vi "MC_8_27_12d_JW.vi"() -> ()   [LabVIEW 2011]
uses:
  <vilib>/Utility/file.llb/Read From Spreadsheet File (string).vi
  <vilib>/Utility/inputDevices.llb/keyboardAcquire.vi
  <vilib>/Utility/file.llb/Write To Spreadsheet File (DBL).vi
  <vilib>/Utility/file.llb/Write To Spreadsheet File (string).vi
  <vilib>/regexp/Match Regular Expression.xnode
panel:
  in  "default (0 dbl) 6":ext format="%.2e"
  in  "default (0 dbl) 5":ext format="%.2e"
  in  "default (0 dbl) 4":ext format="%.2e"
  in  "default (0 dbl) 3":ext format="%.2e"
  in  "default (0 dbl)":ext format="%.2e"
  out "X Axis Display Type":string
  out "Opj X Axis":string
  in  "Room Temp":dbl=294.0
  out "No Image 2":path=path "\\\\acad1\\physics/Jurchescu-group/JW-PD/Image Not Found.png"
  out "Save1 Array":string[][](array[string])
  out "Lin Vd":dbl
  out "Lin-Vg Array-Used":dbl[](array[numeric])
  out "Lin Id-Used":dbl[](array[numeric])
  out "Rec: Comments":string
  out "Folder Index":dbl caption="Length"
  out "Current \nRecord":string[](array[string])
  out "Transformer \nHeaders":string[](array[string])
  out "Current Device ID":string
  out "Column":string
  out "Row":string
  out "Rec: Concentration":dbl
  out "Rec: Solvent":string
  out "Rec: Method":string
  in  "?":T1(tab)
  in  "Transport File":path
  out "Transport Folder":path
  out "Rec: Material":string
  out "Accel (RPM/s):":dbl
  in  "Transfer File":path
  out "Transfer Folder":path
  in  "Image Folder":path
  out "Image File":path=path "D:/UserData/Desktop/Jeremy/WFU/Research/Programs/VI mods/Image Not Found.png"
  in  "Manual Comments":bool
  in  "Comments:":string
  out "Calc: On/Off":dbl caption="On/Off-Sat" format="%#.2e"
  out "Calc: Off I-Sat":dbl caption="Off I-Sat" format="%#.2e"
  in  "Manuel-Dielectric":bool
  in  "Manuel-Length":bool
  out "Calc: VT-Lin":dbl
  out "New: VT-Lin":dbl
  out "Rec: VT-Lin":dbl caption="VT-Lin" format="%#_3g"
  out "Calc: Trap Density-STS":dbl format="%#.2e"
  out "New: Trap Density-STS":dbl format="%#.2e"
  out "Rec: Trap Density-STS":dbl caption="N-Sat (STS)" format="%#.2e"
  out "Calc: Trap Density-VT":dbl format="%#.2e"
  out "New: Trap Density-VT":dbl format="%#.2e"
  out "Rec: Trap Density-VT":dbl caption="N-Sat (VT)" format="%#.2e"
  out "Calc: Mobility-Lin":dbl format="%#.2e"
  out "New: Mobility-Lin":dbl format="%#_4e"
  out "Rec: Mobility-Lin":dbl caption="Mobility-Lin" format="%#_3e"
  out "Calc: Mobility-Sat":dbl format="%#.2e"
  out "Rec: Length":dbl caption="Length" format="%#_3g"
  out "Rec: Width":dbl caption="Width" format="%#_4g"
  out "Rec: Dielectric (d)":dbl caption="Dielectric (d)" format="%#_3g"
  in  "Cancel Button":bool
  in  "Up Button":bool
  in  "Down Button":bool
  out "Data Name:":string
  in  "Save Changes?":bool
  in  "New: Dielectric":dbl
  in  "New: Length":dbl
  in  "New: Width":dbl
  out "New: Mobility-Sat":dbl format="%#.2e"
  in  "Blank Button":bool
  in  "Zoom":i16(slide)=-3 scale=-5.0..5.0
  out "Image Out 2":T2(plugin-control)
  out "Image Out":T2(plugin-control)
  in  "Magnification":u16(ring) items=["5x", "10x", "20x", "50x", "80x"]
  out "Total Width":dbl
  out "Distances":dbl[](array[numeric])
  in  "Undo Button":bool
  in  "Remove Button":bool
  out "Rec: Mobility-Sat":dbl caption="Mobility-Sat" format="%#.2e"
  in  "Export":bool
  out "Calc: VT-Sat":dbl format="%#.2g"
  out "New: VT-Sat":dbl format="%#.2g"
  in  "Manual-Width":bool caption="Manual"
  out "Calc: STS":dbl format="%#.2g"
  out "New: STS":dbl format="%#.2g"
  out "Rec: VT-Sat":dbl caption="VT-Sat" format="%#.2g"
  out "Rec: STS":dbl caption="STS-Sat" format="%#.2g"
  out "Rec: On/Off":dbl caption="On/Off-Sat" format="%#.2e"
  in  "Save Changes? 2":bool
  in  "Save Changes? 3":bool
  out "Rec: Temp":dbl caption="Sample Temp" format="%.1f"
  in  "New: Temp":dbl format="%.1f"
  out "Rec: Off I-Sat":dbl caption="Off I-Sat" format="%#.2e"
  in  "Independant Variable":string(combo)="Length (um):"
  in  "Transfer Plots":T3(tab)=enum."Saturation"
  in  "Lin-Trans Slider":dbl(slide) step=1.0 scale=-22.0..89.0 scale format="%#_1p"
  out "Sqrt-Lin":cluster{dbl[], dbl[]}[](graph)
  in  "Next Sqrt Lin":bool
  in  "Previous Sqrt Lin":bool
  in  "Sat-Trans Slider":dbl(slide) step=1.0 scale=-22.0..89.0 scale format="%#_1p"
  out "Sqrt-Sat":cluster{dbl[], dbl[]}[](graph)
  in  "Previous Sqrt Sat":bool
  in  "Next Sqrt Sat":bool
  out "Raw- Lin":cluster{dbl[], dbl[]}[](graph)
  out "Raw- Sat":cluster{dbl[], dbl[]}[](graph)
  in  "Log Plots":enum32{"Linear", "Saturation", "Transport"}(tab)=enum."Saturation"
  in  "Lin-Log Slider":dbl(slide) step=1.0 scale=-1.0..82.0 scale format="%#_1p"
  in  "Previous Log Lin":bool
  in  "Next Log Lin":bool
  out "Log-Lin":cluster{dbl[], dbl[]}[](graph)
  in  "Sat-Log Slider":dbl(slide) step=1.0 scale=-1.0..82.0 scale format="%#_1p"
  in  "Previous Log Sat":bool
  in  "Next Log Sat":bool
  out "Sat-Log":cluster{dbl[], dbl[]}[](graph)
  out "Transport":cluster{dbl[], dbl[]}[](graph)
  in  "Manual-Temp":bool caption="Manual"
  out "Date Created":string caption="Fabricated"
  out "Date Recorded":string="Date Recorded" caption="Measured"
  out "Image Name":string
  out "Index":string
  in  "Num Pts":dbl=5.0
  in  "NumPoints Log":dbl=5.0 caption="Num Pts"
  in  "Ring":u16(ring) items=["Extra Small", "Small", "Medium", "Large", "Extra Large"]
  in  "Transport Line Color":u32(colorbox)
  in  "Origin Project File":path=path "\\\\acad1\\physics/Jurchescu-group/JW-PD/Group Library/Origin Project Files/DeviceData_8_10_12a_JW.opj"
  in  "No Image File":path=path "\\\\acad1\\physics/Jurchescu-group/JW-PD/Mega Awesome/Image Not Found.png"
  in  "Ramp (s):":dbl=3.0
  in  "Fabricator:":string="NaN"
  in  "Sample #:":dbl=1.0
  in  "Wait Time (s):":dbl=nan
  in  "RPM:":dbl=nan
  in  "Time (s):":dbl=nan
  in  "Room Temp (F):":dbl=nan
  in  "Relative Humidity (%):":dbl=nan
  in  "Solution Temp (C):":dbl=nan
  in  "# Drops*:":dbl=inf
  in  "Surface Treatment:":string="NaN"
  in  "Treatment Concentration (mM):":dbl=nan
  out "String":string
  out "Index 2":dbl
  out "Sat Id-Log-Used":dbl[](array[numeric])
  out "Vg Array-Log-Used":dbl[](array[numeric])
  out "ROI Descriptor out":T4 {"Contours"."Type" items=["No Selection", "Point", "Line", "Rectangle", "Oval", "Polygon", "Freehand Region", "Annulus", "Unused2", "Unused3", "Broken Line", "Freehand Line", "Rotated Rectangle"]}
  out "ROI Descriptor":T4 {"Contours"."Type" items=["No Selection", "Point", "Line", "Rectangle", "Oval", "Polygon", "Freehand Region", "Annulus", "Unused2", "Unused3", "Broken Line", "Freehand Line", "Rotated Rectangle"]}
  out "Numeric 3":dbl
  out "Array 6":dbl[][](array[numeric])
  out "Cluster":T5
  out "Array 5":dbl[](array[numeric])
  out "Array 4":dbl[](array[numeric])
  out "Array 3":dbl[](array[numeric])
  out "Numeric 2":dbl
  out "Numeric":dbl
  out "Sat Id-Used":dbl[](array[numeric])
  out "Sat Vg Array-Used":dbl[](array[numeric])
  out "MobVi Index":dbl
  in  "Row Start":dbl=20.0
  # "Data Locations"
  # "Transfer Location"
  # "Image Location"
  # "Recorded"
  # "Calculated"
  # "Re-Calculated"
  # "Manual"
  # "Used points display at y=0"
  # "Slider\nDoesn't\nWork"
  # "Slider\nDoesn't\nWork"
  # "No new points displayed"
  # "Sample Properties"
  # "*     Inf = Full coverage\n   NaN = Unknown or Not Applicable"
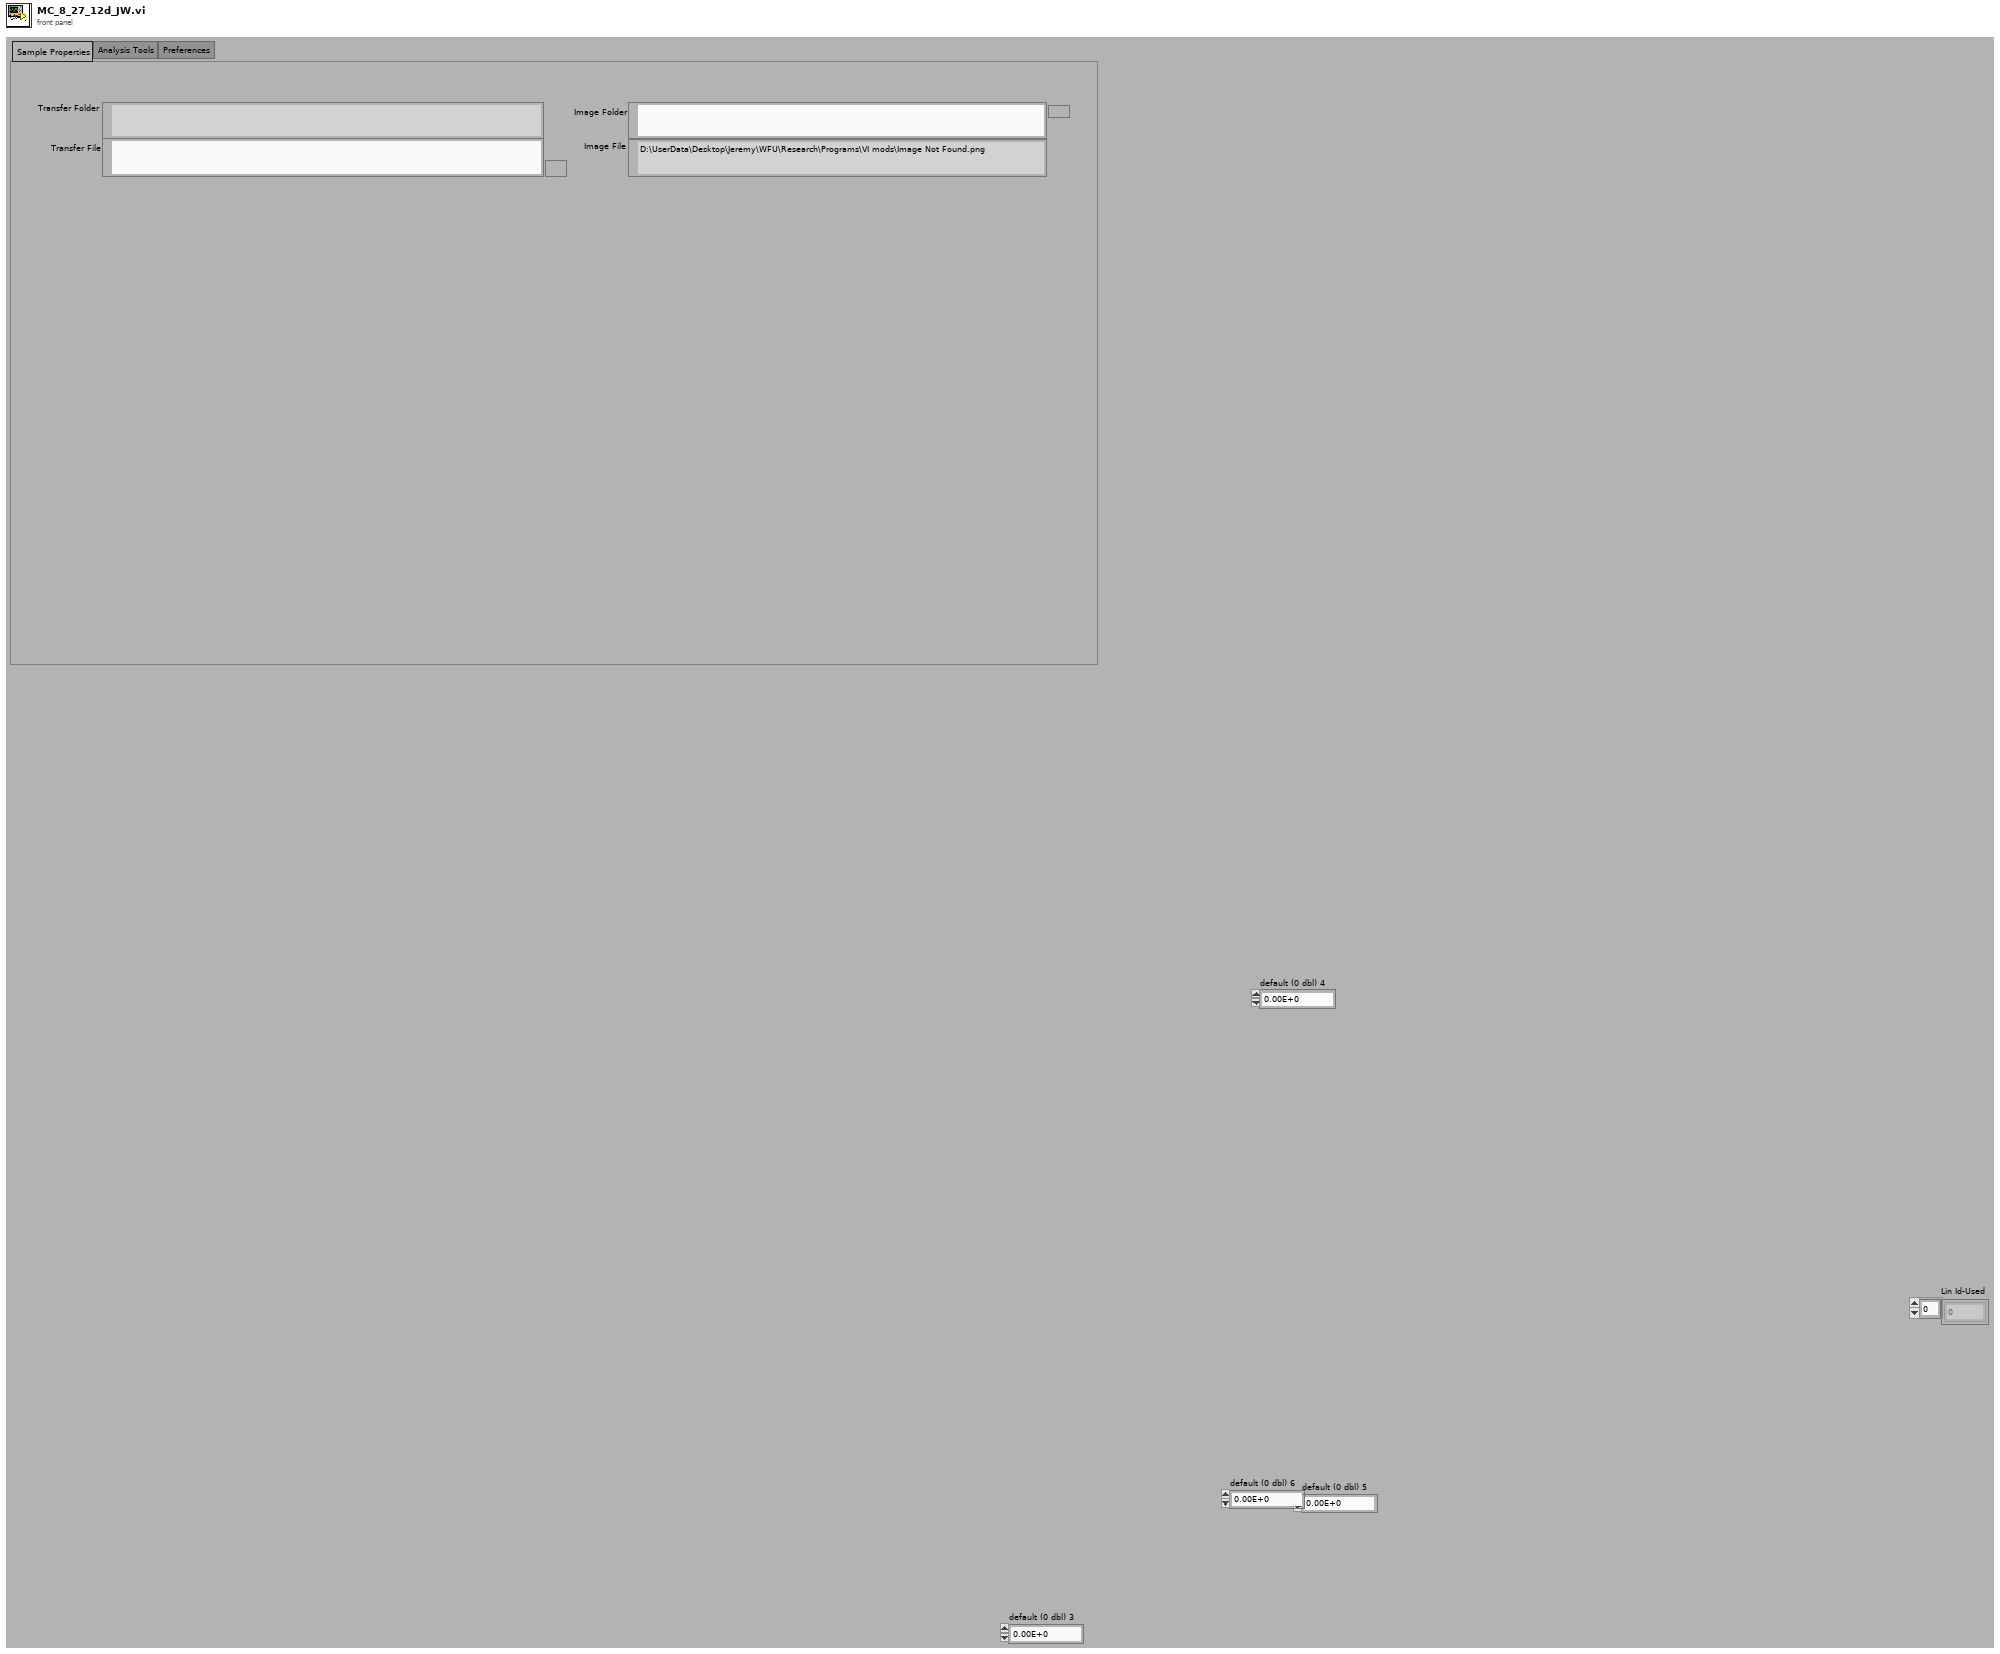
[diagram p1: front panel]
types:
  T1 = enum32{"Sample Properties", "Analysis Tools", "Preferences", "Current Database"}
  T2 = typedef "IMAQ Image.ctl" = refnum<image>
  T3 = enum32{"Linear", "Saturation", "Raw-Linear", "Raw-Saturation"}
  T4 = typedef "ROI Descriptor" = cluster{"Global Rectangle":i32[], "Contours":cluster{"ID":enum32{"External", "Internal"}, "Type":u32, "Coordinates":i32[]}[]}
  T5 = cluster{"Numeric":dbl, "Numeric 2":dbl, "Numeric 3":dbl, "Numeric 4":dbl}
  T6 = cluster{"Mobility-Sat":dbl, "Moblitity-Lin":dbl, "On/Off":dbl, "Off Current":dbl, "Vt-Sat":dbl, "STS":dbl, "Trap Density-VT":dbl, "Trap Density-STS":dbl}
  T7 = cluster{"Date Recorded":string, "Index":string, "Length":dbl, "Width":dbl, "Sample Temp":dbl}
  T8 = cluster{"Date Created":string, "Material":string, "Solvent":string, "Concentration":dbl, "Method":string, "Dielectric (nm)":dbl, "Treatment":string, "Comments":string}
  T9 = cluster{"Raw Sat":cluster{dbl[], dbl[]}[], "Sqrt Sat":cluster{dbl[], dbl[]}[], "Log Sat":cluster{dbl[], dbl[]}[], "Raw Lin":cluster{dbl[], dbl[]}[], "Sqrt Lin":cluster{dbl[], dbl[]}[], "Log Lin":cluster{dbl[], dbl[]}[]}
  T10 = cluster{"Mobility-Sat":dbl, "Vt-Sat":dbl, "Mobility-Lin":dbl, "Vt-Lin":dbl, "Off I-Sat":dbl, "On/Off I-Sat":dbl}
  T11 = cluster{"[0]":cluster{dbl[], dbl[]}, "[1]":cluster{dbl[], dbl[]}, "[2]":cluster{dbl[], dbl[]}, "[3]":cluster{dbl[], dbl[]}, "[4]":cluster{dbl[], dbl[]}, "[5]":cluster{dbl[], dbl[]}, "[6]":cluster{dbl[], dbl[]}, "[7]":cluster{dbl[], dbl[]}, "[8]":cluster{dbl[], dbl[]}}
  T12 = cluster{"Global Rectangle":i32[], "Contours":cluster{"Contour Type":u32, "ROI Type":u32, "Points":i32[]}[]}
  T13 = typedef "LVBoundsTypeDef.ctl" = cluster{"Width":u32, "Height":u32}
  T14 = enum16{"0", "1", "2", "3", "4", "5", "6", "7", "8", "9", "A", "B", "C", "D", "E", "F", "G", "H", "I", "J", "K", "L", "M", "N", "O", "P", "Q", "R", "S", "T", "U", "V", "W", "X", "Y", "Z", "F1", "F2", "F3", "F4", "F5", "F6", "F7", "F8", "F9", "F10", "F11", "F12", "F13", "F14", "F15", "ADD", "BACK", "BACKSLASH", "CAPITAL", "COMMA", "DECIMAL", "DELETE", "DIVIDE", "DOWN", "END", "EQUALS", "ESCAPE", "GRAVE (`)", "HOME", "INSERT", "LBRACKET", "LCONTROL", "LEFT", "L ALT", "LSHIFT", "LWIN", "MINUS", "MULTIPLY", "NEXT", "NUMLOCK", "NUMPAD_0", "NUMPAD_1", "NUMPAD_2", "NUMPAD_3", "NUMPAD_4", "NUMPAD_5", "NUMPAD_6", "NUMPAD_7", "NUMPAD_8", "NUMPAD_9", "PAUSE", "PERIOD", "PRIOR (PG UP)", "RBRACKET", "RCONTROL", "RETURN", "RIGHT", "R ALT", "RSHIFT", "RWIN", "SCROLL", "SEMICOLON", "SLASH", "SPACE", "SUBTRACT", "TAB", "UP", "ENTER (num pad)", "' (quote)"}[]
  T15 = enum16{"0", "1", "2", "3", "4", "5", "6", "7", "8", "9", "A", "B", "C", "D", "E", "F", "G", "H", "I", "J", "K", "L", "M", "N", "O", "P", "Q", "R", "S", "T", "U", "V", "W", "X", "Y", "Z", "F1", "F2", "F3", "F4", "F5", "F6", "F7", "F8", "F9", "F10", "F11", "F12", "F13", "F14", "F15", "ADD", "BACK", "BACKSLASH", "CAPITAL", "COMMA", "DECIMAL", "DELETE", "DIVIDE", "DOWN", "END", "EQUALS", "ESCAPE", "GRAVE (`)", "HOME", "INSERT", "LBRACKET", "LCONTROL", "LEFT", "L ALT", "LSHIFT", "LWIN", "MINUS", "MULTIPLY", "NEXT", "NUMLOCK", "NUMPAD_0", "NUMPAD_1", "NUMPAD_2", "NUMPAD_3", "NUMPAD_4", "NUMPAD_5", "NUMPAD_6", "NUMPAD_7", "NUMPAD_8", "NUMPAD_9", "PAUSE", "PERIOD", "PRIOR (PG UP)", "RBRACKET", "RCONTROL", "RETURN", "RIGHT", "R ALT", "RSHIFT", "RWIN", "SCROLL", "SEMICOLON", "SLASH", "SPACE", "SUBTRACT", "TAB", "UP", "ENTER (num pad)", "' (quote)"}
  T16 = cluster{"Contour Type":u32, "ROI Type":u32, "Points":i32[]}[]
  T17 = cluster{i32[], cluster{"Contour Type":u32, "ROI Type":u32, "Points":i32[]}[]}
  T18 = cluster{"Independant  Variable Indicator":string, "Parameter String Indicator":string}
  T19 = cluster{string, sgl, bool, bool, bool, bool, bool, bool, i32}
  T20 = cluster{i32, cluster{string, sgl, bool, bool, bool, bool, bool, bool, i32}, i32, i32}
  T21 = cluster{"Contour Type":u32, "ROI Type":u32, "Points":i32[]}
  T22 = cluster{"Points[0]":i32, "Points[1]":i32, "Points[2]":i32, "Points[3]":i32, "Points[4]":i32, "Points[5]":i32, "Points[6]":i32, "Points[7]":i32, "Points[8]":i32}
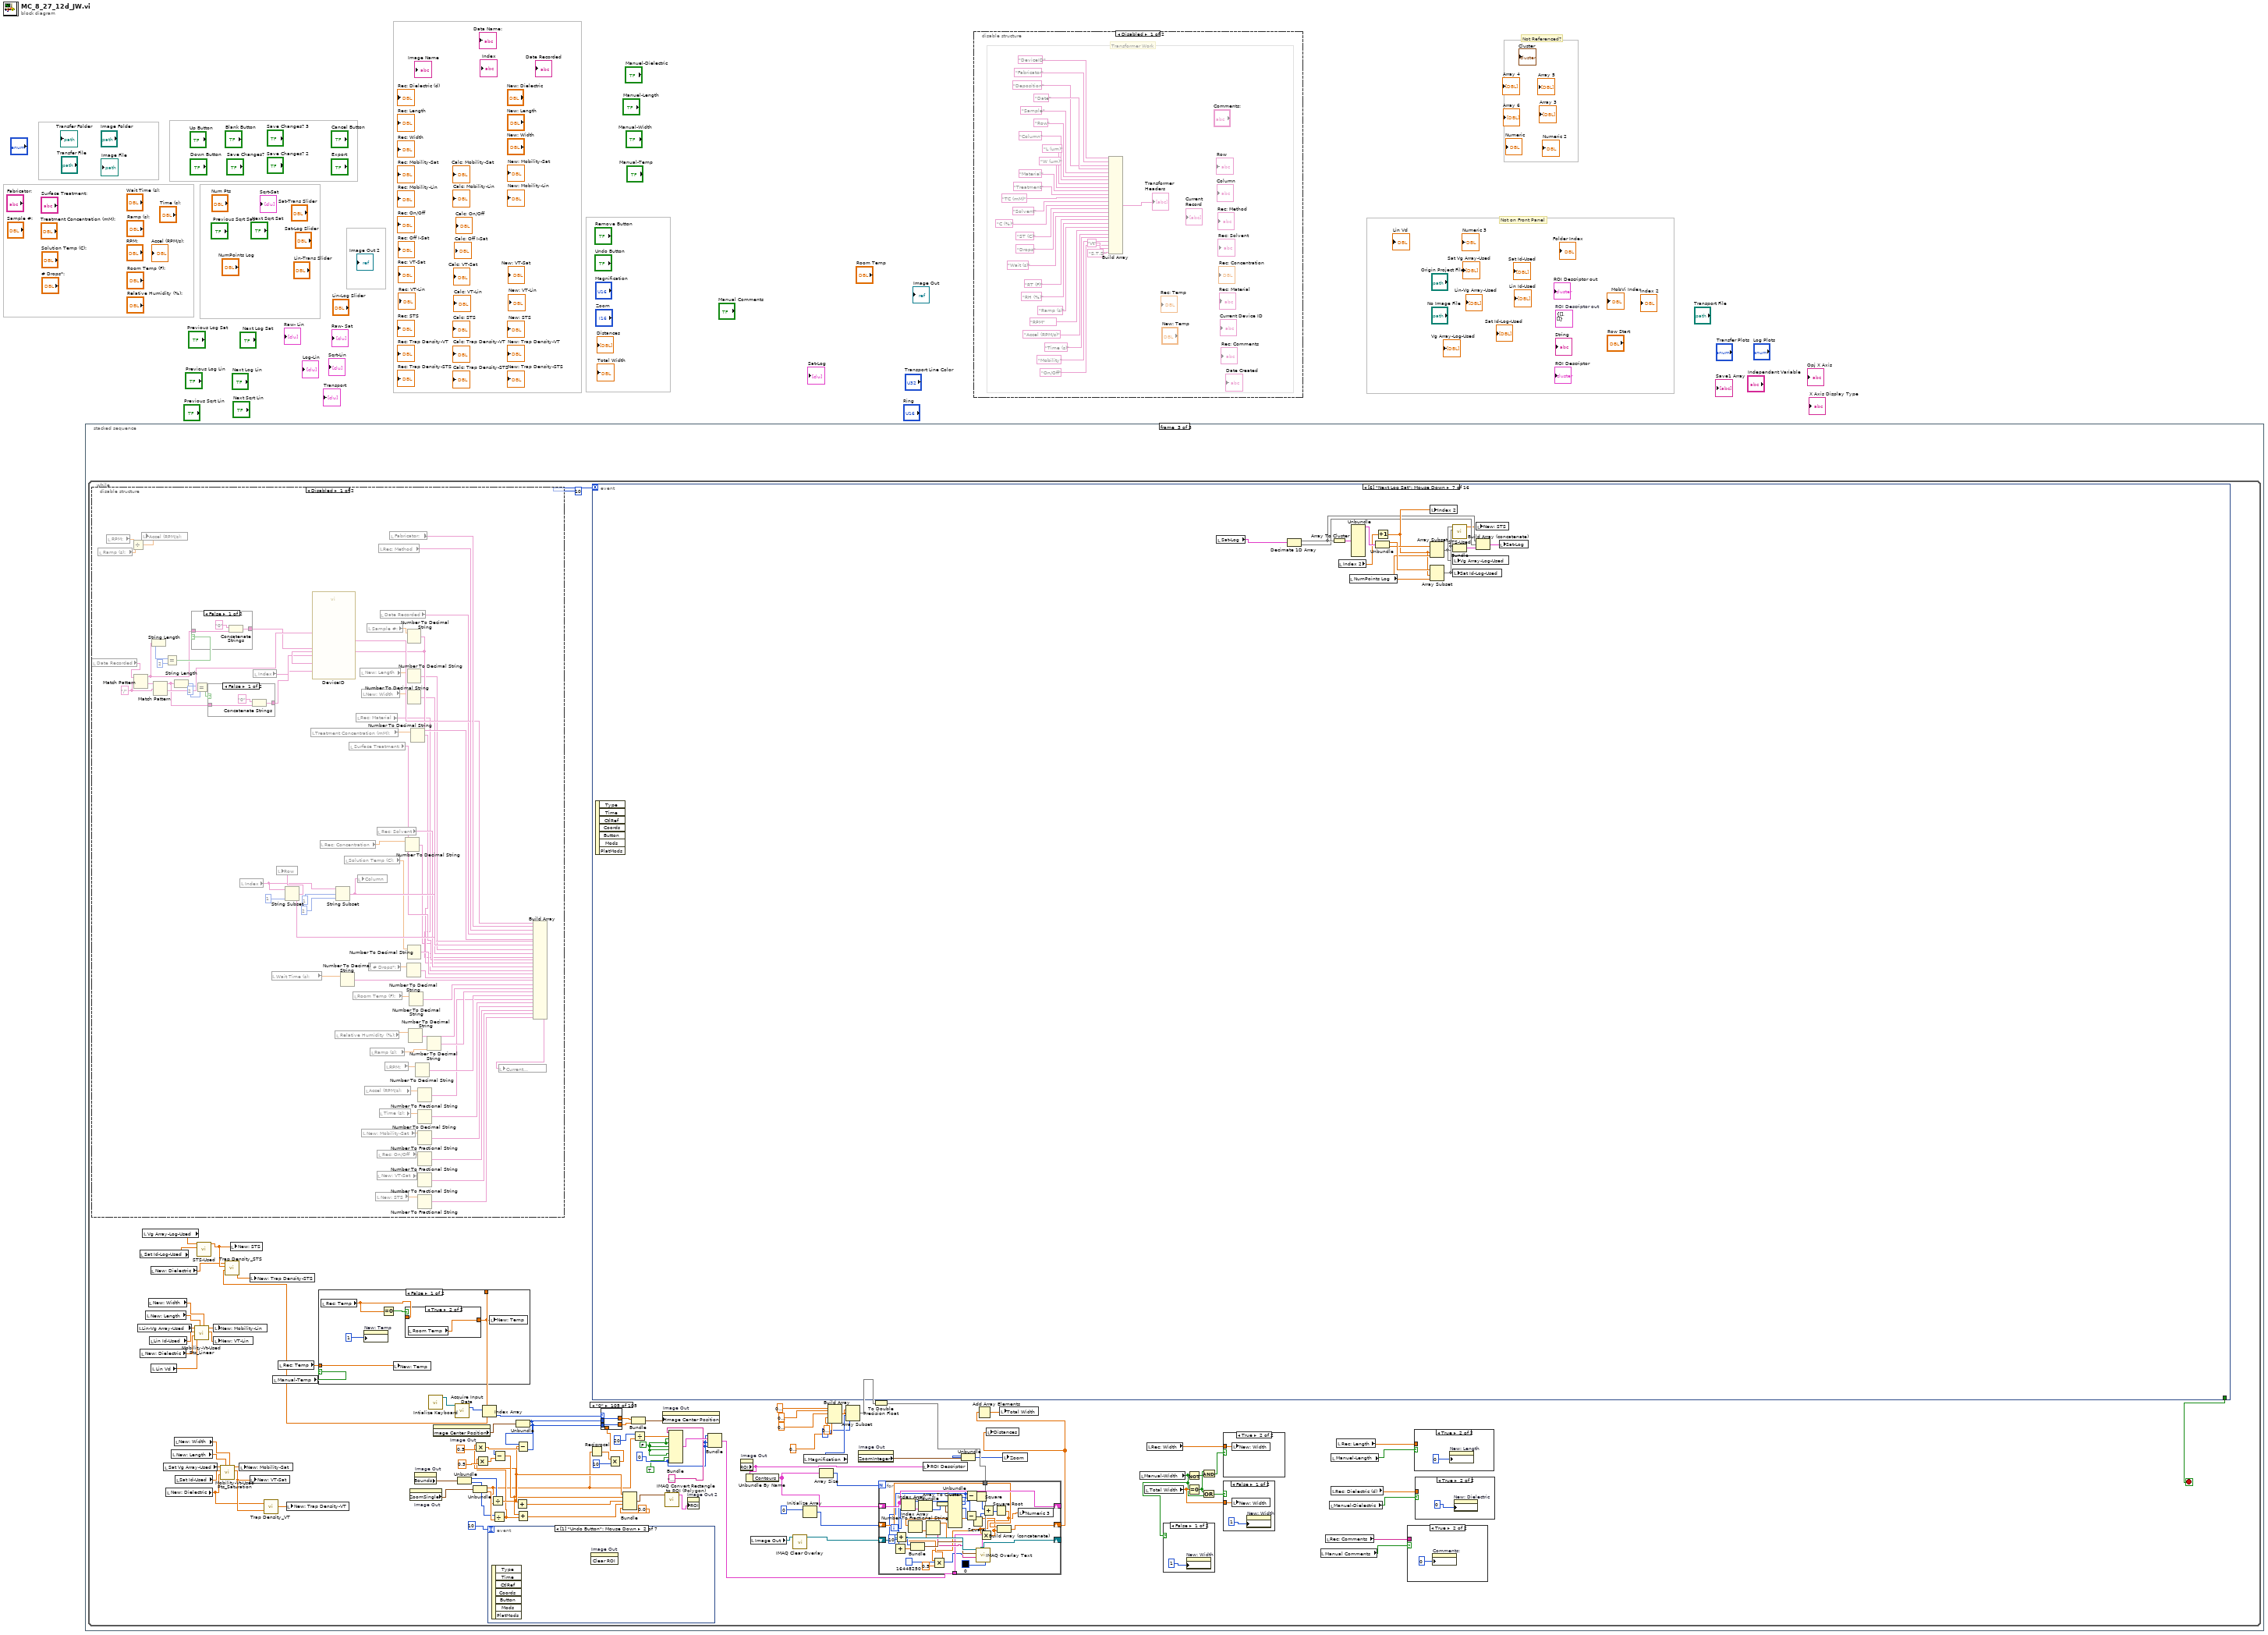
[diagram p0: block diagram]
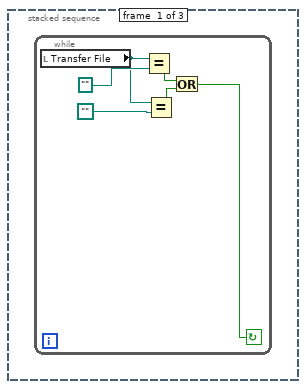
[diagram p3: hidden frame]
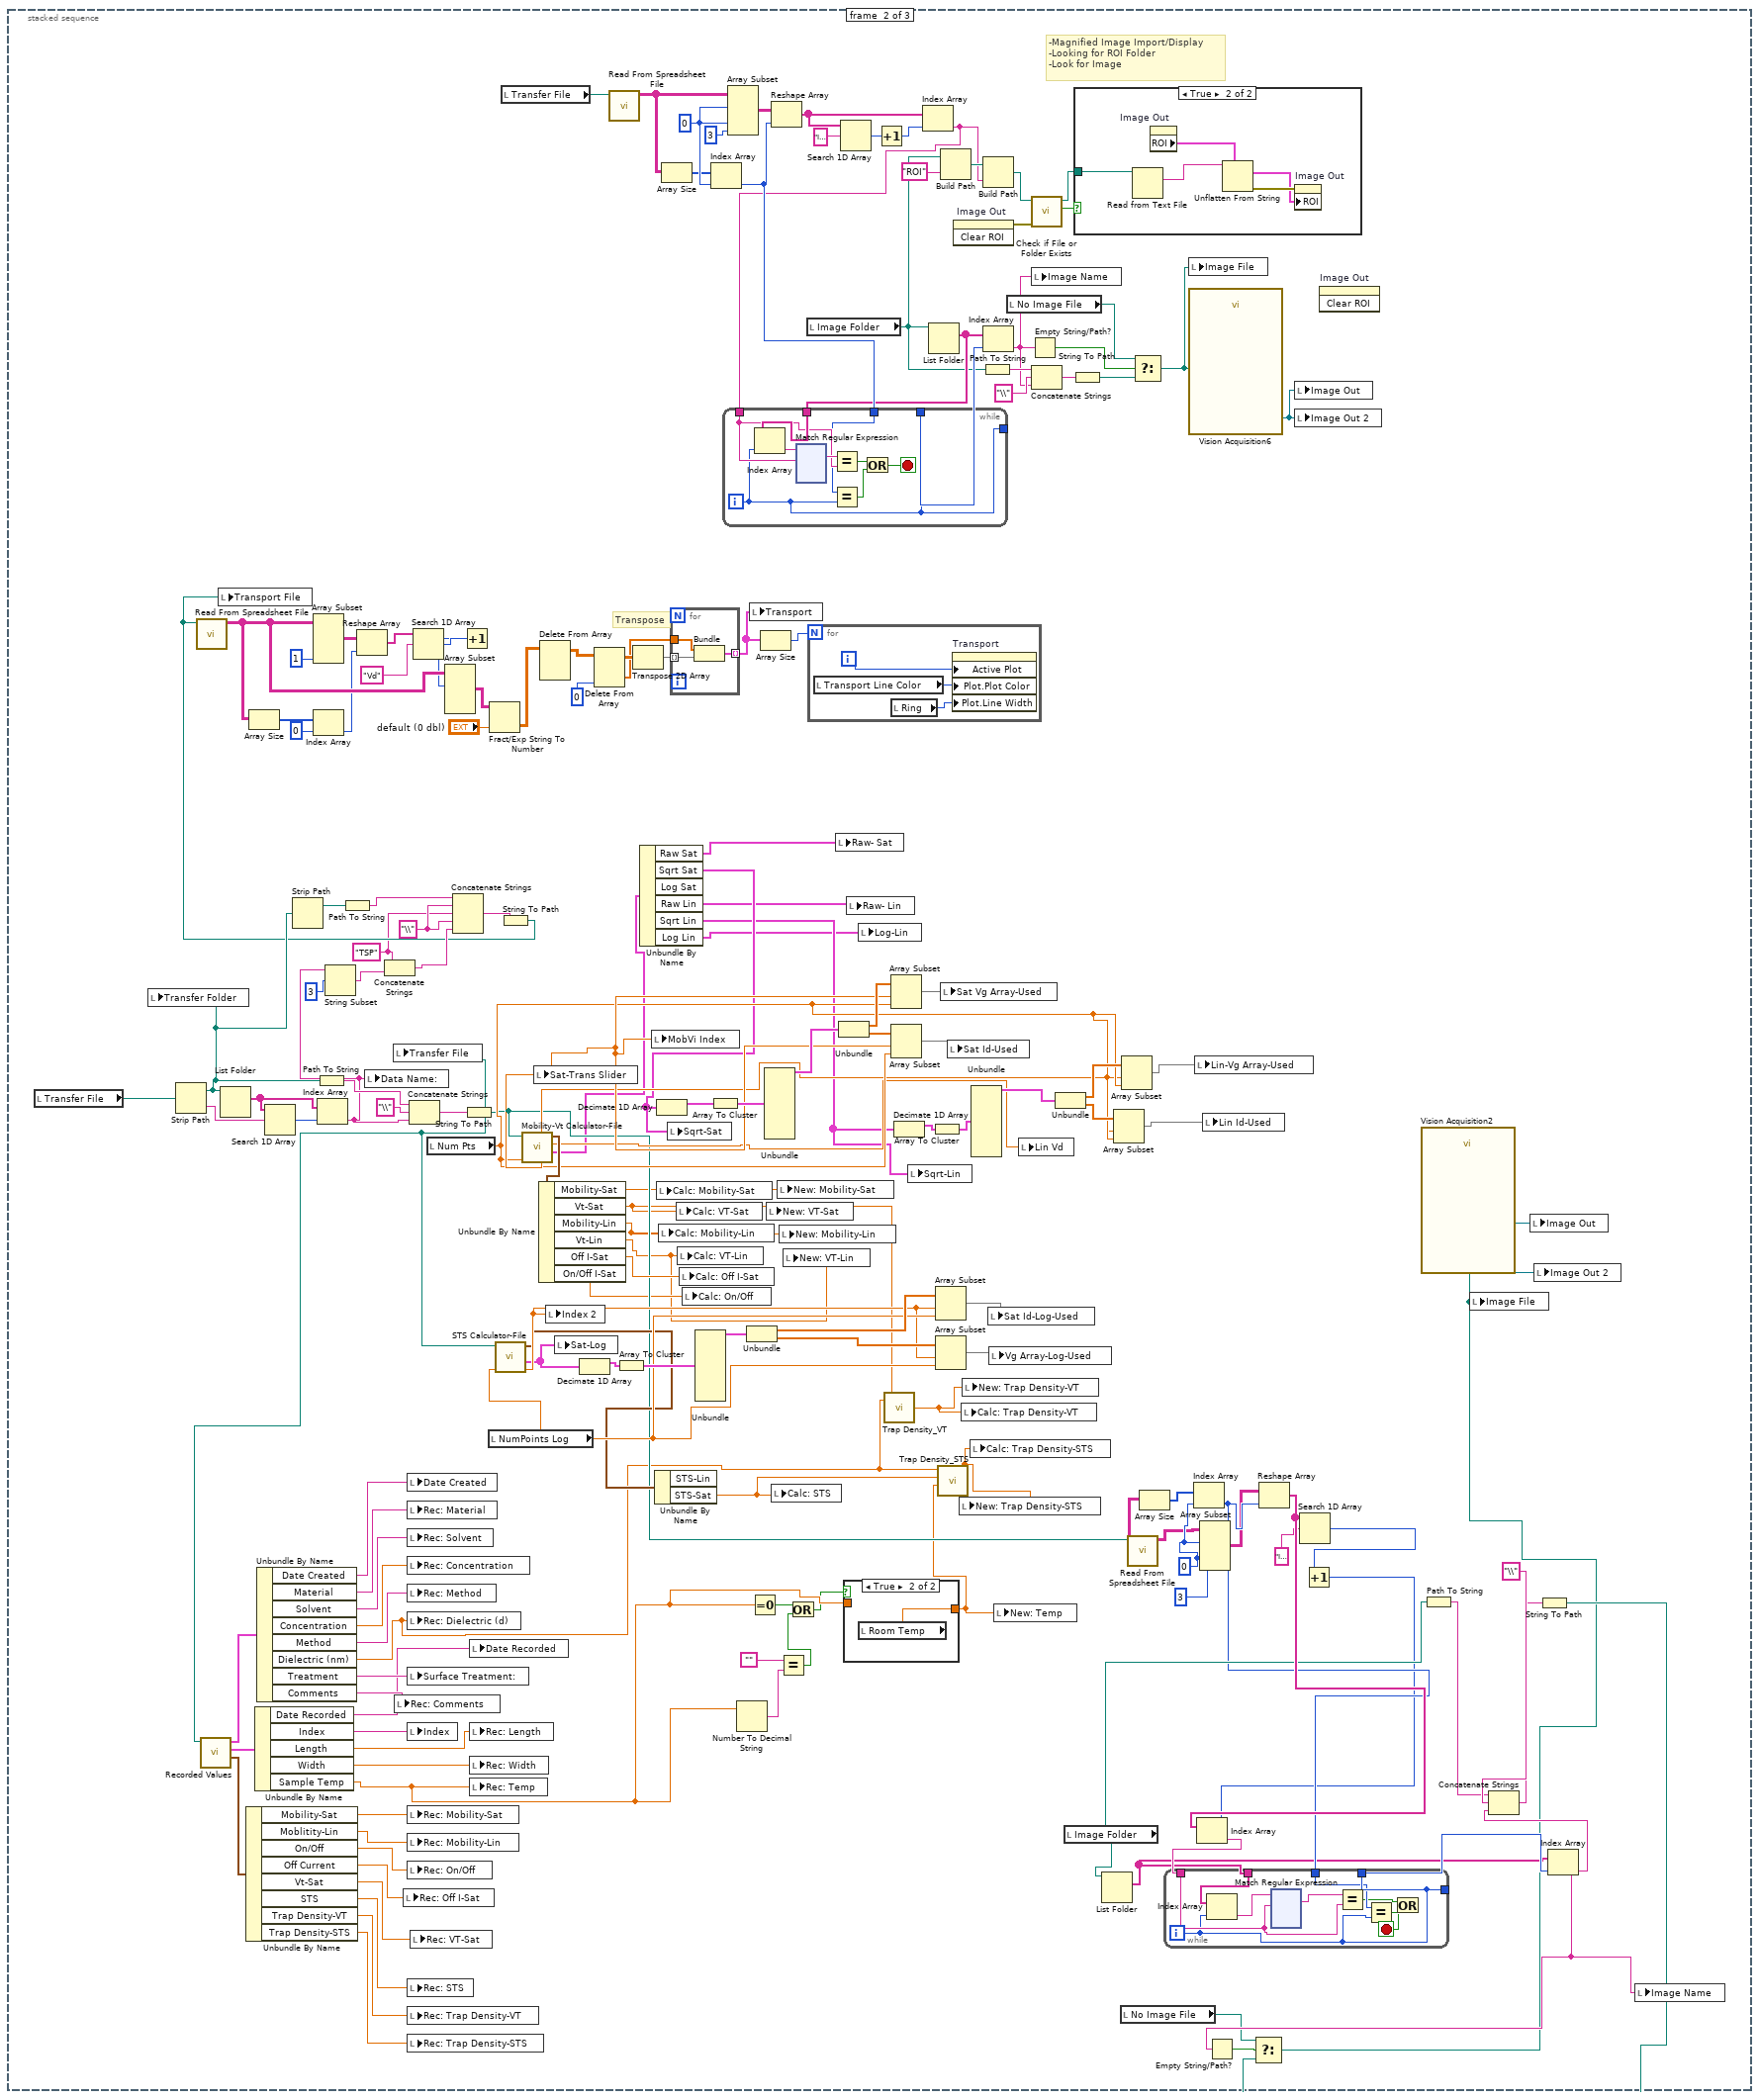
[diagram p4: hidden frame]
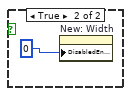
[diagram p10: hidden frame]
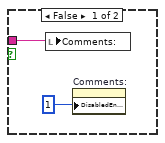
[diagram p11: hidden frame]
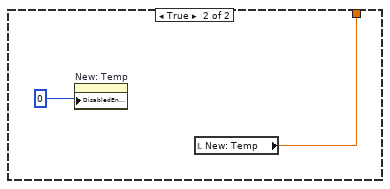
[diagram p13: hidden frame]
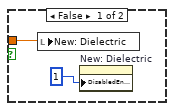
[diagram p14: hidden frame]
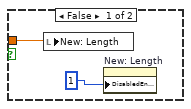
[diagram p15: hidden frame]
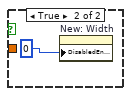
[diagram p17: hidden frame]
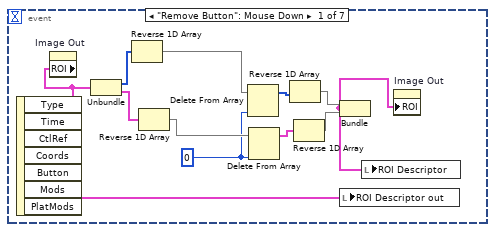
[diagram p18: hidden frame]
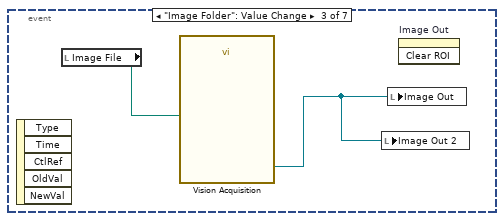
[diagram p19: hidden frame]
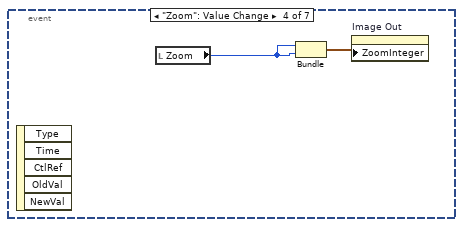
[diagram p20: hidden frame]
diagram:
  (unwired) T4 {"Global Rectangle"=[], "Contours"=[]}  # ROI Descriptor out
  # "Not Referenced?"
  # "Not on Front Panel"
  n1 = stacked-sequence {
    frame #0 {
      n2 = while {
        stop <- w1 continue-if-true
        n3 = local read "Transfer File"() -> (w3:path)
        n4 = Equal?(x=w3, y=path "") -> (x = y?=w5:bool)
        n5 = Equal?(x=w3, y=path "") -> (x = y?=w4:bool)
        n6 = Or(x=w5, y=w4) -> (x .or. y?=w1:bool)
      }
    }
    frame #1 {
      w9 = "\\"
      w8 = "TSP"
      w139 = 0
      w162 = 0
      # "Transpose"
      # "-Magnified Image Import/Display\n-Looking for ROI Folder\n-Look for Image"
      n7 = local read "Transfer File"() -> (w143:path)
      n8 = Strip Path(path=w143) -> (stripped path=w18:path, name=w130:string)
      n9 = local write "Transfer Folder"(w18) -> ()
      n10 = List Folder(path=w18) -> (filenames=w134:string[])  [unwired: 3 in, 3 out]
      n11 = Search 1D Array(1D array=w134, element=w130) -> (index of element=w133:i32)  [unwired: 1 in]
      n12 = Strip Path(path=w18) -> (stripped path=w14:path)  [unwired: 1 out]
      n13 = Path To String(path=w18) -> (string=w129:string)
      n14 = Index Array(array=w134, index=w133) -> (element=w17:string)
      n15 = String Subset(string=w17, offset (0)=3) -> (substring=w15:string)  [unwired: 1 in]
      n16 = Path To String(path=w14) -> (string=w10:string)
      n17 = local write "Data Name:"(w17) -> ()
      n18 = Concatenate Strings(w8, w15) -> (w13:string)
      n19 = Concatenate Strings(w129, "\\", w17) -> (w131:string)
      n20 = local read "Num Pts"() -> (w68:dbl)
      n21 = Concatenate Strings(w10, w9, w8, w9, w13) -> (w12:string)
      n22 = String To Path(string=w131) -> (path=w62:path)
      n23 = call "Recorded Values.vi"("Path"=w62) -> ("Recorded Char"=w98:T6, "Recorded Prop"=w97:T7, "Fabrication Prop"=w99:T8)  [unwired: 8 in]
      n24 = Unbundle By Name(w98) -> ("Mobility-Sat"=w86:dbl, "Moblitity-Lin"=w85:dbl, "On/Off"=w84:dbl, "Off Current"=w83:dbl, "Vt-Sat"=w48:dbl, "STS"=w82:dbl, "Trap Density-VT"=w81:dbl, "Trap Density-STS"=w80:dbl)
      n25 = Unbundle By Name(w97) -> ("Date Recorded"=w90:string, "Index"=w89:string, "Length"=w88:dbl, "Width"=w87:dbl, "Sample Temp"=w54:dbl)
      n26 = Unbundle By Name(w99) -> ("Date Created"=w79:string, "Material"=w96:string, "Solvent"=w95:string, "Concentration"=w94:dbl, "Method"=w93:string, "Dielectric (nm)"=w58:dbl, "Treatment"=w92:string, "Comments"=w91:string)
      n27 = local write "Transfer File"(w62) -> ()
      n28 = local write "Rec: Comments"(w91) -> ()
      n29 = local write "Rec: Off I-Sat"(w83) -> ()
      n30 = local write "Date Created"(w79) -> ()
      n31 = local write "Rec: Material"(w96) -> ()
      n32 = local write "Rec: Solvent"(w95) -> ()
      n33 = local write "Rec: Concentration"(w94) -> ()
      n34 = local write "Rec: Method"(w93) -> ()
      n35 = local write "Rec: Dielectric (d)"(w58) -> ()
      n36 = local write "Surface Treatment:"(w92) -> ()
      n37 = local write "Index"(w89) -> ()
      n38 = local write "Rec: Mobility-Sat"(w86) -> ()
      n39 = local write "Rec: Mobility-Lin"(w85) -> ()
      n40 = local write "Rec: On/Off"(w84) -> ()
      n41 = local write "Rec: STS"(w82) -> ()
      n42 = local write "Rec: Trap Density-VT"(w81) -> ()
      n43 = local write "Rec: Trap Density-STS"(w80) -> ()
      n44 = local write "Rec: VT-Sat"(w48) -> ()
      n45 = local write "Date Recorded"(w90) -> ()
      n46 = local write "Rec: Length"(w88) -> ()
      n47 = local write "Rec: Width"(w87) -> ()
      n48 = local write "Rec: Temp"(w54) -> ()
      n49 = local read "NumPoints Log"() -> (w76:dbl)
      n50 = call "STS Calculator-File.vi"("NumPts"=w76, "Path"=w62) -> ("STS Index-Sat"=w75:dbl, "XY Graph-Sat"=w7:cluster{dbl[], dbl[]}[], "Ouput"=w74:cluster{"STS-Sat":dbl, "STS-Lin":dbl})  [unwired: 5 in, 2 out]
      n51 = String To Path(string=w12) -> (path=w11:path)
      n52 = call-poly <vilib>:"Read From Spreadsheet File.vi"("file path (dialog if empty)"=w11) -> ("all rows"=w32:string[][])  [unwired: 6 in, 4 out]
      n53 = local write "Transport File"(w11) -> ()
      n54 = Array Size(array=w32) -> (size(s)=w38:i32[])
      n55 = Array Subset(array=w32, length (col)=1) -> (w34:string[][])  [unwired: 3 in]
      n56 = Index Array(array=w38, index=0) -> (element=w27:i32)
      n57 = Reshape Array(w34, w27) -> (w33:string[])
      n58 = Search 1D Array(1D array=w33, element="Vd") -> (index of element=w31:i32)  [unwired: 1 in]
      n59 = Increment(x=w31) -> (x+1=w30:i32)
      n60 = Array Subset(array=w32, index (row)=w30) -> (w28:string[][])  [unwired: 3 in]
      n61 = Fract/Exp String To Number(string=w28, default (0 dbl)="default (0 dbl)") -> (number=w20:ext[][])  [unwired: 2 in, 1 out]
      n62 = local read "Transfer File"() -> (w157:path)
      n63 = call "Mobility-Vt Calculator-File.vi"("NumPts"=w68, "Path"=w62) -> ("Graph Cluster"=w39:T9, "Lin Vd"=w64:dbl, "Output"=w78:T10, "Index-Sat"=w77:dbl, "Index-Lin"=w67:dbl)  [unwired: 5 in]
      n64 = local write "Sat-Trans Slider"(w77) -> ()
      n65 = Unbundle By Name(w78) -> ("Mobility-Sat"=w57:dbl, "Vt-Sat"=w56:dbl, "Mobility-Lin"=w47:dbl, "Vt-Lin"=w45:dbl, "Off I-Sat"=w63:dbl, "On/Off I-Sat"=w46:dbl)
      n66 = Delete From Array(array=w20) -> (array with subset deleted=w19:ext[][])  [unwired: 3 in, 1 out]
      n67 = local write "Index 2"(w75) -> ()
      n68 = local write "Sat-Log"(w7) -> ()
      n69 = Decimate 1D Array(w7) -> (w121:cluster{dbl[], dbl[]}[])  [unwired: 1 out]
      n70 = Delete From Array(array=w19, index (col)=0 ("Deaktivierter Index (Spalte)")) -> (deleted portion=w24:ext[], array with subset deleted=w25:ext[][])  [unwired: 2 in]
      n71 = call-poly <vilib>:"Read From Spreadsheet File.vi"("file path (dialog if empty)"=w157) -> ("all rows"=w160:string[][])  [unwired: 6 in, 4 out]
      n72 = Array To Cluster(array=w121) -> (cluster=w123:T11)
      n73 = Transpose 2D Array(2D array=w25) -> (transposed array=w26:ext[][])
      n74 = Unbundle By Name(w39) -> ("Raw Sat"=w42:cluster{dbl[], dbl[]}[], "Sqrt Sat"=w44:cluster{dbl[], dbl[]}[], "Raw Lin"=w41:cluster{dbl[], dbl[]}[], "Sqrt Lin"=w43:cluster{dbl[], dbl[]}[], "Log Lin"=w40:cluster{dbl[], dbl[]}[])  [unwired: 1 out]
      n75 = local write "MobVi Index"(w77) -> ()
      n76 = Unbundle By Name(w74) -> ("STS-Sat"=w61:dbl)  [unwired: 1 out]
      n77 = Decimate 1D Array(w44) -> (w156:cluster{dbl[], dbl[]}[])  [unwired: 1 out]
      n78 = local write "Calc: Mobility-Sat"(w57) -> ()
      n79 = local write "Calc: Mobility-Lin"(w47) -> ()
      n80 = Array Size(array=w160) -> (size(s)=w161:i32[])
      n81 = local write "Sqrt-Sat"(w44) -> ()
      n82 = for {
        tunnel: w24 -> [w178]
        tunnel: w26 -> [w179] mode=indexing
        tunnel: [w177] -> w22 mode=indexing
        n83 = Bundle(w178, w179) -> (w177:cluster{ext[], ext[]})  [unwired: 1 in]
      }
      n84 = local write "Calc: VT-Sat"(w56) -> ()
      n85 = local write "Calc: VT-Lin"(w45) -> ()
      n86 = local write "Calc: Off I-Sat"(w63) -> ()
      n87 = local write "Calc: On/Off"(w46) -> ()
      n88 = Unbundle(w123) -> ("[0]"=w122:cluster{dbl[], dbl[]})  [unwired: 8 out]
      n89 = Array To Cluster(array=w156) -> (cluster=w154:T11)
      n90 = Index Array(array=w161, index=w162) -> (element=w168:i32)
      n91 = Array Subset(array=w160, index (row)=w162, index (col)=w162, length (col)=3) -> (w159:string[][])  [unwired: 1 in]
      n92 = Number To Decimal String(number=w54) -> (decimal integer string=w52:string)  [unwired: 1 in]
      n93 = Unbundle(w122) -> (w119:dbl[], w118:dbl[])
      n94 = local write "Transport"(w22) -> ()
      n95 = Equal To 0?(x=w54) -> (x = 0?=w53:bool)
      n96 = Array Size(array=w22) -> (size(s)=w21:i32)
      n97 = Unbundle(w154) -> ("[0]"=w155:cluster{dbl[], dbl[]})  [unwired: 8 out]
      n98 = local write "New: VT-Sat"(w56) -> ()
      n99 = Reshape Array(w159, w168) -> (w173:string[])
      n100 = local write "Calc: STS"(w61) -> ()
      n101 = local write "New: Mobility-Sat"(w57) -> ()
      n102 = Equal?(x="", y=w52) -> (x = y?=w50:bool)
      n103 = local write "New: Mobility-Lin"(w47) -> ()
      n104 = local write "New: VT-Lin"(w45) -> ()
      n105 = Or(x=w53, y=w50) -> (x .or. y?=w49:bool)
      n106 = local read "Image Folder"() -> (w100:path)
      n107 = for {
        N: w21 -> [_]
        i -> [w176]
        n108 = local read "Transport Line Color"() -> (w175:u32)
        n109 = local read "Ring"() -> (w174:u16)
        n110 = property on="Transport" class="XYGraph (strict)"("Active Plot"=w176, "Plot.Plot Color"=w175, "Plot.Line Width"=w174) -> ()  [unwired: 2 in, 2 out]
      }
      n111 = local write "Raw- Sat"(w42) -> ()
      n112 = Unbundle(w155) -> (w120:dbl[], w124:dbl[])
      n113 = Search 1D Array(1D array=w173, element="Index:") -> (index of element=w165:i32)  [unwired: 1 in]
      n114 = case shown="True" w49 {
        tunnel: [w180 w181] -> w60
        tunnel: w54 -> [w180 _]
        frame False {
        }
        frame True {
          n115 = local read "Room Temp"() -> (w181:dbl)
        }
      }
      n116 = local write "Raw- Lin"(w41) -> ()
      n117 = local write "Log-Lin"(w40) -> ()
      n118 = Increment(x=w165) -> (x+1=w164:i32)
      n119 = call "Trap Density_VT.vi"("VT"=w56, "Dielectric"=w58) -> ("Trap Density-VT"=w55:dbl)
      n120 = Array Subset(array=w120, index=w77, length=w68) -> (w127:dbl[])
      n121 = Array Subset(array=w124, index=w77, length=w68) -> (w128:dbl[])
      n122 = Decimate 1D Array(w43) -> (w73:cluster{dbl[], dbl[]}[])  [unwired: 1 out]
      n123 = local write "Sqrt-Lin"(w43) -> ()
      n124 = Index Array(array=w173, index=w164) -> (element=w101:string)
      n125 = List Folder(path=w100) -> (filenames=w166:string[])  [unwired: 3 in, 3 out]
      n126 = while {
        tunnel: w166 -> [w314]
        tunnel: w101 -> [w312]
        tunnel: [w311] -> _
        tunnel: [w311] -> w167
        tunnel: w168 -> [w310]
        i -> [w311]
        stop <- w307 stop-if-true
        n127 = Index Array(array=w314, index=w311) -> (element=w315:string)
        n128 = xnode "Match Regular Expression"("input string"=w315, "regular expression"=w312) -> ("whole match"=w313:string)  [unwired: 4 in, 4 out]
        n129 = Equal?(x=w313, y=w312) -> (x = y?=w309:bool)
        n130 = Equal?(x=w310, y=w311) -> (x = y?=w308:bool)
        n131 = Or(x=w309, y=w308) -> (x .or. y?=w307:bool)
      }
      n132 = Array To Cluster(array=w73) -> (cluster=w72:T11)
      n133 = Array Subset(array=w119, index=w75, length=w76) -> (w126:dbl[])
      n134 = Array Subset(array=w118, index=w75, length=w76) -> (w125:dbl[])
      n135 = call "Trap Density_STS.vi"("Temp (T) [K]"=w60, "S.T.S. (S)"=w61, "Dielectric"=w58) -> ("Trap Density (N)"=w59:dbl)  [unwired: 8 in]
      n136 = Build Path(base path=w100, name or relative path="ROI") -> (appended path=w103:path)
      n137 = local write "Sat Vg Array-Used"(w127) -> ()
      n138 = local write "Sat Id-Used"(w128) -> ()
      n139 = invoke on="Image Out" class="ImageControl" method="Clear ROI"() -> (error out=w107:errorcluster)  [unwired: 3 in, 2 out]
      n140 = local write "New: Trap Density-STS"(w59) -> ()
      n141 = local write "Calc: Trap Density-VT"(w55) -> ()
      n142 = local write "New: Trap Density-VT"(w55) -> ()
      n143 = local write "Calc: Trap Density-STS"(w59) -> ()
      n144 = Unbundle(w72) -> ("[0]"=w71:cluster{dbl[], dbl[]})  [unwired: 8 out]
      n145 = Path To String(path=w100) -> (string=w170:string)
      n146 = Build Path(base path=w103, name or relative path=w101) -> (appended path=w102:path)
      n147 = Index Array(array=w166, index=w167) -> (element=w117:string)
      n148 = local write "Sat Id-Log-Used"(w126) -> ()
      n149 = local write "Vg Array-Log-Used"(w125) -> ()
      n150 = local write "New: Temp"(w60) -> ()
      n151 = local read "No Image File"() -> (w108:path)
      n152 = local write "Lin Vd"(w64) -> ()
      n153 = Empty String/Path?(string/path=w117) -> (empty?=w116:bool)
      n154 = call <vilib>:"Check if File or Folder Exists.vi"("error in (no error)"=w107, "path"=w102) -> ("file or folder exists?"=w105:bool, "dup path"=w106:path)  [unwired: 7 in, 1 out]
      n155 = local write "Image Name"(w117) -> ()
      n156 = Concatenate Strings(w170, "\\", w117) -> (w171:string)
      n157 = Unbundle(w71) -> (w70:dbl[], w69:dbl[])
      n158 = local read "Image Folder"() -> (w149:path)
      n159 = String To Path(string=w171) -> (path=w115:path)
      n160 = case shown="True" w105 {
        tunnel: w106 -> [_ w182]
        frame False {
        }
        frame True {
          n161 = Read from Text File(file (use dialog)=w182) -> (text=w186:string)  [unwired: 3 in, 3 out]
          n162 = property on="Image Out" class="ImageControl"() -> ("ROI"=w183:T12)  [unwired: 2 in, 2 out]
          n163 = Unflatten From String(type=w183, binary string=w186) -> (value=w184:T12, error out=w185:errorcluster)  [unwired: 3 in, 1 out]
          n164 = property on="Image Out" class="ImageControl"(error in=w185, "ROI"=w184) -> ()  [unwired: 1 in, 2 out]
        }
      }
      n165 = List Folder(path=w149) -> (filenames=w145:string[])  [unwired: 3 in, 3 out]
      n166 = Array Subset(array=w69, index=w67, length=w68) -> (w65:dbl[])
      n167 = local read "No Image File"() -> (w109:path)
      n168 = Array Subset(array=w70, index=w67, length=w68) -> (w66:dbl[])
      n169 = call-poly <vilib>:"Read From Spreadsheet File.vi"("file path (dialog if empty)"=w62) -> ("all rows"=w137:string[][])  [unwired: 6 in, 4 out]
      n170 = Select(t=w108, s=w116, f=w115) -> (s? t:f=w114:path)
      n171 = Array Size(array=w137) -> (size(s)=w138:i32[])
      n172 = local write "Image File"(w114) -> ()
      n173 = call "Vision Acquisition6"("Image Path"=w114) -> ("Image Out"=w169:T2)  [unwired: 25 in, 1 out]
      n174 = Index Array(array=w138, index=w139) -> (element=w148:i32)
      n175 = local write "Lin-Vg Array-Used"(w66) -> ()
      n176 = Array Subset(array=w137, index (row)=w139, index (col)=w139, length (col)=3) -> (w136:string[][])  [unwired: 1 in]
      n177 = local write "Lin Id-Used"(w65) -> ()
      n178 = Reshape Array(w136, w148) -> (w153:string[])
      n179 = local write "Image Out"(w169) -> ()
      n180 = local write "Image Out 2"(w169) -> ()
      n181 = Search 1D Array(1D array=w153, element="Index:") -> (index of element=w142:i32)  [unwired: 1 in]
      n182 = Increment(x=w142) -> (x+1=w141:i32)
      n183 = Index Array(array=w153, index=w141) -> (element=w146:string)
      n184 = while {
        tunnel: w145 -> [w194]
        tunnel: w146 -> [w192]
        tunnel: [w191] -> _
        tunnel: [w191] -> w147
        tunnel: w148 -> [w190]
        i -> [w191]
        stop <- w187 stop-if-true
        n185 = Index Array(array=w194, index=w191) -> (element=w195:string)
        n186 = xnode "Match Regular Expression"("input string"=w195, "regular expression"=w192) -> ("whole match"=w193:string)  [unwired: 4 in, 4 out]
        n187 = Equal?(x=w193, y=w192) -> (x = y?=w189:bool)
        n188 = Equal?(x=w190, y=w191) -> (x = y?=w188:bool)
        n189 = Or(x=w189, y=w188) -> (x .or. y?=w187:bool)
      }
      n190 = invoke on="Image Out" class="ImageControl" method="Clear ROI"() -> ()  [unwired: 3 in, 3 out]
      n191 = Path To String(path=w149) -> (string=w150:string)
      n192 = Index Array(array=w145, index=w147) -> (element=w112:string)
      n193 = Empty String/Path?(string/path=w112) -> (empty?=w113:bool)
      n194 = Concatenate Strings(w150, "\\", w112) -> (w151:string)
      n195 = String To Path(string=w151) -> (path=w111:path)
      n196 = Select(t=w109, s=w113, f=w111) -> (s? t:f=w110:path)
      n197 = call "Vision Acquisition2"("Image Path"=w110) -> ("Image Out"=w144:T2)  [unwired: 25 in, 1 out]
      n198 = local write "Image File"(w110) -> ()
      n199 = local write "Image Out"(w144) -> ()
      n200 = local write "Image Out 2"(w144) -> ()
      n201 = local write "Image Name"(w112) -> ()
    }
    frame #2 {
      n202 = while {
        stop <- w526 stop-if-true
        w476 = FALSE
        w474 = 0
        n203 = disable-structure shown="Disabled" {
          frame Disabled {
            w560 = "/"
            n204 = local read "Date Recorded"() -> (w563:string)
            n205 = local read "Ramp (s):"() -> (w530:dbl)
            n206 = local read "RPM:"() -> (w531:dbl)
            n207 = Divide(x=w531, y=w530) -> (x/y=w529:dbl)
            n208 = Match Pattern(string=w563, regular expression=w560) -> (before substring=w554:string, after substring=w561:string)  [unwired: 1 in, 2 out]
            n209 = local write "Accel (RPM/s):"(w529) -> ()
            n210 = String Length(string=w554) -> (length=w557:i32)
            n211 = Match Pattern(string=w561, regular expression=w560) -> (before substring=w548:string, after substring=w559:string)  [unwired: 1 in, 2 out]
            n212 = Equal?(x=w557, y=2) -> (x = y?=w555:bool)
            n213 = String Length(string=w548) -> (length=w550:i32)
            n214 = case shown="False" w555 {
              tunnel: w554 -> [w600 w602]
              tunnel: [w599 w602] -> w553
              frame False {
                n215 = Concatenate Strings("0", w600) -> (w599:string)
              }
              frame True {
              }
            }
            n216 = Equal?(x=w550, y=2) -> (x = y?=w552:bool)
            n217 = case shown="False" w552 {
              tunnel: w548 -> [w596 w598]
              tunnel: [w595 w598] -> w549
              frame False {
                n218 = Concatenate Strings("0", w596) -> (w595:string)
              }
              frame True {
              }
            }
            n219 = local read "Index"() -> (w533:string)
            n220 = local read "Index"() -> (w547:string)
            n221 = local read "Wait Time (s):"() -> (w593:dbl)
            n222 = String Subset(string=w533, length (rest)=1) -> (substring=w588:string)  [unwired: 1 in]
            n223 = local write "Row"(w588) -> ()
            n224 = local read "Treatment Concentration (mM):"() -> (w541:dbl)
            n225 = local read "Rec: Concentration"() -> (w528:dbl)
            n226 = local read "Relative Humidity (%):"() -> (w538:dbl)
            n227 = String Subset(string=w533, offset (0)=1, length (rest)=2) -> (substring=w589:string)
            n228 = Number To Decimal String(number=w593) -> (decimal integer string=w594:string)  [unwired: 1 in]
            n229 = local read "Solution Temp (C):"() -> (w582:dbl)
            n230 = local read "Surface Treatment:"() -> (w540:string)
            n231 = local read "Room Temp (F):"() -> (w586:dbl)
            n232 = local read "Rec: Material"() -> (w536:string)
            n233 = local write "Column"(w589) -> ()
            n234 = local read "New: Length"() -> (w546:dbl)
            n235 = local read "New: Width"() -> (w545:dbl)
            n236 = local read "New: Mobility-Sat"() -> (w575:dbl)
            n237 = local read "Accel (RPM/s):"() -> (w573:dbl)
            n238 = local read "Sample #:"() -> (w565:dbl)
            n239 = local read "# Drops*:"() -> (w583:dbl)
            n240 = local read "Ramp (s):"() -> (w591:dbl)
            n241 = local read "New: STS"() -> (w567:dbl)
            n242 = local read "Rec: Solvent"() -> (w542:string)
            n243 = local read "New: VT-Sat"() -> (w569:dbl)
            n244 = local read "Rec: On/Off"() -> (w571:dbl)
            n245 = local read "Rec: Method"() -> (w566:string)
            n246 = local read "Time (s):"() -> (w578:dbl)
            n247 = local read "Date Recorded"() -> (w562:string)
            n248 = local read "RPM:"() -> (w579:dbl)
            n249 = local read "Fabricator:"() -> (w587:string)
            n250 = Number To Decimal String(number=w528) -> (decimal integer string=w527:string)  [unwired: 1 in]
            n251 = Number To Decimal String(number=w583) -> (decimal integer string=w584:string)  [unwired: 1 in]
            n252 = Number To Decimal String(number=w565) -> (decimal integer string=w558:string)  [unwired: 1 in]
            n253 = call "DeviceID"("Sample"=w558, "Year"=w559, "Month"=w553, "Day"=w549, "Index"=w547) -> ("Result"=w564:string)  [unwired: 9 in, 1 out]
            n254 = Number To Decimal String(number=w546) -> (decimal integer string=w544:string)  [unwired: 1 in]
            n255 = Number To Decimal String(number=w545) -> (decimal integer string=w543:string)  [unwired: 1 in]
            n256 = Number To Decimal String(number=w582) -> (decimal integer string=w581:string)  [unwired: 1 in]
            n257 = Number To Decimal String(number=w538) -> (decimal integer string=w537:string)  [unwired: 1 in]
            n258 = Number To Decimal String(number=w586) -> (decimal integer string=w585:string)  [unwired: 1 in]
            n259 = Number To Decimal String(number=w541) -> (decimal integer string=w539:string)  [unwired: 1 in]
            n260 = Number To Decimal String(number=w579) -> (decimal integer string=w580:string)  [unwired: 1 in]
            n261 = Number To Fractional String(number=w573) -> (F-format string=w574:string)  [unwired: 3 in]
            n262 = Number To Decimal String(number=w578) -> (decimal integer string=w577:string)  [unwired: 1 in]
            n263 = Number To Fractional String(number=w575) -> (F-format string=w576:string)  [unwired: 3 in]
            n264 = Number To Fractional String(number=w571) -> (F-format string=w572:string)  [unwired: 3 in]
            n265 = Number To Fractional String(number=w569) -> (F-format string=w570:string)  [unwired: 3 in]
            n266 = Number To Fractional String(number=w567) -> (F-format string=w568:string)  [unwired: 3 in]
            n267 = Number To Decimal String(number=w591) -> (decimal integer string=w592:string)  [unwired: 1 in]
            n268 = Build Array(w564, w587, w566, w562, w558, w588, w589, w544, w543, w536, w540, w539, w542, w527, w581, w584, w594, w585, w537, w592, w580, w574, w577, w576, w572, w570, w568) -> (w590:string[])
            n269 = local write "Current \nRecord"(w590) -> ()
          }
          frame Enabled {
          }
        }
        n270 = local read "Lin-Vg Array-Used"() -> (w444:dbl[])
        n271 = local read "Sat Id-Log-Used"() -> (w448:dbl[])
        n272 = local read "New: Dielectric"() -> (w441:dbl)
        n273 = local read "Vg Array-Log-Used"() -> (w447:dbl[])
        n274 = local read "New: Length"() -> (w443:dbl)
        n275 = local read "New: Width"() -> (w440:dbl)
        n276 = local read "Lin Id-Used"() -> (w445:dbl[])
        n277 = local read "New: Dielectric"() -> (w437:dbl)
        n278 = local read "Lin Vd"() -> (w439:dbl)
        n279 = local read "Sat Vg Array-Used"() -> (w450:dbl[])
        n280 = local read "New: Dielectric"() -> (w435:dbl)
        n281 = local read "New: Length"() -> (w451:dbl)
        n282 = local read "New: Width"() -> (w453:dbl)
        n283 = local read "Sat Id-Used"() -> (w449:dbl[])
        n284 = call "Mobility-Vt-Used Pts_Linear.vi"("Width"=w440, "Length"=w443, "Vd"=w439, "Dielectric (d)"=w441, "Sat Id Used"=w445, "Vg Used"=w444) -> ("Vt"=w446:dbl, "Mobility"=w442:dbl)  [unwired: 3 in, 1 out]
        n285 = call "STS-Used.vi"("Id Used"=w448, "Vg-Used"=w447) -> ("STS"=w438:dbl)  [unwired: 9 in]
        n286 = local write "New: Mobility-Lin"(w442) -> ()
        n287 = local write "New: VT-Lin"(w446) -> ()
        n288 = call "Mobility-Vt-Used Pts_Saturation.vi"("Width"=w453, "Length"=w451, "Dielectric (d)"=w435, "Sat Id Used"=w449, "Vg Used"=w450) -> ("Vt"=w436:dbl, "Mobility"=w452:dbl)  [unwired: 4 in, 1 out]
        n289 = local write "New: STS"(w438) -> ()
        n290 = local write "New: Mobility-Sat"(w452) -> ()
        n291 = local write "New: VT-Sat"(w436) -> ()
        n292 = call "Trap Density_VT.vi"("VT"=w436, "Dielectric"=w435) -> ("Trap Density-VT"=w434:dbl)
        n293 = local read "Manual-Temp"() -> (w431:bool)
        n294 = local read "Rec: Temp"() -> (w432:dbl)
        n295 = local write "New: Trap Density-VT"(w434) -> ()
        n296 = case shown="False" w431 {
          tunnel: w432 -> [w612 _]
          tunnel: [w609 w616] -> w430
          frame False {
            n297 = local read "Rec: Temp"() -> (w610:dbl)
            n298 = property on="New: Temp" class="DigNum (strict)"("DisabledEnum"=1) -> ()  [unwired: 2 in, 2 out]
            n299 = Equal To 0?(x=w610) -> (x = 0?=w611:bool)
            n300 = local write "New: Temp"(w612) -> ()
            n301 = case shown="True" w611 {
              tunnel: [w613 w614] -> w609
              tunnel: w610 -> [w613 _]
              frame False {
              }
              frame True {
                n302 = local read "Room Temp"() -> (w614:dbl)
              }
            }
            n303 = local write "New: Temp"(w609) -> ()
          }
          frame True {
            n304 = property on="New: Temp" class="DigNum (strict)"("DisabledEnum"=0) -> ()  [unwired: 2 in, 2 out]
            n305 = local read "New: Temp"() -> (w616:dbl)
          }
        }
        n306 = call "Trap Density_STS.vi"("Temp (T) [K]"=w430, "S.T.S. (S)"=w438, "Dielectric"=w437) -> ("Trap Density (N)"=w433:dbl)  [unwired: 8 in]
        n307 = local write "New: Trap Density-STS"(w433) -> ()
        n308 = property on="Image Out" class="ImageControl"() -> ("ZoomSingle"=w494:cluster{"X":sgl, "Y":sgl})  [unwired: 2 in, 2 out]
        n309 = property on="Image Out" class="ImageControl"() -> ("Bounds"=w495:T13)  [unwired: 2 in, 2 out]
        n310 = call <vilib>:"Intialize Keyboard.vi"() -> ("device ID"=w506:refnum<k1>)  [unwired: 10 in, 1 out]
        n311 = property on="Image Out" class="ImageControl"() -> ("Image Center Position"=w501:cluster{"X":u32, "Y":u32})  [unwired: 2 in, 2 out]
        n312 = call-poly <vilib>:"Acquire Input Data.vi"("device ID"=w506) -> ("keys pressed"=w505:T14)  [unwired: 16 in, 2 out]
        n313 = Unbundle(w495) -> ("Width"=w492:u32, "Height"=w491:u32)
        n314 = Unbundle(w494) -> ("X"=w469:sgl, "Y"=w493:sgl)
        n315 = Index Array(array=w505) -> (element=w509:T15)  [unwired: 1 in]
        n316 = event shown="[1] \"Undo Button\": Mouse Down" {
          selector: _ -> [_ _ _ _ _ _ _]
          dyn-events: _ -> [_ _ _ _ _ _ _]
          timeout: 10 -> [_ _ _ _ _ _ _]
          event "Remove Button": Mouse Down {
            w629 = 0
            n317 = event-data() -> ()  [unwired: 1 in, 7 out]
            n318 = property on="Image Out" class="ImageControl"() -> ("ROI"=w627:T12)  [unwired: 2 in, 2 out]
            n319 = Unbundle(w627) -> ("Global Rectangle"=w630:i32[], "Contours"=w632:T16)
            n320 = Reverse 1D Array(array=w630) -> (reversed array=w631:i32[])
            n321 = Reverse 1D Array(array=w632) -> (reversed array=w633:T16)
            n322 = Delete From Array(array=w631, index=w629) -> (array with subset deleted=w634:i32[])  [unwired: 1 in, 1 out]
            n323 = Delete From Array(array=w633, index=w629) -> (array with subset deleted=w635:T16)  [unwired: 1 in, 1 out]
            n324 = Reverse 1D Array(array=w634) -> (reversed array=w636:i32[])
            n325 = Reverse 1D Array(array=w635) -> (reversed array=w637:T16)
            n326 = Bundle(w636, w637) -> (w628:T17)  [unwired: 1 in]
            n327 = local write "ROI Descriptor out"(w627) -> ()
            n328 = local write "ROI Descriptor"(w628) -> ()
            n329 = property on="Image Out" class="ImageControl"("ROI"=w628) -> ()  [unwired: 2 in, 2 out]
          }
          event "Undo Button": Mouse Down {
            n330 = event-data() -> ()  [unwired: 1 in, 7 out]
            n331 = invoke on="Image Out" class="ImageControl" method="Clear ROI"() -> ()  [unwired: 3 in, 3 out]
          }
          event "Image Folder": Value Change {
            n332 = event-data() -> ()  [unwired: 1 in, 5 out]
            n333 = local read "Image File"() -> (w639:path)
            n334 = call "Vision Acquisition"("Image Path"=w639) -> ("Image Out"=w638:T2)  [unwired: 25 in, 1 out]
            n335 = local write "Image Out 2"(w638) -> ()
            n336 = local write "Image Out"(w638) -> ()
            n337 = invoke on="Image Out" class="ImageControl" method="Clear ROI"() -> ()  [unwired: 3 in, 3 out]
          }
          event "Zoom": Value Change {
            n338 = event-data() -> ()  [unwired: 1 in, 5 out]
            n339 = local read "Zoom"() -> (w640:i16)
            n340 = Bundle("Zoom"=w640, "Zoom"=w640) -> (w641:cluster{"Zoom":i16, "Zoom":i16})  [unwired: 1 in]
            n341 = property on="Image Out" class="ImageControl"("ZoomInteger"=w641) -> ()  [unwired: 2 in, 2 out]
          }
          event Timeout {
            n342 = event-data() -> ()  [unwired: 1 in, 2 out]
          }
          event "Image Out": Mouse Enter {
            (unwired) 6
            n343 = event-data() -> ()  [unwired: 1 in, 3 out]
            n344 = call "Simulate_Keyboard.vi"("Action"=0, "Virtual Key"=162) -> ()  [unwired: 7 in, 1 out]
          }
          event "Image Out": Mouse Leave {
            n345 = event-data() -> ()  [unwired: 1 in, 3 out]
            n346 = flat-sequence {
              frame #0 {
                n347 = Wait (ms)(milliseconds to wait=10) -> ()  [unwired: 1 out]
              }
              frame #1 {
                (unwired) 6
                n348 = call "Simulate_Keyboard.vi"("Action"=2, "Virtual Key"=162) -> ()  [unwired: 7 in, 1 out]
              }
            }
          }
        }
        n349 = Divide(x=w492, y=w469) -> (x/y=w482:sgl)
        n350 = Multiply(x=w482, y=0.5) -> (x*y=w488:dbl)
        n351 = Divide(x=w491, y=w493) -> (x/y=w481:sgl)
        n352 = Multiply(x=w481, y=0.5) -> (x*y=w487:dbl)
        n353 = Unbundle(w501) -> ("X"=w483:u32, "Y"=w484:u32)
        n354 = Subtract(x=w484, y=w487) -> (x-y=w485:dbl)
        n355 = Subtract(x=w483, y=w488) -> (x-y=w486:dbl)
        n356 = Add(x=w486, y=w482) -> (x+y=w500:dbl)
        n357 = Add(x=w485, y=w481) -> (x+y=w499:dbl)
        n358 = Reciprocal(x=w469) -> (1/x=w468:sgl)
        n359 = event shown="[6] \"Next Log Sat\": Mouse Down" {
          selector: _ -> [_ _ _ _ _ _ _ _ _ _ _ _ _ _ _ _]
          dyn-events: _ -> [_ _ _ _ _ _ _ _ _ _ _ _ _ _ _ _]
          timeout: 10 -> [_ _ _ _ _ _ _ _ _ _ _ _ _ _ _ _]
          tunnel: [_ _ _ _ _ _ _ _ _ _ _ _ _ TRUE _ TRUE] -> w526
          event Timeout {
            n360 = event-data() -> ()  [unwired: 1 in, 2 out]
          }
          event "Down Button": Mouse Down {
            w906 = "\\"
            w907 = "TSP"
            w1030 = 0
            # "Transpose"
            n361 = event-data() -> ()  [unwired: 1 in, 7 out]
            n362 = local read "Transfer File"() -> (w1035:path)
            n363 = Strip Path(path=w1035) -> (stripped path=w897:path, name=w1043:string)
            n364 = local write "Transfer Folder"(w897) -> ()
            n365 = property on="Image Out" class="ImageControl"() -> (error out=w984:errorcluster, "Image Center Position"=w988:cluster{"X":u32, "Y":u32})  [unwired: 2 in, 1 out]
            n366 = Strip Path(path=w897) -> (stripped path=w902:path)  [unwired: 1 out]
            n367 = List Folder(path=w897) -> (filenames=w1040:string[], error out=w981:errorcluster)  [unwired: 3 in, 2 out]
            n368 = Path To String(path=w902) -> (string=w905:string)
            n369 = invoke on="Image Out" class="ImageControl" method="Clear ROI"() -> ()  [unwired: 3 in, 3 out]
            n370 = local read "Folder Index"() -> (w983:dbl)
            n371 = Array Size(array=w1040) -> (size(s)=w1036:i32)
            n372 = Search 1D Array(1D array=w1040, element=w1043) -> (index of element=w1037:i32)  [unwired: 1 in]
            n373 = Unbundle(w988) -> ("X"=w986:u32)  [unwired: 1 out]
            n374 = Decrement(x=w1036) -> (x-1=w1038:i32)
            n375 = Equal?(x=w1037, y=w1038) -> (x = y?=w1039:bool)
            n376 = local read "Folder Index"() -> (w920:dbl)
            n377 = case shown="False" w1039 {
              tunnel: w983 -> [w1207 _]
              tunnel: [w1206 0] -> w982
              tunnel: w981 -> [w1205 w1208]
              tunnel: [w1205 w1208] -> w980
              frame False {
                n378 = Increment(x=w1207) -> (x+1=w1206:dbl)
              }
              frame True {
              }
            }
            n379 = local write "Folder Index"(w982) -> ()
            n380 = Bundle("X"=w986, 0) -> (w987:cluster{"X":u32, i32})  [unwired: 1 in]
            n381 = property on="Image Out" class="ImageControl"(error in=w984, "Image Center Position"=w987) -> ()  [unwired: 1 in, 2 out]
            n382 = Path To String(path=w897) -> (string=w1044:string)
            n383 = Index Array(array=w1040, index=w982) -> (element=w898:string)
            n384 = String Subset(string=w898, offset (0)=3) -> (substring=w901:string)  [unwired: 1 in]
            n385 = Concatenate Strings(w907, w901) -> (w903:string)
            n386 = Concatenate Strings(w905, w906, w907, w906, w903) -> (w904:string)
            n387 = String To Path(string=w904) -> (path=w899:path)
            n388 = local write "Transport File"(w899) -> ()
            n389 = Strip Path(path=w899) -> (stripped path=w919:path, name=w910:string)
            n390 = local write "Transport Folder"(w919) -> ()
            n391 = List Folder(path=w919) -> (filenames=w914:string[], error out=w922:errorcluster)  [unwired: 3 in, 2 out]
            n392 = Array Size(array=w914) -> (size(s)=w918:i32)
            n393 = Search 1D Array(1D array=w914, element=w910) -> (index of element=w917:i32)  [unwired: 1 in]
            n394 = Decrement(x=w918) -> (x-1=w916:i32)
            n395 = Equal?(x=w917, y=w916) -> (x = y?=w915:bool)
            n396 = case shown="False" w915 {
              tunnel: w920 -> [w1069 _]
              tunnel: [w1068 0] -> w921
              tunnel: w922 -> [w1067 w1070]
              tunnel: [w1067 w1070] -> _
              frame False {
                n397 = Increment(x=w1069) -> (x+1=w1068:dbl)
              }
              frame True {
              }
            }
            n398 = local write "Folder Index"(w921) -> ()
            n399 = local write "Data Name:"(w898) -> ()
            n400 = Path To String(path=w919) -> (string=w909:string)
            n401 = Index Array(array=w914, index=w921) -> (element=w913:string)
            n402 = local write "Data Name:"(w913) -> ()
            n403 = Concatenate Strings(w1044, "\\", w898) -> (w1042:string)
            n404 = Concatenate Strings(w909, "\\", w913) -> (w911:string)
            n405 = String To Path(string=w1042) -> (path=w955:path)
            n406 = call "Recorded Values.vi"("Path"=w955) -> ("Recorded Char"=w1046:T6, "Recorded Prop"=w1047:T7, "Fabrication Prop"=w1045:T8)  [unwired: 8 in]
            n407 = Unbundle By Name(w1046) -> ("Mobility-Sat"=w1059:dbl, "Moblitity-Lin"=w1060:dbl, "On/Off"=w1061:dbl, "Off Current"=w1062:dbl, "Vt-Sat"=w950:dbl, "STS"=w1063:dbl, "Trap Density-VT"=w1064:dbl, "Trap Density-STS"=w1065:dbl)
            n408 = Unbundle By Name(w1045) -> ("Date Created"=w1066:string, "Material"=w1048:string, "Solvent"=w1049:string, "Concentration"=w1050:dbl, "Method"=w1051:string, "Dielectric (nm)"=w1052:dbl, "Treatment"=w1053:string, "Comments"=w1054:string)
            n409 = Unbundle By Name(w1047) -> ("Date Recorded"=w1055:string, "Index"=w1056:string, "Length"=w1057:dbl, "Width"=w1058:dbl, "Sample Temp"=w952:dbl)
            n410 = local write "Date Created"(w1066) -> ()
            n411 = local write "Rec: Off I-Sat"(w1062) -> ()
            n412 = local write "Rec: Comments"(w1054) -> ()
            n413 = local write "Rec: Material"(w1048) -> ()
            n414 = local write "Rec: VT-Sat"(w950) -> ()
            n415 = local write "Rec: Concentration"(w1050) -> ()
            n416 = local write "Rec: Method"(w1051) -> ()
            n417 = local write "Rec: Dielectric (d)"(w1052) -> ()
            n418 = local write "Surface Treatment:"(w1053) -> ()
            n419 = local write "Index"(w1056) -> ()
            n420 = local write "Rec: Mobility-Sat"(w1059) -> ()
            n421 = local write "Rec: Mobility-Lin"(w1060) -> ()
            n422 = local write "Rec: On/Off"(w1061) -> ()
            n423 = local write "Rec: STS"(w1063) -> ()
            n424 = local write "Rec: Trap Density-VT"(w1064) -> ()
            n425 = local write "Rec: Trap Density-STS"(w1065) -> ()
            n426 = local write "Rec: Solvent"(w1049) -> ()
            n427 = local write "Date Recorded"(w1055) -> ()
            n428 = local write "Rec: Length"(w1057) -> ()
            n429 = local write "Rec: Width"(w1058) -> ()
            n430 = local write "Rec: Temp"(w952) -> ()
            n431 = Equal To 0?(x=w952) -> (x = 0?=w953:bool)
            n432 = case shown="True" w953 {
              tunnel: [w1078 w1079] -> w951
              tunnel: w952 -> [w1078 _]
              frame False {
              }
              frame True {
                n433 = local read "Room Temp"() -> (w1079:dbl)
              }
            }
            n434 = String To Path(string=w911) -> (path=w908:path)
            n435 = local read "NumPoints Log"() -> (w976:dbl)
            n436 = local write "Transfer File"(w955) -> ()
            n437 = local read "Num Pts"() -> (w979:dbl)
            n438 = Strip Path(path=w908) -> ()  [unwired: 2 out]
            n439 = call-poly <vilib>:"Read From Spreadsheet File.vi"("file path (dialog if empty)"=w908) -> ("all rows"=w936:string[][])  [unwired: 6 in, 4 out]
            n440 = Array Size(array=w936) -> (size(s)=w942:i32[])
            n441 = call-poly <vilib>:"Read From Spreadsheet File.vi"("file path (dialog if empty)"=w955) -> ("all rows"=w1032:string[][])  [unwired: 6 in, 4 out]
            n442 = call "Mobility-Vt Calculator-File.vi"("NumPts"=w979, "Path"=w955) -> ("Graph Cluster"=w948:T9, "Output"=w978:T10, "Index-Sat"=w977:dbl, "Index-Lin"=w963:dbl)  [unwired: 5 in, 1 out]
            n443 = local read "New: Dielectric"() -> (w960:dbl)
            n444 = call "STS Calculator-File.vi"("NumPts"=w976, "Path"=w955) -> ("STS Index-Sat"=w975:dbl, "XY Graph-Sat"=w974:cluster{dbl[], dbl[]}[], "Ouput"=w973:cluster{"STS-Sat":dbl, "STS-Lin":dbl})  [unwired: 5 in, 2 out]
            n445 = Array Subset(array=w936, length (col)=1) -> (w938:string[][])  [unwired: 3 in]
            n446 = Index Array(array=w942, index=0) -> (element=w931:i32)
            n447 = local write "Sat-Trans Slider"(w977) -> ()
            n448 = Unbundle By Name(w978) -> ("Mobility-Sat"=w972:dbl, "Vt-Sat"=w959:dbl, "Mobility-Lin"=w971:dbl, "Vt-Lin"=w970:dbl, "Off I-Sat"=w956:dbl, "On/Off I-Sat"=w949:dbl)
            n449 = Unbundle By Name(w973) -> ("STS-Sat"=w954:dbl)  [unwired: 1 out]
            n450 = Reshape Array(w938, w931) -> (w937:string[])
            n451 = local write "Index 2"(w975) -> ()
            n452 = local write "MobVi Index"(w977) -> ()
            n453 = local write "Sat-Log"(w974) -> ()
            n454 = Array Size(array=w1032) -> (size(s)=w1031:i32[])
            n455 = Search 1D Array(1D array=w937, element="Vd") -> (index of element=w935:i32)  [unwired: 1 in]
            n456 = Unbundle By Name(w948) -> ("Raw Sat"=w945:cluster{dbl[], dbl[]}[], "Sqrt Sat"=w947:cluster{dbl[], dbl[]}[], "Raw Lin"=w944:cluster{dbl[], dbl[]}[], "Sqrt Lin"=w946:cluster{dbl[], dbl[]}[], "Log Lin"=w943:cluster{dbl[], dbl[]}[])  [unwired: 1 out]
            n457 = local write "Sqrt-Sat"(w947) -> ()
            n458 = call "Trap Density_VT.vi"("VT"=w959, "Dielectric"=w960) -> ("Trap Density-VT"=w958:dbl)
            n459 = call "Trap Density_STS.vi"("Temp (T) [K]"=w951, "S.T.S. (S)"=w954, "Dielectric"=w960) -> ("Trap Density (N)"=w957:dbl)  [unwired: 8 in]
            n460 = local write "New: STS"(w954) -> ()
            n461 = local write "Calc: STS"(w954) -> ()
            n462 = Increment(x=w935) -> (x+1=w934:i32)
            n463 = Array Subset(array=w936, index (row)=w934) -> (w932:string[][])  [unwired: 3 in]
            n464 = Fract/Exp String To Number(string=w932, default (0 dbl)="default (0 dbl) 3") -> (number=w924:ext[][])  [unwired: 2 in, 1 out]
            n465 = local write "Calc: Mobility-Sat"(w972) -> ()
            n466 = local write "Calc: Off I-Sat"(w970) -> ()
            n467 = local write "Calc: Mobility-Lin"(w971) -> ()
            n468 = Index Array(array=w1031, index=w1030) -> (element=w1013:i32)
            n469 = Decimate 1D Array(w974) -> (w1007:cluster{dbl[], dbl[]}[])  [unwired: 1 out]
            n470 = Decimate 1D Array(w947) -> (w1017:cluster{dbl[], dbl[]}[])  [unwired: 1 out]
            n471 = local write "Calc: Off I-Sat"(w956) -> ()
            n472 = local write "Calc: On/Off"(w949) -> ()
            n473 = Decimate 1D Array(w946) -> (w969:cluster{dbl[], dbl[]}[])  [unwired: 1 out]
            n474 = local write "Calc: VT-Sat"(w959) -> ()
            n475 = Array Subset(array=w1032, index (row)=w1030, index (col)=w1030, length (col)=3) -> (w1033:string[][])  [unwired: 1 in]
            n476 = Delete From Array(array=w924) -> (array with subset deleted=w923:ext[][])  [unwired: 3 in, 1 out]
            n477 = local write "Calc: Trap Density-VT"(w958) -> ()
            n478 = local write "Calc: Trap Density-STS"(w957) -> ()
            n479 = local write "New: Trap Density-STS"(w957) -> ()
            n480 = local write "New: Trap Density-VT"(w958) -> ()
            n481 = Array To Cluster(array=w1007) -> (cluster=w1005:T11)
            n482 = Array To Cluster(array=w1017) -> (cluster=w1019:T11)
            n483 = local write "Raw- Sat"(w945) -> ()
            n484 = local write "Sqrt-Lin"(w946) -> ()
            n485 = Delete From Array(array=w923, index (col)=0 ("Deaktivierter Index (Spalte)")) -> (deleted portion=w928:ext[], array with subset deleted=w929:ext[][])  [unwired: 2 in]
            n486 = local write "Raw- Lin"(w944) -> ()
            n487 = local write "New: VT-Lin"(w970) -> ()
            n488 = local write "Log-Lin"(w943) -> ()
            n489 = local write "New: VT-Sat"(w959) -> ()
            n490 = local write "New: Mobility-Sat"(w972) -> ()
            n491 = Transpose 2D Array(2D array=w929) -> (transposed array=w930:ext[][])
            n492 = local write "New: Mobility-Lin"(w971) -> ()
            n493 = Reshape Array(w1033, w1013) -> (w1020:string[])
            n494 = Array To Cluster(array=w969) -> (cluster=w968:T11)
            n495 = Subtract(x=w1013, y=20) -> (x-y=w1012:i32)
            n496 = for {
              tunnel: w928 -> [w1076]
              tunnel: w930 -> [w1077] mode=indexing
              tunnel: [w1075] -> w926 mode=indexing
              n497 = Bundle(w1076, w1077) -> (w1075:cluster{ext[], ext[]})  [unwired: 1 in]
            }
            n498 = property on="Sat-Trans Slider" class="Slide (strict)"("Scale.Maximum"=w1012) -> ()  [unwired: 2 in, 2 out]
            n499 = Unbundle(w1005) -> ("[0]"=w1006:cluster{dbl[], dbl[]})  [unwired: 8 out]
            n500 = Unbundle(w1019) -> ("[0]"=w1018:cluster{dbl[], dbl[]})  [unwired: 8 out]
            n501 = Unbundle(w968) -> ("[0]"=w965:cluster{dbl[], dbl[]})  [unwired: 8 out]
            n502 = Search 1D Array(1D array=w1020, element="Index:") -> (index of element=w1027:i32)  [unwired: 1 in]
            n503 = local write "Transport"(w926) -> ()
            n504 = Array Size(array=w926) -> (size(s)=w925:i32)
            n505 = local read "Num Pts"() -> (w964:dbl)
            n506 = Unbundle(w965) -> (w967:dbl[], w966:dbl[])
            n507 = for {
              N: w925 -> [_]
              i -> [w1074]
              n508 = local read "Transport Line Color"() -> (w1073:u32)
              n509 = local read "Ring"() -> (w1072:u16)
              n510 = property on="Transport" class="XYGraph (strict)"("Active Plot"=w1074, "Plot.Plot Color"=w1073, "Plot.Line Width"=w1072) -> ()  [unwired: 2 in, 2 out]
            }
            n511 = Increment(x=w1027) -> (x+1=w1028:i32)
            n512 = Unbundle(w1006) -> (w1004:dbl[], w1003:dbl[])
            n513 = Unbundle(w1018) -> (w1009:dbl[], w1008:dbl[])
            n514 = Array Subset(array=w967, index=w963, length=w964) -> (w962:dbl[])
            n515 = Array Subset(array=w966, index=w963, length=w964) -> (w961:dbl[])
            n516 = Array Subset(array=w1004, index=w975, length=w976) -> (w1011:dbl[])
            n517 = Array Subset(array=w1003, index=w975, length=w976) -> (w1010:dbl[])
            n518 = Array Subset(array=w1009, index=w977, length=w979) -> (w1016:dbl[])
            n519 = Array Subset(array=w1008, index=w977, length=w979) -> (w1015:dbl[])
            n520 = Index Array(array=w1020, index=w1028) -> (element=w992:string)
            n521 = local write "Lin-Vg Array-Used"(w962) -> ()
            n522 = local write "Sat Vg Array-Used"(w1016) -> ()
            n523 = local write "Vg Array-Log-Used"(w1010) -> ()
            n524 = local write "Lin Id-Used"(w961) -> ()
            n525 = local read "Image Folder"() -> (w990:path)
            n526 = local write "Sat Id-Used"(w1015) -> ()
            n527 = local write "Sat Id-Log-Used"(w1011) -> ()
            n528 = List Folder(path=w990, error in=w980) -> (filenames=w1026:string[], error out=w993:errorcluster)  [unwired: 2 in, 2 out]
            n529 = while {
              tunnel: w1026 -> [w1092]
              tunnel: w992 -> [w1090]
              tunnel: [w1089] -> _
              tunnel: [w1089] -> w1025
              tunnel: w1013 -> [w1088]
              i -> [w1089]
              stop <- w1085 stop-if-true
              n530 = Index Array(array=w1092, index=w1089) -> (element=w1093:string)
              n531 = xnode "Match Regular Expression"("input string"=w1093, "regular expression"=w1090) -> ("whole match"=w1091:string)  [unwired: 4 in, 4 out]
              n532 = Equal?(x=w1091, y=w1090) -> (x = y?=w1087:bool)
              n533 = Equal?(x=w1088, y=w1089) -> (x = y?=w1086:bool)
              n534 = Or(x=w1087, y=w1086) -> (x .or. y?=w1085:bool)
            }
            n535 = Build Path(base path=w990, name or relative path="ROI") -> (appended path=w989:path)
            n536 = Path To String(path=w990) -> (string=w1023:string)
            n537 = Index Array(array=w1026, index=w1025) -> (element=w1001:string)
            n538 = invoke on="Image Out" class="ImageControl" method="Clear ROI"(error in=w993) -> (error out=w996:errorcluster)  [unwired: 2 in, 2 out]
            n539 = local write "Image Name"(w1001) -> ()
            n540 = Build Path(base path=w989, name or relative path=w992) -> (appended path=w997:path)
            n541 = call <vilib>:"Check if File or Folder Exists.vi"("error in (no error)"=w996, "path"=w997) -> ("file or folder exists?"=w994:bool, "dup path"=w995:path)  [unwired: 7 in, 1 out]
            n542 = Concatenate Strings(w1023, "\\", w1001) -> (w1022:string)
            n543 = case shown="False" w994 {
              tunnel: w995 -> [_ w1080]
              frame False {
              }
              frame True {
                n544 = Read from Text File(file (use dialog)=w1080) -> (text=w1084:string)  [unwired: 3 in, 3 out]
                n545 = property on="Image Out" class="ImageControl"() -> ("ROI"=w1081:T12)  [unwired: 2 in, 2 out]
                n546 = Unflatten From String(type=w1081, binary string=w1084) -> (value=w1082:T12, error out=w1083:errorcluster)  [unwired: 3 in, 1 out]
                n547 = property on="Image Out" class="ImageControl"(error in=w1083, "ROI"=w1082) -> ()  [unwired: 1 in, 2 out]
              }
            }
            n548 = String To Path(string=w1022) -> (path=w1000:path)
            n549 = Empty String/Path?(string/path=w1001) -> (empty?=w1002:bool)
            n550 = local read "No Image File"() -> (w998:path)
            n551 = Select(t=w998, s=w1002, f=w1000) -> (s? t:f=w999:path)
            n552 = local write "Image File"(w999) -> ()
            n553 = call "Vision Acquisition4"("Image Path"=w999) -> ("Image Out"=w1024:T2)  [unwired: 25 in, 1 out]
            n554 = local write "Image Out"(w1024) -> ()
            n555 = local write "Image Out 2"(w1024) -> ()
          }
          event "Transfer File": Value Change {
            w1220 = "\\"
            w1221 = "TSP"
            w1359 = 0
            # "Transpose"
            n556 = event-data() -> ()  [unwired: 1 in, 5 out]
            n557 = local read "Transfer File"() -> (w1355:path)
            n558 = Strip Path(path=w1355) -> (stripped path=w1211:path, name=w1367:string)
            n559 = local write "Transfer Folder"(w1211) -> ()
            n560 = property on="Image Out" class="ImageControl"() -> (error out=w1311:errorcluster, "Image Center Position"=w1315:cluster{"X":u32, "Y":u32})  [unwired: 2 in, 1 out]
            n561 = List Folder(path=w1211) -> (filenames=w1364:string[], error out=w1321:errorcluster)  [unwired: 3 in, 2 out]
            n562 = Strip Path(path=w1211) -> (stripped path=w1216:path)  [unwired: 1 out]
            n563 = Search 1D Array(1D array=w1364, element=w1367) -> (index of element=w1310:i32)  [unwired: 1 in]
            n564 = Path To String(path=w1216) -> (string=w1219:string)
            n565 = local write "Folder Index"(w1310) -> ()
            n566 = Unbundle(w1315) -> ("X"=w1313:u32)  [unwired: 1 out]
            n567 = Path To String(path=w1211) -> (string=w1368:string)
            n568 = Index Array(array=w1364, index=w1310) -> (element=w1212:string)
            n569 = String Subset(string=w1212, offset (0)=3) -> (substring=w1215:string)  [unwired: 1 in]
            n570 = Concatenate Strings(w1221, w1215) -> (w1217:string)
            n571 = Concatenate Strings(w1219, w1220, w1221, w1220, w1217) -> (w1218:string)
            n572 = Bundle("X"=w1313, 0) -> (w1314:cluster{"X":u32, i32})  [unwired: 1 in]
            n573 = String To Path(string=w1218) -> (path=w1213:path)
            n574 = local write "Transport File"(w1213) -> ()
            n575 = Strip Path(path=w1213) -> (stripped path=w1242:path, name=w1247:string)
            n576 = local write "Transport Folder"(w1242) -> ()
            n577 = local write "Data Name:"(w1212) -> ()
            n578 = property on="Image Out" class="ImageControl"(error in=w1311, "Image Center Position"=w1314) -> ()  [unwired: 1 in, 2 out]
            n579 = List Folder(path=w1242) -> (filenames=w1243:string[])  [unwired: 3 in, 3 out]
            n580 = Search 1D Array(1D array=w1243, element=w1247) -> (index of element=w1210:i32)  [unwired: 1 in]
            n581 = Concatenate Strings(w1368, "\\", w1212) -> (w1366:string)
            n582 = String To Path(string=w1366) -> (path=w1262:path)
            n583 = call "Recorded Values.vi"("Path"=w1262) -> ("Recorded Char"=w1308:T6, "Recorded Prop"=w1307:T7, "Fabrication Prop"=w1309:T8)  [unwired: 8 in]
            n584 = Unbundle By Name(w1308) -> ("Mobility-Sat"=w1295:dbl, "Moblitity-Lin"=w1294:dbl, "On/Off"=w1293:dbl, "Off Current"=w1292:dbl, "Vt-Sat"=w1258:dbl, "STS"=w1291:dbl, "Trap Density-VT"=w1290:dbl, "Trap Density-STS"=w1289:dbl)
            n585 = Unbundle By Name(w1309) -> ("Date Created"=w1288:string, "Material"=w1306:string, "Solvent"=w1305:string, "Concentration"=w1304:dbl, "Method"=w1303:string, "Dielectric (nm)"=w1302:dbl, "Treatment"=w1301:string, "Comments"=w1300:string)
            n586 = Unbundle By Name(w1307) -> ("Date Recorded"=w1299:string, "Index"=w1298:string, "Length"=w1297:dbl, "Width"=w1296:dbl, "Sample Temp"=w1260:dbl)
            n587 = local write "Date Created"(w1288) -> ()
            n588 = local write "Rec: Material"(w1306) -> ()
            n589 = local write "Rec: Off I-Sat"(w1292) -> ()
            n590 = local write "Rec: Comments"(w1300) -> ()
            n591 = local write "Rec: VT-Sat"(w1258) -> ()
            n592 = local write "Rec: Concentration"(w1304) -> ()
            n593 = local write "Rec: Method"(w1303) -> ()
            n594 = local write "Rec: Dielectric (d)"(w1302) -> ()
            n595 = local write "Surface Treatment:"(w1301) -> ()
            n596 = local write "Index"(w1298) -> ()
            n597 = local write "Rec: Mobility-Sat"(w1295) -> ()
            n598 = local write "Rec: Mobility-Lin"(w1294) -> ()
            n599 = local write "Rec: On/Off"(w1293) -> ()
            n600 = local write "Rec: STS"(w1291) -> ()
            n601 = local write "Rec: Trap Density-VT"(w1290) -> ()
            n602 = local write "Rec: Trap Density-STS"(w1289) -> ()
            n603 = local write "Rec: Solvent"(w1305) -> ()
            n604 = local write "Date Recorded"(w1299) -> ()
            n605 = local write "Rec: Length"(w1297) -> ()
            n606 = local write "Rec: Width"(w1296) -> ()
            n607 = local write "Rec: Temp"(w1260) -> ()
            n608 = Equal To 0?(x=w1260) -> (x = 0?=w1261:bool)
            n609 = case shown="True" w1261 {
              tunnel: [w1375 w1376] -> w1259
              tunnel: w1260 -> [w1375 _]
              frame False {
              }
              frame True {
                n610 = local read "Room Temp"() -> (w1376:dbl)
              }
            }
            n611 = local write "Folder Index"(w1210) -> ()
            n612 = local read "NumPoints Log"() -> (w1284:dbl)
            n613 = local write "Transfer File"(w1262) -> ()
            n614 = local read "Num Pts"() -> (w1285:dbl)
            n615 = Path To String(path=w1242) -> (string=w1248:string)
            n616 = call-poly <vilib>:"Read From Spreadsheet File.vi"("file path (dialog if empty)"=w1262) -> ("all rows"=w1361:string[][])  [unwired: 6 in, 4 out]
            n617 = Index Array(array=w1243, index=w1210) -> (element=w1244:string)
            n618 = local read "New: Dielectric"() -> (w1268:dbl)
            n619 = call "STS Calculator-File.vi"("NumPts"=w1284, "Path"=w1262) -> ("STS Index-Sat"=w1282:dbl, "XY Graph-Sat"=w1283:cluster{dbl[], dbl[]}[], "Ouput"=w1281:cluster{"STS-Sat":dbl, "STS-Lin":dbl})  [unwired: 5 in, 2 out]
            n620 = call "Mobility-Vt Calculator-File.vi"("NumPts"=w1285, "Path"=w1262) -> ("Graph Cluster"=w1255:T9, "Output"=w1286:T10, "Index-Sat"=w1287:dbl, "Index-Lin"=w1274:dbl)  [unwired: 5 in, 1 out]
            n621 = local write "Data Name:"(w1244) -> ()
            n622 = Unbundle By Name(w1286) -> ("Mobility-Sat"=w1270:dbl, "Vt-Sat"=w1264:dbl, "Mobility-Lin"=w1269:dbl, "Vt-Lin"=w1256:dbl, "Off I-Sat"=w1263:dbl, "On/Off I-Sat"=w1257:dbl)
            n623 = local write "Index 2"(w1282) -> ()
            n624 = Unbundle By Name(w1281) -> ("STS-Sat"=w1265:dbl)  [unwired: 1 out]
            n625 = local write "MobVi Index"(w1287) -> ()
            n626 = local write "Sat-Log"(w1283) -> ()
            n627 = Concatenate Strings(w1248, "\\", w1244) -> (w1246:string)
            n628 = local write "Sat-Trans Slider"(w1287) -> ()
            n629 = Array Size(array=w1361) -> (size(s)=w1360:i32[])
            n630 = call "Trap Density_VT.vi"("VT"=w1264, "Dielectric"=w1268) -> ("Trap Density-VT"=w1267:dbl)
            n631 = call "Trap Density_STS.vi"("Temp (T) [K]"=w1259, "S.T.S. (S)"=w1265, "Dielectric"=w1268) -> ("Trap Density (N)"=w1266:dbl)  [unwired: 8 in]
            n632 = String To Path(string=w1246) -> (path=w1249:path)
            n633 = local write "Calc: Mobility-Lin"(w1269) -> ()
            n634 = local write "Calc: Mobility-Sat"(w1270) -> ()
            n635 = local write "Calc: VT-Sat"(w1264) -> ()
            n636 = local write "Calc: Off I-Sat"(w1263) -> ()
            n637 = local write "Calc: VT-Lin"(w1256) -> ()
            n638 = local write "Calc: On/Off"(w1257) -> ()
            n639 = local write "Calc: STS"(w1265) -> ()
            n640 = Strip Path(path=w1249) -> ()  [unwired: 2 out]
            n641 = Unbundle By Name(w1255) -> ("Raw Sat"=w1252:cluster{dbl[], dbl[]}[], "Sqrt Sat"=w1253:cluster{dbl[], dbl[]}[], "Raw Lin"=w1251:cluster{dbl[], dbl[]}[], "Sqrt Lin"=w1254:cluster{dbl[], dbl[]}[], "Log Lin"=w1250:cluster{dbl[], dbl[]}[])  [unwired: 1 out]
            n642 = call-poly <vilib>:"Read From Spreadsheet File.vi"("file path (dialog if empty)"=w1249) -> ("all rows"=w1228:string[][])  [unwired: 6 in, 4 out]
            n643 = Decimate 1D Array(w1254) -> (w1280:cluster{dbl[], dbl[]}[])  [unwired: 1 out]
            n644 = local write "Calc: Trap Density-VT"(w1267) -> ()
            n645 = local write "Calc: Trap Density-STS"(w1266) -> ()
            n646 = local write "New: Trap Density-STS"(w1266) -> ()
            n647 = local write "New: Trap Density-VT"(w1267) -> ()
            n648 = local write "Sqrt-Lin"(w1254) -> ()
            n649 = Array Size(array=w1228) -> (size(s)=w1222:i32[])
            n650 = local write "New: VT-Sat"(w1264) -> ()
            n651 = Decimate 1D Array(w1283) -> (w1336:cluster{dbl[], dbl[]}[])  [unwired: 1 out]
            n652 = Index Array(array=w1360, index=w1359) -> (element=w1342:i32)
            n653 = Decimate 1D Array(w1253) -> (w1345:cluster{dbl[], dbl[]}[])  [unwired: 1 out]
            n654 = local write "Sqrt-Sat"(w1253) -> ()
            n655 = local write "New: Mobility-Lin"(w1269) -> ()
            n656 = Array Subset(array=w1361, index (row)=w1359, index (col)=w1359, length (col)=3) -> (w1362:string[][])  [unwired: 1 in]
            n657 = local write "New: VT-Lin"(w1256) -> ()
            n658 = Array To Cluster(array=w1280) -> (cluster=w1279:T11)
            n659 = local write "New: STS"(w1265) -> ()
            n660 = local write "New: Mobility-Sat"(w1270) -> ()
            n661 = Array Subset(array=w1228, length (col)=1) -> (w1226:string[][])  [unwired: 3 in]
            n662 = Index Array(array=w1222, index=0) -> (element=w1233:i32)
            n663 = Array To Cluster(array=w1336) -> (cluster=w1334:T11)
            n664 = Array To Cluster(array=w1345) -> (cluster=w1347:T11)
            n665 = Reshape Array(w1362, w1342) -> (w1348:string[])
            n666 = Subtract(x=w1342, y=20) -> (x-y=w1340:i32)
            n667 = local write "Raw- Sat"(w1252) -> ()
            n668 = Unbundle(w1279) -> ("[0]"=w1278:cluster{dbl[], dbl[]})  [unwired: 8 out]
            n669 = Reshape Array(w1226, w1233) -> (w1227:string[])
            n670 = local write "Raw- Lin"(w1251) -> ()
            n671 = local read "Num Pts"() -> (w1275:dbl)
            n672 = property on="Sat-Trans Slider" class="Slide (strict)"("Scale.Maximum"=w1340) -> ()  [unwired: 2 in, 2 out]
            n673 = local write "Log-Lin"(w1250) -> ()
            n674 = Unbundle(w1278) -> (w1277:dbl[], w1276:dbl[])
            n675 = Unbundle(w1334) -> ("[0]"=w1335:cluster{dbl[], dbl[]})  [unwired: 8 out]
            n676 = Unbundle(w1347) -> ("[0]"=w1346:cluster{dbl[], dbl[]})  [unwired: 8 out]
            n677 = Search 1D Array(1D array=w1227, element="Vd") -> (index of element=w1229:i32)  [unwired: 1 in]
            n678 = Search 1D Array(1D array=w1348, element="Index:") -> (index of element=w1356:i32)  [unwired: 1 in]
            n679 = local read "Num Pts"() -> (w1271:dbl)
            n680 = Increment(x=w1229) -> (x+1=w1230:i32)
            n681 = Array Subset(array=w1228, index (row)=w1230) -> (w1232:string[][])  [unwired: 3 in]
            n682 = Array Subset(array=w1277, index=w1274, length=w1275) -> (w1273:dbl[])
            n683 = Array Subset(array=w1276, index=w1274, length=w1275) -> (w1272:dbl[])
            n684 = Increment(x=w1356) -> (x+1=w1357:i32)
            n685 = Unbundle(w1335) -> (w1332:dbl[], w1331:dbl[])
            n686 = Unbundle(w1346) -> (w1333:dbl[], w1337:dbl[])
            n687 = Fract/Exp String To Number(string=w1232, default (0 dbl)="default (0 dbl) 5") -> (number=w1240:ext[][])  [unwired: 2 in, 1 out]
            n688 = Delete From Array(array=w1240) -> (array with subset deleted=w1241:ext[][])  [unwired: 3 in, 1 out]
            n689 = local read "Image Folder"() -> (w1317:path)
            n690 = Delete From Array(array=w1241, index (col)=0 ("Deaktivierter Index (Spalte)")) -> (deleted portion=w1236:ext[], array with subset deleted=w1235:ext[][])  [unwired: 2 in]
            n691 = local write "Lin-Vg Array-Used"(w1273) -> ()
            n692 = Array Subset(array=w1332, index=w1282, length=w1284) -> (w1339:dbl[])
            n693 = Array Subset(array=w1331, index=w1282, length=w1284) -> (w1338:dbl[])
            n694 = Array Subset(array=w1333, index=w1287, length=w1271) -> (w1344:dbl[])
            n695 = Array Subset(array=w1337, index=w1287, length=w1271) -> (w1343:dbl[])
            n696 = Index Array(array=w1348, index=w1357) -> (element=w1319:string)
            n697 = local write "Lin Id-Used"(w1272) -> ()
            n698 = Transpose 2D Array(2D array=w1235) -> (transposed array=w1234:ext[][])
            n699 = local write "Sat Vg Array-Used"(w1344) -> ()
            n700 = local write "Vg Array-Log-Used"(w1338) -> ()
            n701 = for {
              tunnel: w1236 -> [w1373]
              tunnel: w1234 -> [w1374] mode=indexing
              tunnel: [w1372] -> w1238 mode=indexing
              n702 = Bundle(w1373, w1374) -> (w1372:cluster{ext[], ext[]})  [unwired: 1 in]
            }
            n703 = local write "Sat Id-Log-Used"(w1339) -> ()
            n704 = local write "Sat Id-Used"(w1343) -> ()
            n705 = local write "Index"(w1319) -> ()
            n706 = List Folder(path=w1317, error in=w1321) -> (filenames=w1353:string[], error out=w1320:errorcluster)  [unwired: 2 in, 2 out]
            n707 = Build Path(base path=w1317, name or relative path="ROI") -> (appended path=w1316:path)
            n708 = local write "Transport"(w1238) -> ()
            n709 = Array Size(array=w1238) -> (size(s)=w1239:i32)
            n710 = invoke on="Image Out" class="ImageControl" method="Clear ROI"(error in=w1320) -> (error out=w1324:errorcluster)  [unwired: 2 in, 2 out]
            n711 = Build Path(base path=w1316, name or relative path=w1319) -> (appended path=w1325:path)
            n712 = while {
              tunnel: w1353 -> [w1389]
              tunnel: w1319 -> [w1387]
              tunnel: [w1386] -> _
              tunnel: [w1386] -> w1352
              tunnel: w1342 -> [w1385]
              i -> [w1386]
              stop <- w1382 stop-if-true
              n713 = Index Array(array=w1389, index=w1386) -> (element=w1390:string)
              n714 = xnode "Match Regular Expression"("input string"=w1390, "regular expression"=w1387) -> ("whole match"=w1388:string)  [unwired: 4 in, 4 out]
              n715 = Equal?(x=w1388, y=w1387) -> (x = y?=w1384:bool)
              n716 = Equal?(x=w1385, y=w1386) -> (x = y?=w1383:bool)
              n717 = Or(x=w1384, y=w1383) -> (x .or. y?=w1382:bool)
            }
            n718 = for {
              N: w1239 -> [_]
              i -> [w1371]
              n719 = local read "Transport Line Color"() -> (w1370:u32)
              n720 = local read "Ring"() -> (w1369:u16)
              n721 = property on="Transport" class="XYGraph (strict)"("Active Plot"=w1371, "Plot.Plot Color"=w1370, "Plot.Line Width"=w1369) -> ()  [unwired: 2 in, 2 out]
            }
            n722 = call <vilib>:"Check if File or Folder Exists.vi"("error in (no error)"=w1324, "path"=w1325) -> ("file or folder exists?"=w1322:bool, "dup path"=w1323:path)  [unwired: 7 in, 1 out]
            n723 = case shown="True" w1322 {
              tunnel: w1323 -> [_ w1377]
              frame False {
              }
              frame True {
                n724 = Read from Text File(file (use dialog)=w1377) -> (text=w1381:string)  [unwired: 3 in, 3 out]
                n725 = property on="Image Out" class="ImageControl"() -> ("ROI"=w1378:T12)  [unwired: 2 in, 2 out]
                n726 = Unflatten From String(type=w1378, binary string=w1381) -> (value=w1379:T12, error out=w1380:errorcluster)  [unwired: 3 in, 1 out]
                n727 = property on="Image Out" class="ImageControl"(error in=w1380, "ROI"=w1379) -> ()  [unwired: 1 in, 2 out]
              }
            }
            n728 = invoke on="Image Out" class="ImageControl" method="Clear ROI"() -> ()  [unwired: 3 in, 3 out]
            n729 = Path To String(path=w1317) -> (string=w1351:string)
            n730 = Index Array(array=w1353, index=w1352) -> (element=w1329:string)
            n731 = Concatenate Strings(w1351, "\\", w1329) -> (w1350:string)
            n732 = local write "Image Name"(w1329) -> ()
            n733 = String To Path(string=w1350) -> (path=w1328:path)
            n734 = Empty String/Path?(string/path=w1329) -> (empty?=w1330:bool)
            n735 = local read "No Image File"() -> (w1326:path)
            n736 = Select(t=w1326, s=w1330, f=w1328) -> (s? t:f=w1327:path)
            n737 = local write "Image File"(w1327) -> ()
            n738 = call "Vision Acquisition3"("Image Path"=w1327) -> ("Image Out"=w1354:T2)  [unwired: 25 in, 1 out]
            n739 = local write "Image Out"(w1354) -> ()
            n740 = local write "Image Out 2"(w1354) -> ()
          }
          event "Up Button": Mouse Down {
            w1514 = "\\"
            w1515 = "TSP"
            w1657 = 0
            # "Transpose"
            n741 = event-data() -> ()  [unwired: 1 in, 5 out]
            n742 = local read "Transfer File"() -> (w1653:path)
            n743 = Strip Path(path=w1653) -> (stripped path=w1506:path, name=w1667:string)
            n744 = local write "Transfer Folder"(w1506) -> ()
            n745 = List Folder(path=w1506) -> (filenames=w1662:string[], error out=w1620:errorcluster)  [unwired: 3 in, 2 out]
            n746 = Array Size(array=w1662) -> (size(s)=w1608:i32)
            n747 = Search 1D Array(1D array=w1662, element=w1667) -> (index of element=w1663:i32)  [unwired: 1 in]
            n748 = Equal To 0?(x=w1663) -> (x = 0?=w1664:bool)
            n749 = local read "Folder Index"() -> (w1607:dbl)
            n750 = property on="Image Out" class="ImageControl"() -> (error out=w1610:errorcluster, "Image Center Position"=w1614:cluster{"X":u32, "Y":u32})  [unwired: 2 in, 1 out]
            n751 = Strip Path(path=w1506) -> (stripped path=w1510:path)  [unwired: 1 out]
            n752 = Path To String(path=w1510) -> (string=w1513:string)
            n753 = case shown="True" w1664 {
              tunnel: w1607 -> [w1808 _]
              tunnel: [w1807 w1809] -> w1606
              tunnel: w1608 -> [_ w1810]
              frame False {
                n754 = Decrement(x=w1808) -> (x-1=w1807:dbl)
              }
              frame True {
                n755 = Decrement(x=w1810) -> (x-1=w1809:i32)
              }
            }
            n756 = Unbundle(w1614) -> ("X"=w1612:u32)  [unwired: 1 out]
            n757 = local write "Folder Index"(w1606) -> ()
            n758 = local read "Folder Index"() -> (w1538:dbl)
            n759 = Bundle("X"=w1612, 0) -> (w1613:cluster{"X":u32, i32})  [unwired: 1 in]
            n760 = Path To String(path=w1506) -> (string=w1668:string)
            n761 = Index Array(array=w1662, index=w1606) -> (element=w1507:string)
            n762 = String Subset(string=w1507, offset (0)=3) -> (substring=w1509:string)  [unwired: 1 in]
            n763 = Concatenate Strings(w1515, w1509) -> (w1511:string)
            n764 = Concatenate Strings(w1513, w1514, w1515, w1514, w1511) -> (w1512:string)
            n765 = String To Path(string=w1512) -> (path=w1505:path)
            n766 = local write "Transport File"(w1505) -> ()
            n767 = Strip Path(path=w1505) -> (stripped path=w1539:path, name=w1544:string)
            n768 = local write "Transport Folder"(w1539) -> ()
            n769 = List Folder(path=w1539) -> (filenames=w1540:string[], error out=w1536:errorcluster)  [unwired: 3 in, 2 out]
            n770 = Array Size(array=w1540) -> (size(s)=w1502:i32)
            n771 = Search 1D Array(1D array=w1540, element=w1544) -> (index of element=w1504:i32)  [unwired: 1 in]
            n772 = local write "Data Name:"(w1507) -> ()
            n773 = property on="Image Out" class="ImageControl"(error in=w1610, "Image Center Position"=w1613) -> ()  [unwired: 1 in, 2 out]
            n774 = Equal To 0?(x=w1504) -> (x = 0?=w1503:bool)
            n775 = case shown="False" w1503 {
              tunnel: w1538 -> [w1671 _]
              tunnel: [w1670 w1672] -> w1537
              tunnel: w1536 -> [w1669 w1673]
              tunnel: [w1669 w1673] -> _
              tunnel: w1502 -> [_ w1672]
              frame False {
                n776 = Decrement(x=w1671) -> (x-1=w1670:dbl)
              }
              frame True {
              }
            }
            n777 = local write "Folder Index"(w1537) -> ()
            n778 = Concatenate Strings(w1668, "\\", w1507) -> (w1666:string)
            n779 = Path To String(path=w1539) -> (string=w1545:string)
            n780 = Index Array(array=w1540, index=w1537) -> (element=w1541:string)
            n781 = String To Path(string=w1666) -> (path=w1558:path)
            n782 = call "Recorded Values.vi"("Path"=w1558) -> ("Recorded Char"=w1604:T6, "Recorded Prop"=w1603:T7, "Fabrication Prop"=w1605:T8)  [unwired: 8 in]
            n783 = Unbundle By Name(w1604) -> ("Mobility-Sat"=w1591:dbl, "Moblitity-Lin"=w1590:dbl, "On/Off"=w1589:dbl, "Off Current"=w1588:dbl, "Vt-Sat"=w1554:dbl, "STS"=w1587:dbl, "Trap Density-VT"=w1586:dbl, "Trap Density-STS"=w1585:dbl)
            n784 = Unbundle By Name(w1605) -> ("Date Created"=w1584:string, "Material"=w1602:string, "Solvent"=w1601:string, "Concentration"=w1600:dbl, "Method"=w1599:string, "Dielectric (nm)"=w1598:dbl, "Treatment"=w1597:string, "Comments"=w1596:string)
            n785 = Unbundle By Name(w1603) -> ("Date Recorded"=w1595:string, "Index"=w1594:string, "Length"=w1593:dbl, "Width"=w1592:dbl, "Sample Temp"=w1555:dbl)
            n786 = local write "Date Created"(w1584) -> ()
            n787 = local write "Rec: Material"(w1602) -> ()
            n788 = local write "Rec: Off I-Sat"(w1588) -> ()
            n789 = local write "Rec: Comments"(w1596) -> ()
            n790 = local write "Rec: VT-Sat"(w1554) -> ()
            n791 = local write "Rec: Solvent"(w1601) -> ()
            n792 = local write "Rec: Concentration"(w1600) -> ()
            n793 = local write "Rec: Method"(w1599) -> ()
            n794 = local write "Rec: Dielectric (d)"(w1598) -> ()
            n795 = local write "Surface Treatment:"(w1597) -> ()
            n796 = local write "Index"(w1594) -> ()
            n797 = local write "Rec: Mobility-Sat"(w1591) -> ()
            n798 = local write "Rec: Mobility-Lin"(w1590) -> ()
            n799 = local write "Rec: On/Off"(w1589) -> ()
            n800 = local write "Rec: STS"(w1587) -> ()
            n801 = local write "Rec: Trap Density-VT"(w1586) -> ()
            n802 = local write "Rec: Trap Density-STS"(w1585) -> ()
            n803 = local write "Date Recorded"(w1595) -> ()
            n804 = local write "Rec: Length"(w1593) -> ()
            n805 = local write "Rec: Width"(w1592) -> ()
            n806 = local write "Rec: Temp"(w1555) -> ()
            n807 = Equal To 0?(x=w1555) -> (x = 0?=w1557:bool)
            n808 = case shown="False" w1557 {
              tunnel: [w1680 w1681] -> w1556
              tunnel: w1555 -> [w1680 _]
              frame False {
              }
              frame True {
                n809 = local read "Room Temp"() -> (w1681:dbl)
              }
            }
            n810 = local write "Data Name:"(w1541) -> ()
            n811 = local read "NumPoints Log"() -> (w1580:dbl)
            n812 = local write "Transfer File"(w1558) -> ()
            n813 = local read "Num Pts"() -> (w1583:dbl)
            n814 = Concatenate Strings(w1545, "\\", w1541) -> (w1543:string)
            n815 = local read "New: Dielectric"() -> (w1564:dbl)
            n816 = call "Mobility-Vt Calculator-File.vi"("NumPts"=w1583, "Path"=w1558) -> ("Graph Cluster"=w1552:T9, "Output"=w1582:T10, "Index-Sat"=w1581:dbl, "Index-Lin"=w1568:dbl)  [unwired: 5 in, 1 out]
            n817 = call "STS Calculator-File.vi"("NumPts"=w1580, "Path"=w1558) -> ("STS Index-Sat"=w1579:dbl, "XY Graph-Sat"=w1578:cluster{dbl[], dbl[]}[], "Ouput"=w1577:cluster{"STS-Sat":dbl, "STS-Lin":dbl})  [unwired: 5 in, 2 out]
            n818 = call-poly <vilib>:"Read From Spreadsheet File.vi"("file path (dialog if empty)"=w1558) -> ("all rows"=w1659:string[][])  [unwired: 6 in, 4 out]
            n819 = String To Path(string=w1543) -> (path=w1546:path)
            n820 = Unbundle By Name(w1582) -> ("Mobility-Sat"=w1567:dbl, "Vt-Sat"=w1560:dbl, "Mobility-Lin"=w1566:dbl, "Vt-Lin"=w1565:dbl, "Off I-Sat"=w1559:dbl, "On/Off I-Sat"=w1553:dbl)
            n821 = Strip Path(path=w1546) -> ()  [unwired: 2 out]
            n822 = call-poly <vilib>:"Read From Spreadsheet File.vi"("file path (dialog if empty)"=w1546) -> ("all rows"=w1522:string[][])  [unwired: 6 in, 4 out]
            n823 = local write "Sat-Trans Slider"(w1581) -> ()
            n824 = Unbundle By Name(w1577) -> ("STS-Sat"=w1561:dbl)  [unwired: 1 out]
            n825 = local write "Index 2"(w1579) -> ()
            n826 = local write "MobVi Index"(w1581) -> ()
            n827 = local write "Sat-Log"(w1578) -> ()
            n828 = Array Size(array=w1522) -> (size(s)=w1516:i32[])
            n829 = local write "Calc: Mobility-Sat"(w1567) -> ()
            n830 = local write "Calc: VT-Sat"(w1560) -> ()
            n831 = local write "Calc: Mobility-Lin"(w1566) -> ()
            n832 = local write "Calc: Off I-Sat"(w1559) -> ()
            n833 = local write "Calc: On/Off"(w1553) -> ()
            n834 = Array Size(array=w1659) -> (size(s)=w1658:i32[])
            n835 = local write "Calc: VT-Lin"(w1565) -> ()
            n836 = call "Trap Density_VT.vi"("VT"=w1560, "Dielectric"=w1564) -> ("Trap Density-VT"=w1563:dbl)
            n837 = call "Trap Density_STS.vi"("Temp (T) [K]"=w1556, "S.T.S. (S)"=w1561, "Dielectric"=w1564) -> ("Trap Density (N)"=w1562:dbl)  [unwired: 8 in]
            n838 = Unbundle By Name(w1552) -> ("Raw Sat"=w1549:cluster{dbl[], dbl[]}[], "Sqrt Sat"=w1550:cluster{dbl[], dbl[]}[], "Raw Lin"=w1548:cluster{dbl[], dbl[]}[], "Sqrt Lin"=w1551:cluster{dbl[], dbl[]}[], "Log Lin"=w1547:cluster{dbl[], dbl[]}[])  [unwired: 1 out]
            n839 = local write "Sqrt-Sat"(w1550) -> ()
            n840 = local write "Calc: STS"(w1561) -> ()
            n841 = local write "New: STS"(w1561) -> ()
            n842 = Array Subset(array=w1522, length (col)=1) -> (w1520:string[][])  [unwired: 3 in]
            n843 = Index Array(array=w1516, index=0) -> (element=w1527:i32)
            n844 = Decimate 1D Array(w1551) -> (w1576:cluster{dbl[], dbl[]}[])  [unwired: 1 out]
            n845 = local write "Calc: Trap Density-VT"(w1563) -> ()
            n846 = local write "New: VT-Sat"(w1560) -> ()
            n847 = local write "Calc: Trap Density-STS"(w1562) -> ()
            n848 = local write "New: Trap Density-STS"(w1562) -> ()
            n849 = local write "New: Trap Density-VT"(w1563) -> ()
            n850 = Reshape Array(w1520, w1527) -> (w1521:string[])
            n851 = local write "New: VT-Lin"(w1565) -> ()
            n852 = local write "Sqrt-Lin"(w1551) -> ()
            n853 = local write "New: Mobility-Sat"(w1567) -> ()
            n854 = local write "New: Mobility-Lin"(w1566) -> ()
            n855 = Decimate 1D Array(w1578) -> (w1637:cluster{dbl[], dbl[]}[])  [unwired: 1 out]
            n856 = Index Array(array=w1658, index=w1657) -> (element=w1643:i32)
            n857 = Decimate 1D Array(w1550) -> (w1647:cluster{dbl[], dbl[]}[])  [unwired: 1 out]
            n858 = Array To Cluster(array=w1576) -> (cluster=w1575:T11)
            n859 = Array Subset(array=w1659, index (row)=w1657, index (col)=w1657, length (col)=3) -> (w1660:string[][])  [unwired: 1 in]
            n860 = Search 1D Array(1D array=w1521, element="Vd") -> (index of element=w1523:i32)  [unwired: 1 in]
            n861 = local write "Raw- Sat"(w1549) -> ()
            n862 = local write "Raw- Lin"(w1548) -> ()
            n863 = local write "Log-Lin"(w1547) -> ()
            n864 = Array To Cluster(array=w1637) -> (cluster=w1635:T11)
            n865 = Array To Cluster(array=w1647) -> (cluster=w1649:T11)
            n866 = Reshape Array(w1660, w1643) -> (w1650:string[])
            n867 = Increment(x=w1523) -> (x+1=w1524:i32)
            n868 = Array Subset(array=w1522, index (row)=w1524) -> (w1526:string[][])  [unwired: 3 in]
            n869 = Subtract(x=w1643, y=20) -> (x-y=w1642:i32)
            n870 = Unbundle(w1575) -> ("[0]"=w1572:cluster{dbl[], dbl[]})  [unwired: 8 out]
            n871 = Fract/Exp String To Number(string=w1526, default (0 dbl)="default (0 dbl) 6") -> (number=w1534:ext[][])  [unwired: 2 in, 1 out]
            n872 = Delete From Array(array=w1534) -> (array with subset deleted=w1535:ext[][])  [unwired: 3 in, 1 out]
            n873 = property on="Sat-Trans Slider" class="Slide (strict)"("Scale.Maximum"=w1642) -> ()  [unwired: 2 in, 2 out]
            n874 = Delete From Array(array=w1535, index (col)=0 ("Deaktivierter Index (Spalte)")) -> (deleted portion=w1530:ext[], array with subset deleted=w1529:ext[][])  [unwired: 2 in]
            n875 = local read "Num Pts"() -> (w1569:dbl)
            n876 = Unbundle(w1635) -> ("[0]"=w1636:cluster{dbl[], dbl[]})  [unwired: 8 out]
            n877 = Unbundle(w1649) -> ("[0]"=w1648:cluster{dbl[], dbl[]})  [unwired: 8 out]
            n878 = Unbundle(w1572) -> (w1571:dbl[], w1570:dbl[])
            n879 = Search 1D Array(1D array=w1650, element="Index:") -> (index of element=w1654:i32)  [unwired: 1 in]
            n880 = Transpose 2D Array(2D array=w1529) -> (transposed array=w1528:ext[][])
            n881 = Increment(x=w1654) -> (x+1=w1655:i32)
            n882 = Unbundle(w1636) -> (w1634:dbl[], w1633:dbl[])
            n883 = Unbundle(w1648) -> (w1641:dbl[], w1640:dbl[])
            n884 = for {
              tunnel: w1530 -> [w1678]
              tunnel: w1528 -> [w1679] mode=indexing
              tunnel: [w1677] -> w1532 mode=indexing
              n885 = Bundle(w1678, w1679) -> (w1677:cluster{ext[], ext[]})  [unwired: 1 in]
            }
            n886 = Array Subset(array=w1571, index=w1568, length=w1569) -> (w1573:dbl[])
            n887 = Array Subset(array=w1570, index=w1568, length=w1569) -> (w1574:dbl[])
            n888 = local read "Image Folder"() -> (w1609:path)
            n889 = local write "Lin-Vg Array-Used"(w1573) -> ()
            n890 = Array Subset(array=w1634, index=w1579, length=w1580) -> (w1639:dbl[])
            n891 = Array Subset(array=w1633, index=w1579, length=w1580) -> (w1638:dbl[])
            n892 = Array Subset(array=w1641, index=w1581, length=w1583) -> (w1646:dbl[])
            n893 = Array Subset(array=w1640, index=w1581, length=w1583) -> (w1645:dbl[])
            n894 = local write "Lin Id-Used"(w1574) -> ()
            n895 = local write "Transport"(w1532) -> ()
            n896 = Index Array(array=w1650, index=w1655) -> (element=w1616:string)
            n897 = Array Size(array=w1532) -> (size(s)=w1533:i32)
            n898 = for {
              N: w1533 -> [_]
              i -> [w1676]
              n899 = local read "Transport Line Color"() -> (w1675:u32)
              n900 = local read "Ring"() -> (w1674:u16)
              n901 = property on="Transport" class="XYGraph (strict)"("Active Plot"=w1676, "Plot.Plot Color"=w1675, "Plot.Line Width"=w1674) -> ()  [unwired: 2 in, 2 out]
            }
            n902 = local write "Sat Vg Array-Used"(w1646) -> ()
            n903 = local write "Vg Array-Log-Used"(w1638) -> ()
            n904 = local write "Sat Id-Log-Used"(w1639) -> ()
            n905 = local write "Sat Id-Used"(w1645) -> ()
            n906 = local write "Index"(w1616) -> ()
            n907 = List Folder(path=w1609, error in=w1620) -> (filenames=w1652:string[], error out=w1619:errorcluster)  [unwired: 2 in, 2 out]
            n908 = Build Path(base path=w1609, name or relative path="ROI") -> (appended path=w1617:path)
            n909 = invoke on="Image Out" class="ImageControl" method="Clear ROI"(error in=w1619) -> (error out=w1623:errorcluster)  [unwired: 2 in, 2 out]
            n910 = while {
              tunnel: w1652 -> [w1694]
              tunnel: w1616 -> [w1692]
              tunnel: [w1691] -> w1651
              tunnel: w1643 -> [w1690]
              i -> [w1691]
              stop <- w1687 stop-if-true
              n911 = Index Array(array=w1694, index=w1691) -> (element=w1695:string)
              n912 = xnode "Match Regular Expression"("input string"=w1695, "regular expression"=w1692) -> ("whole match"=w1693:string)  [unwired: 4 in, 4 out]
              n913 = Equal?(x=w1693, y=w1692) -> (x = y?=w1689:bool)
              n914 = Equal?(x=w1690, y=w1691) -> (x = y?=w1688:bool)
              n915 = Or(x=w1689, y=w1688) -> (x .or. y?=w1687:bool)
            }
            n916 = Build Path(base path=w1617, name or relative path=w1616) -> (appended path=w1615:path)
            n917 = call <vilib>:"Check if File or Folder Exists.vi"("error in (no error)"=w1623, "path"=w1615) -> ("file or folder exists?"=w1621:bool, "dup path"=w1622:path)  [unwired: 7 in, 1 out]
            n918 = case shown="True" w1621 {
              tunnel: w1622 -> [_ w1682]
              frame False {
              }
              frame True {
                n919 = Read from Text File(file (use dialog)=w1682) -> (text=w1686:string)  [unwired: 3 in, 3 out]
                n920 = property on="Image Out" class="ImageControl"() -> ("ROI"=w1683:T12)  [unwired: 2 in, 2 out]
                n921 = Unflatten From String(type=w1683, binary string=w1686) -> (value=w1684:T12, error out=w1685:errorcluster)  [unwired: 3 in, 1 out]
                n922 = property on="Image Out" class="ImageControl"(error in=w1685, "ROI"=w1684) -> ()  [unwired: 1 in, 2 out]
              }
            }
            n923 = Index Array(array=w1652, index=w1651) -> (element=w1625:string)
            n924 = local write "Image Name"(w1625) -> ()
            n925 = Empty String/Path?(string/path=w1625) -> (empty?=w1632:bool)
            n926 = Build Path(base path=w1609, name or relative path=w1625) -> (appended path=w1624:path)
            n927 = local read "No Image File"() -> (w1631:path)
            n928 = Select(t=w1631, s=w1632, f=w1624) -> (s? t:f=w1626:path)
            n929 = call <vilib>:"Get File Extension.vi"("file"=w1626) -> ("lowercase file extension"=w1628:string)  [unwired: 7 in, 3 out]
            n930 = local write "Image File"(w1626) -> ()
            n931 = local write "String"(w1628) -> ()
            n932 = Search 1D Array(1D array=string[] ["bmp", "jpeg", "png", "jpg", "gif"], element=w1628) -> (index of element=w1627:i32)  [unwired: 1 in]
            n933 = call "Vision Acquisition5"("Image Path"=w1626) -> ("Image Out"=w1630:T2)  [unwired: 25 in, 1 out]
            n934 = Less Than 0?(x=w1627) -> ()  [unwired: 1 out]
            n935 = local write "Image Out"(w1630) -> ()
            n936 = local write "Image Out 2"(w1630) -> ()
          }
          event "Save Changes? 3": Mouse Down {
            n937 = event-data() -> ()  [unwired: 1 in, 7 out]
            n938 = local read "Image Folder"() -> (w1811:path)
            n939 = Build Path(base path=w1811, name or relative path="ROI") -> (appended path=w1818:path)
            n940 = call <vilib>:"Check if File or Folder Exists.vi"("path"=w1818) -> ("file or folder exists?"=w1820:bool, "dup path"=w1817:path)  [unwired: 8 in, 1 out]
            n941 = case shown="False" w1820 {
              tunnel: w1817 -> [w1822 w1823]
              tunnel: [w1821 w1823] -> w1812
              frame False {
                n942 = Create Folder(path (use dialog)=w1822) -> (created path=w1821:path)  [unwired: 2 in, 2 out]
              }
              frame True {
              }
            }
            n943 = local read "Index"() -> (w1814:string)
            n944 = property on="Image Out" class="ImageControl"() -> ("ROI"=w1816:T12)  [unwired: 2 in, 2 out]
            n945 = Build Path(base path=w1812, name or relative path=w1814) -> (appended path=w1813:path)
            n946 = Flatten To String(anything=w1816) -> (data string=w1815:string)  [unwired: 3 in, 2 out]
            n947 = Write to Text File(file (use dialog)=w1813, text=w1815) -> ()  [unwired: 2 in, 3 out]
          }
          event "Next Sqrt Sat": Mouse Down {
            n948 = event-data() -> ()  [unwired: 1 in, 5 out]
            n949 = local read "Sqrt-Sat"() -> (w1836:cluster{dbl[], dbl[]}[])
            n950 = Decimate 1D Array(w1836) -> (w1832:cluster{dbl[], dbl[]}[], w1831:cluster{dbl[], dbl[]}[])
            n951 = Array To Cluster(array=w1832) -> (cluster=w1842:T11)
            n952 = Unbundle(w1842) -> ("[0]"=w1841:cluster{dbl[], dbl[]})  [unwired: 8 out]
            n953 = local read "MobVi Index"() -> (w1838:dbl)
            n954 = local read "Num Pts"() -> (w1837:dbl)
            n955 = Unbundle(w1841) -> (w1840:dbl[], w1839:dbl[])
            n956 = Increment(x=w1838) -> (x+1=w1833:dbl)
            n957 = local read "New: Dielectric"() -> (w1827:dbl)
            n958 = local read "New: Length"() -> (w1826:dbl)
            n959 = local read "New: Width"() -> (w1825:dbl)
            n960 = local write "MobVi Index"(w1833) -> ()
            n961 = Array Subset(array=w1840, index=w1833, length=w1837) -> (w1829:dbl[])
            n962 = Array Subset(array=w1839, index=w1833, length=w1837) -> (w1828:dbl[])
            n963 = local write "Sat Vg Array-Used"(w1829) -> ()
            n964 = local write "Sat Id-Used"(w1828) -> ()
            n965 = call "Mobility-Vt-Used Pts_Saturation.vi"("Width"=w1825, "Length"=w1826, "Dielectric (d)"=w1827, "Sat Id Used"=w1828, "Vg Used"=w1829) -> ("Vt"=w1824:dbl, "Mobility"=w1830:dbl)  [unwired: 4 in, 1 out]
            n966 = Bundle(w1829, w1828) -> (w1835:cluster{dbl[], dbl[]})  [unwired: 1 in]
            n967 = Build Array (concatenate)(w1832, w1831, w1835) -> (w1834:cluster{dbl[], dbl[]}[])
            n968 = local write "New: Mobility-Sat"(w1830) -> ()
            n969 = local write "New: VT-Sat"(w1824) -> ()
            n970 = local write "Sqrt-Sat"(w1834) -> ()
          }
          event "Next Log Sat": Mouse Down {
            n971 = event-data() -> ()  [unwired: 1 in, 7 out]
            n972 = local read "Sat-Log"() -> (w1851:cluster{dbl[], dbl[]}[])
            n973 = Decimate 1D Array(w1851) -> (w1847:cluster{dbl[], dbl[]}[], w1846:cluster{dbl[], dbl[]}[])
            n974 = Array To Cluster(array=w1847) -> (cluster=w1857:T11)
            n975 = local read "Index 2"() -> (w1853:dbl)
            n976 = local read "NumPoints Log"() -> (w1852:dbl)
            n977 = Unbundle(w1857) -> ("[0]"=w1856:cluster{dbl[], dbl[]})  [unwired: 8 out]
            n978 = Unbundle(w1856) -> (w1855:dbl[], w1854:dbl[])
            n979 = Increment(x=w1853) -> (x+1=w1848:dbl)
            n980 = local write "Index 2"(w1848) -> ()
            n981 = Array Subset(array=w1854, index=w1848, length=w1852) -> (w1843:dbl[])
            n982 = Array Subset(array=w1855, index=w1848, length=w1852) -> (w1844:dbl[])
            n983 = call "STS-Used.vi"("Id Used"=w1844, "Vg-Used"=w1843) -> ("STS"=w1845:dbl)  [unwired: 9 in]
            n984 = Bundle(w1844, w1843) -> (w1850:cluster{dbl[], dbl[]})  [unwired: 1 in]
            n985 = local write "Vg Array-Log-Used"(w1843) -> ()
            n986 = local write "Sat Id-Log-Used"(w1844) -> ()
            n987 = local write "New: STS"(w1845) -> ()
            n988 = Build Array (concatenate)(w1847, w1846, w1850) -> (w1849:cluster{dbl[], dbl[]}[])
            n989 = local write "Sat-Log"(w1849) -> ()
          }
          event "Previous Log Sat": Mouse Down {
            n990 = event-data() -> ()  [unwired: 1 in, 7 out]
            n991 = local read "Sat-Log"() -> (w1867:cluster{dbl[], dbl[]}[])
            n992 = Decimate 1D Array(w1867) -> (w1864:cluster{dbl[], dbl[]}[], w1863:cluster{dbl[], dbl[]}[])
            n993 = Array To Cluster(array=w1864) -> (cluster=w1872:T11)
            n994 = local read "Index 2"() -> (w1860:dbl)
            n995 = local read "NumPoints Log"() -> (w1868:dbl)
            n996 = Unbundle(w1872) -> ("[0]"=w1871:cluster{dbl[], dbl[]})  [unwired: 8 out]
            n997 = Unbundle(w1871) -> (w1870:dbl[], w1869:dbl[])
            n998 = Decrement(x=w1860) -> (x-1=w1861:dbl)
            n999 = local write "Index 2"(w1861) -> ()
            n1000 = Array Subset(array=w1870, index=w1861, length=w1868) -> (w1858:dbl[])
            n1001 = Array Subset(array=w1869, index=w1861, length=w1868) -> (w1859:dbl[])
            n1002 = local write "Sat Id-Log-Used"(w1858) -> ()
            n1003 = Bundle(w1858, w1859) -> (w1866:cluster{dbl[], dbl[]})  [unwired: 1 in]
            n1004 = call "STS-Used.vi"("Id Used"=w1858, "Vg-Used"=w1859) -> ("STS"=w1862:dbl)  [unwired: 9 in]
            n1005 = local write "Vg Array-Log-Used"(w1859) -> ()
            n1006 = Build Array (concatenate)(w1864, w1863, w1866) -> (w1865:cluster{dbl[], dbl[]}[])
            n1007 = local write "New: STS"(w1862) -> ()
            n1008 = local write "Sat-Log"(w1865) -> ()
          }
          event "Previous Sqrt Sat": Mouse Down {
            n1009 = event-data() -> ()  [unwired: 1 in, 5 out]
            n1010 = local read "Sqrt-Sat"() -> (w1886:cluster{dbl[], dbl[]}[])
            n1011 = Decimate 1D Array(w1886) -> (w1883:cluster{dbl[], dbl[]}[], w1882:cluster{dbl[], dbl[]}[])
            n1012 = Array To Cluster(array=w1883) -> (cluster=w1891:T11)
            n1013 = local read "MobVi Index"() -> (w1881:dbl)
            n1014 = Unbundle(w1891) -> ("[0]"=w1890:cluster{dbl[], dbl[]})  [unwired: 8 out]
            n1015 = local read "Num Pts"() -> (w1887:dbl)
            n1016 = Unbundle(w1890) -> (w1889:dbl[], w1888:dbl[])
            n1017 = Decrement(x=w1881) -> (x-1=w1880:dbl)
            n1018 = local read "New: Dielectric"() -> (w1874:dbl)
            n1019 = local read "New: Length"() -> (w1875:dbl)
            n1020 = local read "New: Width"() -> (w1876:dbl)
            n1021 = local write "MobVi Index"(w1880) -> ()
            n1022 = Array Subset(array=w1889, index=w1880, length=w1887) -> (w1879:dbl[])
            n1023 = Array Subset(array=w1888, index=w1880, length=w1887) -> (w1878:dbl[])
            n1024 = local write "Sat Vg Array-Used"(w1879) -> ()
            n1025 = local write "Sat Id-Used"(w1878) -> ()
            n1026 = call "Mobility-Vt-Used Pts_Linear.vi"("Width"=w1876, "Length"=w1875, "Dielectric (d)"=w1874, "Sat Id Used"=w1878, "Vg Used"=w1879) -> ("Vt"=w1873:dbl, "Mobility"=w1877:dbl)  [unwired: 4 in, 1 out]
            n1027 = Bundle(w1879, w1878) -> (w1885:cluster{dbl[], dbl[]})  [unwired: 1 in]
            n1028 = local write "New: VT-Sat"(w1873) -> ()
            n1029 = Build Array (concatenate)(w1883, w1882, w1885) -> (w1884:cluster{dbl[], dbl[]}[])
            n1030 = local write "New: Mobility-Sat"(w1877) -> ()
            n1031 = local write "Sqrt-Sat"(w1884) -> ()
          }
          event "Sat-Trans Slider": Value Change {
            n1032 = event-data() -> ()  [unwired: 1 in, 5 out]
            n1033 = local read "Sqrt-Sat"() -> (w1904:cluster{dbl[], dbl[]}[])
            n1034 = Decimate 1D Array(w1904) -> (w1901:cluster{dbl[], dbl[]}[], w1900:cluster{dbl[], dbl[]}[])
            n1035 = Array To Cluster(array=w1901) -> (cluster=w1909:T11)
            n1036 = Unbundle(w1909) -> ("[0]"=w1908:cluster{dbl[], dbl[]})  [unwired: 8 out]
            n1037 = local read "Sat-Trans Slider"() -> (w1893:dbl)
            n1038 = local read "Num Pts"() -> (w1905:dbl)
            n1039 = Unbundle(w1908) -> (w1907:dbl[], w1906:dbl[])
            n1040 = local read "New: Dielectric"() -> (w1894:dbl)
            n1041 = local read "New: Length"() -> (w1895:dbl)
            n1042 = local read "New: Width"() -> (w1896:dbl)
            n1043 = local write "MobVi Index"(w1893) -> ()
            n1044 = Array Subset(array=w1907, index=w1893, length=w1905) -> (w1899:dbl[])
            n1045 = Array Subset(array=w1906, index=w1893, length=w1905) -> (w1898:dbl[])
            n1046 = local write "Sat Vg Array-Used"(w1899) -> ()
            n1047 = local write "Sat Id-Used"(w1898) -> ()
            n1048 = call "Mobility-Vt-Used Pts_Linear.vi"("Width"=w1896, "Length"=w1895, "Dielectric (d)"=w1894, "Sat Id Used"=w1898, "Vg Used"=w1899) -> ("Vt"=w1892:dbl, "Mobility"=w1897:dbl)  [unwired: 4 in, 1 out]
            n1049 = Bundle(w1899, w1898) -> (w1903:cluster{dbl[], dbl[]})  [unwired: 1 in]
            n1050 = local write "New: VT-Sat"(w1892) -> ()
            n1051 = Build Array (concatenate)(w1901, w1900, w1903) -> (w1902:cluster{dbl[], dbl[]}[])
            n1052 = local write "New: Mobility-Sat"(w1897) -> ()
            n1053 = local write "Sqrt-Sat"(w1902) -> ()
          }
          event "Sat-Log Slider": Value Change {
            n1054 = event-data() -> ()  [unwired: 1 in, 5 out]
            n1055 = local read "Sat-Log"() -> (w1918:cluster{dbl[], dbl[]}[])
            n1056 = Decimate 1D Array(w1918) -> (w1915:cluster{dbl[], dbl[]}[], w1914:cluster{dbl[], dbl[]}[])
            n1057 = Array To Cluster(array=w1915) -> (cluster=w1923:T11)
            n1058 = Unbundle(w1923) -> ("[0]"=w1922:cluster{dbl[], dbl[]})  [unwired: 8 out]
            n1059 = local read "NumPoints Log"() -> (w1919:dbl)
            n1060 = local read "Sat-Log Slider"() -> (w1913:dbl)
            n1061 = Unbundle(w1922) -> (w1921:dbl[], w1920:dbl[])
            n1062 = local write "Index 2"(w1913) -> ()
            n1063 = Array Subset(array=w1921, index=w1913, length=w1919) -> (w1911:dbl[])
            n1064 = Array Subset(array=w1920, index=w1913, length=w1919) -> (w1910:dbl[])
            n1065 = local write "Vg Array-Log-Used"(w1910) -> ()
            n1066 = local write "Sat Id-Log-Used"(w1911) -> ()
            n1067 = call "STS-Used.vi"("Id Used"=w1911, "Vg-Used"=w1910) -> ("STS"=w1912:dbl)  [unwired: 9 in]
            n1068 = Bundle(w1911, w1910) -> (w1917:cluster{dbl[], dbl[]})  [unwired: 1 in]
            n1069 = local write "New: STS"(w1912) -> ()
            n1070 = Build Array (concatenate)(w1915, w1914, w1917) -> (w1916:cluster{dbl[], dbl[]}[])
            n1071 = local write "Sat-Log"(w1916) -> ()
          }
          event "Save Changes?": Mouse Down {
            n1072 = event-data() -> ()  [unwired: 1 in, 5 out]
            n1073 = flat-sequence {
              tunnel: [w1930] -> w1928
              tunnel: [w1938] -> w1927
              tunnel: [w1931] -> w1926
              tunnel: w1928 -> [w2470]
              tunnel: w1927 -> [w2467]
              tunnel: [w2468] -> w1925
              tunnel: w1926 -> [w2468]
              tunnel: [w2467] -> w1924
              tunnel: w1925 -> [w2475]
              tunnel: w1924 -> [w2474]
              frame #0 {
                n1074 = Wait (ms)(milliseconds to wait=1) -> ()  [unwired: 1 out]
              }
              frame #1 {
                n1075 = local read "Transfer File"() -> (w1930:path)
                n1076 = local read "New: Temp"() -> (w1932:dbl)
                n1077 = local read "New: Length"() -> (w1936:dbl)
                n1078 = local read "New: Width"() -> (w1934:dbl)
                n1079 = To Single Precision Float(number=w1932) -> (single precision float=w1933:sgl)
                n1080 = Number To Decimal String(number=w1933) -> (decimal integer string=w1941:string)  [unwired: 1 in]
                n1081 = To Single Precision Float(number=w1934) -> (single precision float=w1935:sgl)
                n1082 = To Single Precision Float(number=w1936) -> (single precision float=w1937:sgl)
                n1083 = local read "Index"() -> (w1946:string)
                n1084 = Strip Path(path=w1930) -> (stripped path=w1951:path)  [unwired: 1 out]
                n1085 = Number To Decimal String(number=w1937) -> (decimal integer string=w1944:string)  [unwired: 1 in]
                n1086 = Number To Decimal String(number=w1935) -> (decimal integer string=w1945:string)  [unwired: 1 in]
                n1087 = Concatenate Strings("_", w1941, "K") -> (w1939:string)
                n1088 = call "Build Text"("Temp"=w1939, "Index"=w1946, "Length"=w1944, "Width"=w1945) -> ("Result"=w1947:string)  [unwired: 10 in, 1 out]
                n1089 = flat-sequence {
                  tunnel: [w2424] -> w1943
                  tunnel: w1943 -> [w2441]
                  frame #0 {
                    # "Makes Empty File for Transformer Data"
                    n1090 = local read "Transfer Folder"() -> (w2413:path)
                    n1091 = Build Path(base path=w2413, name or relative path="Stats") -> (appended path=w2415:path)
                    n1092 = call <vilib>:"Check if File or Folder Exists.vi"("path"=w2415) -> ("file or folder exists?"=w2416:bool, "dup path"=w2417:path)  [unwired: 8 in, 1 out]
                    n1093 = case shown="False" w2416 {
                      tunnel: [w2421 w2423] -> w2418
                      tunnel: w2417 -> [w2422 w2423]
                      frame False {
                        n1094 = Create Folder(path (use dialog)=w2422) -> (created path=w2421:path)  [unwired: 2 in, 2 out]
                      }
                      frame True {
                      }
                    }
                    n1095 = Build Path(base path=w2418, name or relative path="Tranformer Data.txt") -> (appended path=w2420:path)
                    n1096 = call-poly <vilib>:"Write To Spreadsheet File.vi"("append to file? (new file:F)"=TRUE, "file path (dialog if empty)"=w2420) -> ()  [unwired: 6 in, 1 out]
                  }
                  frame #1 {
                    # "Adds Headers if they don't exist"
                    n1097 = local read "Transfer Folder"() -> (w2430:path)
                    n1098 = Concatenate Strings("Stats\\", "Tranformer Data.txt") -> (w2431:string)
                    n1099 = Build Path(base path=w2430, name or relative path=w2431) -> (appended path=w2424:path)
                    n1100 = call-poly <vilib>:"Read From Spreadsheet File.vi"("file path (dialog if empty)"=w2424) -> ("first row"=w2429:string[])  [unwired: 6 in, 4 out]
                    n1101 = Search 1D Array(1D array=w2429, element="DeviceID") -> (index of element=w2427:i32)  [unwired: 1 in]
                    n1102 = Equal?(x=w2427, y=0) -> (x = y?=w2425:bool)
                    n1103 = case shown="False" w2425 {
                      tunnel: w2424 -> [w2435 _]
                      frame False {
                        n1104 = local read "Transformer \nHeaders"() -> (w2434:string[])
                        n1105 = call-poly <vilib>:"Write To Spreadsheet File.vi"("1D data"=w2434, "file path (dialog if empty)"=w2435) -> ()  [unwired: 6 in, 1 out]
                      }
                      frame True {
                      }
                    }
                  }
                  frame #2 {
                    # "Adds current device if it doesn't exist"
                    n1106 = local read "Current \nRecord"() -> (w2440:string[])
                    n1107 = Index Array(array=w2440, index=0) -> (element=w2439:string)
                    n1108 = local read "Transfer Folder"() -> (w2443:path)
                    n1109 = Concatenate Strings("Stats\\", "Tranformer Data.txt") -> (w2444:string)
                    n1110 = local write "Current Device ID"(w2439) -> ()
                    n1111 = local read "Current Device ID"() -> (w2449:string)
                    n1112 = Build Path(base path=w2443, name or relative path=w2444) -> (appended path=w2442:path)
                    n1113 = call-poly <vilib>:"Read From Spreadsheet File.vi"("file path (dialog if empty)"=w2442) -> ("all rows"=w2436:string[][])  [unwired: 6 in, 4 out]
                    n1114 = Index Array(array=w2436, index (col)=0) -> (element=w2437:string[])  [unwired: 1 in]
                    n1115 = Search 1D Array(1D array=w2437, element=w2449) -> (index of element=w2438:i32)  [unwired: 1 in]
                    n1116 = Equal?(x=w2438, y=-1) -> (x = y?=w2451:bool)
                    n1117 = case shown="False" w2451 {
                      tunnel: w2441 -> [w2454 w2465]
                      tunnel: w2438 -> [w2457 _]
                      tunnel: w2436 -> [w2458 _]
                      frame False {
                        n1118 = local read "Current \nRecord"() -> (w2456:string[])
                        n1119 = Replace Array Subset(array=w2458, new element=w2456, index (row)=w2457) -> (w2455:string[][])  [unwired: 1 in]
                        n1120 = flat-sequence {
                          tunnel: w2454 -> [w2459]
                          tunnel: w2455 -> [w2460]
                          tunnel: [w2460] -> w2453
                          tunnel: [w2459] -> w2452
                          tunnel: w2453 -> [w2462]
                          tunnel: w2452 -> [w2461]
                          frame #0 {
                            n1121 = Delete(path (use dialog)=w2459) -> ()  [unwired: 4 in, 3 out]
                          }
                          frame #1 {
                            n1122 = call-poly <vilib>:"Write To Spreadsheet File.vi"("append to file? (new file:F)"=TRUE, "2D data"=w2462, "file path (dialog if empty)"=w2461) -> ()  [unwired: 5 in, 1 out]
                          }
                        }
                      }
                      frame True {
                        n1123 = local read "Current \nRecord"() -> (w2464:string[])
                        n1124 = call-poly <vilib>:"Write To Spreadsheet File.vi"("append to file? (new file:F)"=TRUE, "1D data"=w2464, "file path (dialog if empty)"=w2465) -> ()  [unwired: 5 in, 1 out]
                      }
                    }
                  }
                }
                n1125 = Path To String(path=w1951) -> (string=w1949:string)
                n1126 = stacked-sequence {
                  tunnel: [_ _ _ _ _ _ _ _ _ _ _ _ _ w2384] -> w1931
                  tunnel: w1930 -> [w1953 _ _ _ _ _ _ _ _ _ _ _ _ _]
                  frame #0 {
                    n1127 = call-poly <vilib>:"Read From Spreadsheet File.vi"("file path (dialog if empty)"=w1953) -> ("all rows"=w1952:string[][])  [unwired: 6 in, 4 out]
                    n1128 = Array Size(array=w1952) -> (size(s)=w1957:i32[])
                    n1129 = Array Subset(array=w1952, index (row)=0, index (col)=0, length (col)=3) -> (w1961:string[][])  [unwired: 1 in]
                    n1130 = Index Array(array=w1957, index=0) -> (element=w1955:i32)
                    n1131 = Reshape Array(w1961, w1955) -> (w1954:string[])
                    n1132 = Search 1D Array(1D array=w1954, element="Dielectric (nm):") -> (index of element=w1964:i32)  [unwired: 1 in]
                    n1133 = Equal?(x=w1964, y=-1) -> (x = y?=w1963:bool)
                    n1134 = case shown="False" w1963 {
                      tunnel: w1952 -> [w1972 w1976]
                      tunnel: w1964 -> [w1968 _]
                      tunnel: [w1967 w1976] -> w1962
                      frame False {
                        n1135 = local read "New: Dielectric"() -> (w1974:dbl)
                        n1136 = Number To Fractional String(number=w1974) -> (F-format string=w1969:string)  [unwired: 3 in]
                        n1137 = Divide(x=w1968, y=3) -> (x/y=w1971:dbl)
                        n1138 = To Word Integer(number=w1971) -> (16bit integer=w1970:i16)
                        n1139 = Replace Array Subset(array=w1972, new element=w1969, index (row)=w1970, index (col)=1) -> (w1967:string[][])
                      }
                      frame True {
                      }
                    }
                    n1140 = local write "Save1 Array"(w1962) -> ()
                  }
                  frame #1 {
                    n1141 = local read "Save1 Array"() -> (w1978:string[][])
                    n1142 = Array Size(array=w1978) -> (size(s)=w1981:i32[])
                    n1143 = Array Subset(array=w1978, index (row)=0, index (col)=0, length (col)=3) -> (w1985:string[][])  [unwired: 1 in]
                    n1144 = Index Array(array=w1981, index=0) -> (element=w1979:i32)
                    n1145 = Reshape Array(w1985, w1979) -> (w1977:string[])
                    n1146 = Search 1D Array(1D array=w1977, element="Comments:") -> (index of element=w1988:i32)  [unwired: 1 in]
                    n1147 = Equal?(x=w1988, y=-1) -> (x = y?=w1987:bool)
                    n1148 = case shown="False" w1987 {
                      tunnel: w1978 -> [w1996 w1999]
                      tunnel: w1988 -> [w1993 _]
                      tunnel: [w1992 w1999] -> w1986
                      frame False {
                        n1149 = local read "Comments:"() -> (w1991:string)
                        n1150 = Divide(x=w1993, y=3) -> (x/y=w1995:dbl)
                        n1151 = To Word Integer(number=w1995) -> (16bit integer=w1994:i16)
                        n1152 = Replace Array Subset(array=w1996, new element=w1991, index (row)=w1994, index (col)=1) -> (w1992:string[][])
                      }
                      frame True {
                      }
                    }
                    n1153 = local write "Save1 Array"(w1986) -> ()
                  }
                  frame #2 {
                    n1154 = local read "Save1 Array"() -> (w2001:string[][])
                    n1155 = Array Size(array=w2001) -> (size(s)=w2004:i32[])
                    n1156 = Array Subset(array=w2001, index (row)=0, index (col)=0, length (col)=3) -> (w2008:string[][])  [unwired: 1 in]
                    n1157 = Index Array(array=w2004, index=0) -> (element=w2002:i32)
                    n1158 = Reshape Array(w2008, w2002) -> (w2000:string[])
                    n1159 = Search 1D Array(1D array=w2000, element="Length (um):") -> (index of element=w2011:i32)  [unwired: 1 in]
                    n1160 = Equal?(x=w2011, y=-1) -> (x = y?=w2010:bool)
                    n1161 = case shown="False" w2010 {
                      tunnel: w2001 -> [w2021 w2024]
                      tunnel: w2011 -> [w2018 _]
                      tunnel: [w2017 w2024] -> w2009
                      frame False {
                        n1162 = local read "New: Length"() -> (w2014:dbl)
                        n1163 = Divide(x=w2018, y=3) -> (x/y=w2020:dbl)
                        n1164 = Format Value(format string="%#g", value (0)=w2014) -> (output string=w2015:string)  [unwired: 1 in]
                        n1165 = To Word Integer(number=w2020) -> (16bit integer=w2019:i16)
                        n1166 = Replace Array Subset(array=w2021, new element=w2015, index (row)=w2019, index (col)=1) -> (w2017:string[][])
                      }
                      frame True {
                      }
                    }
                    n1167 = local write "Save1 Array"(w2009) -> ()
                  }
                  frame #3 {
                    n1168 = local read "Save1 Array"() -> (w2026:string[][])
                    n1169 = Array Size(array=w2026) -> (size(s)=w2031:i32[])
                    n1170 = Array Subset(array=w2026, index (row)=0, index (col)=0, length (col)=3) -> (w2027:string[][])  [unwired: 1 in]
                    n1171 = Index Array(array=w2031, index=0) -> (element=w2033:i32)
                    n1172 = Reshape Array(w2027, w2033) -> (w2025:string[])
                    n1173 = Search 1D Array(1D array=w2025, element="Width (um):") -> (index of element=w2036:i32)  [unwired: 1 in]
                    n1174 = Equal?(x=w2036, y=-1) -> (x = y?=w2035:bool)
                    n1175 = case shown="False" w2035 {
                      tunnel: w2036 -> [w2044 _]
                      tunnel: w2026 -> [w2043 w2049]
                      tunnel: [w2042 w2049] -> w2034
                      frame False {
                        n1176 = local read "New: Width"() -> (w2039:dbl)
                        n1177 = Divide(x=w2044, y=3) -> (x/y=w2046:dbl)
                        n1178 = To Word Integer(number=w2046) -> (16bit integer=w2045:i16)
                        n1179 = Format Value(format string="%#g", value (0)=w2039) -> (output string=w2040:string)  [unwired: 1 in]
                        n1180 = Replace Array Subset(array=w2043, new element=w2040, index (row)=w2045, index (col)=1) -> (w2042:string[][])
                      }
                      frame True {
                      }
                    }
                    n1181 = local write "Save1 Array"(w2034) -> ()
                  }
                  frame #4 {
                    w2059 = "Sample Temp (K):"
                    n1182 = local read "Save1 Array"() -> (w2051:string[][])
                    n1183 = Array Size(array=w2051) -> (size(s)=w2056:i32[])
                    n1184 = Array Subset(array=w2051, index (row)=0, index (col)=0, length (col)=3) -> (w2052:string[][])  [unwired: 1 in]
                    n1185 = Index Array(array=w2056, index=0) -> (element=w2058:i32)
                    n1186 = Reshape Array(w2052, w2058) -> (w2050:string[])
                    n1187 = Search 1D Array(1D array=w2050, element=w2059) -> (index of element=w2062:i32)  [unwired: 1 in]
                    n1188 = Equal?(x=w2062, y=-1) -> (x = y?=w2061:bool)
                    n1189 = case shown="True" w2061 {
                      tunnel: w2051 -> [w2071 w2085]
                      tunnel: w2062 -> [w2068 _]
                      tunnel: [w2067 w2084] -> w2060
                      tunnel: w2050 -> [_ w2087]
                      tunnel: w2059 -> [_ w2074]
                      frame False {
                        n1190 = local read "New: Temp"() -> (w2065:dbl)
                        n1191 = Divide(x=w2068, y=3) -> (x/y=w2070:dbl)
                        n1192 = Format Value(format string="%#g", value (0)=w2065) -> (output string=w2064:string)  [unwired: 1 in]
                        n1193 = To Word Integer(number=w2070) -> (16bit integer=w2069:i16)
                        n1194 = Replace Array Subset(array=w2071, new element=w2064, index (row)=w2069, index (col)=1) -> (w2067:string[][])
                      }
                      frame True {
                        n1195 = local read "New: Temp"() -> (w2076:dbl)
                        n1196 = Search 1D Array(1D array=w2087, element="Width (um):") -> (index of element=w2081:i32)  [unwired: 1 in]
                        n1197 = Divide(x=w2081, y=3) -> (x/y=w2082:dbl)
                        n1198 = To Word Integer(number=w2082) -> (16bit integer=w2080:i16)
                        n1199 = Format Value(format string="%#g", value (0)=w2076) -> (output string=w2075:string)  [unwired: 1 in]
                        n1200 = Build Array(w2074, w2075) -> (w2078:string[])
                        n1201 = Increment(x=w2080) -> (x+1=w2079:i16)
                        n1202 = Insert Into Array(array=w2085, index (row)=w2079, new element=w2078) -> (w2084:string[][])  [unwired: 1 in]
                      }
                    }
                    n1203 = local write "Save1 Array"(w2060) -> ()
                  }
                  frame #5 {
                    w2097 = "Mobility-Sat (cm^2/Vs):"
                    n1204 = local read "Save1 Array"() -> (w2089:string[][])
                    n1205 = Array Size(array=w2089) -> (size(s)=w2094:i32[])
                    n1206 = Array Subset(array=w2089, index (row)=0, index (col)=0, length (col)=3) -> (w2090:string[][])  [unwired: 1 in]
                    n1207 = Index Array(array=w2094, index=0) -> (element=w2096:i32)
                    n1208 = Reshape Array(w2090, w2096) -> (w2088:string[])
                    n1209 = Search 1D Array(1D array=w2088, element=w2097) -> (index of element=w2100:i32)  [unwired: 1 in]
                    n1210 = Equal?(x=w2100, y=-1) -> (x = y?=w2099:bool)
                    n1211 = case shown="True" w2099 {
                      tunnel: w2089 -> [w2109 w2117]
                      tunnel: w2100 -> [w2106 _]
                      tunnel: [w2105 w2116] -> w2098
                      tunnel: w2088 -> [_ w2114]
                      tunnel: w2097 -> [_ w2112]
                      frame False {
                        n1212 = local read "New: Mobility-Sat"() -> (w2102:dbl)
                        n1213 = Divide(x=w2106, y=3) -> (x/y=w2108:dbl)
                        n1214 = To Word Integer(number=w2108) -> (16bit integer=w2107:i16)
                        n1215 = Format Value(format string="%#g", value (0)=w2102) -> (output string=w2103:string)  [unwired: 1 in]
                        n1216 = Replace Array Subset(array=w2109, new element=w2103, index (row)=w2107, index (col)=1) -> (w2105:string[][])
                      }
                      frame True {
                        n1217 = local read "New: Mobility-Sat"() -> (w2118:dbl)
                        n1218 = Search 1D Array(1D array=w2114, element="Mobility (cm^2/Vs):") -> (index of element=w2121:i32)  [unwired: 1 in]
                        n1219 = Divide(x=w2121, y=3) -> (x/y=w2122:dbl)
                        n1220 = To Word Integer(number=w2122) -> (16bit integer=w2113:i16)
                        n1221 = Format Value(format string="%#g", value (0)=w2118) -> (output string=w2115:string)  [unwired: 1 in]
                        n1222 = Build Array(w2112, w2115) -> (w2120:string[])
                        n1223 = Replace Array Subset(array=w2117, new element=w2120, index (row)=w2113) -> (w2116:string[][])  [unwired: 1 in]
                      }
                    }
                    n1224 = local write "Save1 Array"(w2098) -> ()
                  }
                  frame #6 {
                    w2134 = "Mobility-Lin (cm^2/Vs):"
                    n1225 = local read "Save1 Array"() -> (w2125:string[][])
                    n1226 = Array Size(array=w2125) -> (size(s)=w2131:i32[])
                    n1227 = Array Subset(array=w2125, index (row)=0, index (col)=0, length (col)=3) -> (w2127:string[][])  [unwired: 1 in]
                    n1228 = Index Array(array=w2131, index=0) -> (element=w2133:i32)
                    n1229 = Reshape Array(w2127, w2133) -> (w2126:string[])
                    n1230 = Search 1D Array(1D array=w2126, element=w2134) -> (index of element=w2137:i32)  [unwired: 1 in]
                    n1231 = Equal?(x=w2137, y=-1) -> (x = y?=w2136:bool)
                    n1232 = case shown="True" w2136 {
                      tunnel: w2125 -> [w2146 w2152]
                      tunnel: w2137 -> [w2143 _]
                      tunnel: [w2142 w2151] -> w2135
                      tunnel: w2126 -> [_ w2150]
                      tunnel: w2134 -> [_ w2149]
                      frame False {
                        n1233 = local read "Calc: Mobility-Lin"() -> (w2139:dbl)
                        n1234 = Divide(x=w2143, y=3) -> (x/y=w2145:dbl)
                        n1235 = To Word Integer(number=w2145) -> (16bit integer=w2144:i16)
                        n1236 = Format Value(format string="%#g", value (0)=w2139) -> (output string=w2140:string)  [unwired: 1 in]
                        n1237 = Replace Array Subset(array=w2146, new element=w2140, index (row)=w2144, index (col)=1) -> (w2142:string[][])
                      }
                      frame True {
                        n1238 = local read "Calc: Mobility-Lin"() -> (w2153:dbl)
                        n1239 = Search 1D Array(1D array=w2150, element="Mobility-Sat (cm^2/Vs):") -> (index of element=w2158:i32)  [unwired: 1 in]
                        n1240 = Divide(x=w2158, y=3) -> (x/y=w2159:dbl)
                        n1241 = To Word Integer(number=w2159) -> (16bit integer=w2157:i16)
                        n1242 = Format Value(format string="%#g", value (0)=w2153) -> (output string=w2162:string)  [unwired: 1 in]
                        n1243 = Build Array(w2149, w2162) -> (w2155:string[])
                        n1244 = Increment(x=w2157) -> (x+1=w2156:i16)
                        n1245 = Insert Into Array(array=w2152, index (row)=w2156, new element=w2155) -> (w2151:string[][])  [unwired: 1 in]
                      }
                    }
                    n1246 = local write "Save1 Array"(w2135) -> ()
                  }
                  frame #7 {
                    w2172 = "On/Off I-Sat:"
                    n1247 = local read "Save1 Array"() -> (w2163:string[][])
                    n1248 = Array Size(array=w2163) -> (size(s)=w2169:i32[])
                    n1249 = Array Subset(array=w2163, index (row)=0, index (col)=0, length (col)=3) -> (w2165:string[][])  [unwired: 1 in]
                    n1250 = Index Array(array=w2169, index=0) -> (element=w2171:i32)
                    n1251 = Reshape Array(w2165, w2171) -> (w2164:string[])
                    n1252 = Search 1D Array(1D array=w2164, element=w2172) -> (index of element=w2175:i32)  [unwired: 1 in]
                    n1253 = Equal?(x=w2175, y=-1) -> (x = y?=w2174:bool)
                    n1254 = case shown="True" w2174 {
                      tunnel: w2163 -> [w2184 w2191]
                      tunnel: w2175 -> [w2181 _]
                      tunnel: [w2180 w2192] -> w2173
                      tunnel: w2164 -> [_ w2189]
                      tunnel: w2172 -> [_ w2187]
                      frame False {
                        n1255 = local read "Calc: On/Off"() -> (w2177:dbl)
                        n1256 = Divide(x=w2181, y=3) -> (x/y=w2183:dbl)
                        n1257 = To Word Integer(number=w2183) -> (16bit integer=w2182:i16)
                        n1258 = Format Value(format string="%#g", value (0)=w2177) -> (output string=w2178:string)  [unwired: 1 in]
                        n1259 = Replace Array Subset(array=w2184, new element=w2178, index (row)=w2182, index (col)=1) -> (w2180:string[][])
                      }
                      frame True {
                        n1260 = local read "Calc: On/Off"() -> (w2193:dbl)
                        n1261 = Search 1D Array(1D array=w2189, element="On/Off Current:") -> (index of element=w2196:i32)  [unwired: 1 in]
                        n1262 = Divide(x=w2196, y=3) -> (x/y=w2197:dbl)
                        n1263 = To Word Integer(number=w2197) -> (16bit integer=w2188:i16)
                        n1264 = Format Value(format string="%#g", value (0)=w2193) -> (output string=w2190:string)  [unwired: 1 in]
                        n1265 = Build Array(w2187, w2190) -> (w2195:string[])
                        n1266 = Replace Array Subset(array=w2191, new element=w2195, index (row)=w2188) -> (w2192:string[][])  [unwired: 1 in]
                      }
                    }
                    n1267 = local write "Save1 Array"(w2173) -> ()
                  }
                  frame #8 {
                    w2209 = "Off I-Sat (A):"
                    n1268 = local read "Save1 Array"() -> (w2200:string[][])
                    n1269 = Array Size(array=w2200) -> (size(s)=w2206:i32[])
                    n1270 = Array Subset(array=w2200, index (row)=0, index (col)=0, length (col)=3) -> (w2202:string[][])  [unwired: 1 in]
                    n1271 = Index Array(array=w2206, index=0) -> (element=w2208:i32)
                    n1272 = Reshape Array(w2202, w2208) -> (w2201:string[])
                    n1273 = Search 1D Array(1D array=w2201, element=w2209) -> (index of element=w2212:i32)  [unwired: 1 in]
                    n1274 = Equal?(x=w2212, y=-1) -> (x = y?=w2211:bool)
                    n1275 = case shown="True" w2211 {
                      tunnel: w2200 -> [w2221 w2227]
                      tunnel: w2212 -> [w2218 _]
                      tunnel: [w2217 w2226] -> w2210
                      tunnel: w2201 -> [_ w2225]
                      tunnel: w2209 -> [_ w2224]
                      frame False {
                        n1276 = local read "Calc: Off I-Sat"() -> (w2216:dbl)
                        n1277 = Divide(x=w2218, y=3) -> (x/y=w2220:dbl)
                        n1278 = Format Value(format string="%#g", value (0)=w2216) -> (output string=w2214:string)  [unwired: 1 in]
                        n1279 = To Word Integer(number=w2220) -> (16bit integer=w2219:i16)
                        n1280 = Replace Array Subset(array=w2221, new element=w2214, index (row)=w2219, index (col)=1) -> (w2217:string[][])
                      }
                      frame True {
                        n1281 = local read "Calc: Off I-Sat"() -> (w2228:dbl)
                        n1282 = Search 1D Array(1D array=w2225, element="On/Off I-Sat:") -> (index of element=w2233:i32)  [unwired: 1 in]
                        n1283 = Divide(x=w2233, y=3) -> (x/y=w2234:dbl)
                        n1284 = To Word Integer(number=w2234) -> (16bit integer=w2232:i16)
                        n1285 = Format Value(format string="%#g", value (0)=w2228) -> (output string=w2237:string)  [unwired: 1 in]
                        n1286 = Build Array(w2224, w2237) -> (w2230:string[])
                        n1287 = Increment(x=w2232) -> (x+1=w2231:i16)
                        n1288 = Insert Into Array(array=w2227, index (row)=w2231, new element=w2230) -> (w2226:string[][])  [unwired: 1 in]
                      }
                    }
                    n1289 = local write "Save1 Array"(w2210) -> ()
                  }
                  frame #9 {
                    w2239 = "Vt-Sat (V):"
                    n1290 = local read "Save1 Array"() -> (w2240:string[][])
                    n1291 = Array Size(array=w2240) -> (size(s)=w2245:i32[])
                    n1292 = Array Subset(array=w2240, index (row)=0, index (col)=0, length (col)=3) -> (w2241:string[][])  [unwired: 1 in]
                    n1293 = Index Array(array=w2245, index=0) -> (element=w2247:i32)
                    n1294 = Reshape Array(w2241, w2247) -> (w2238:string[])
                    n1295 = Search 1D Array(1D array=w2238, element=w2239) -> (index of element=w2250:i32)  [unwired: 1 in]
                    n1296 = Equal?(x=w2250, y=-1) -> (x = y?=w2249:bool)
                    n1297 = case shown="True" w2249 {
                      tunnel: w2240 -> [w2257 w2266]
                      tunnel: w2250 -> [w2253 _]
                      tunnel: [w2252 w2265] -> w2248
                      tunnel: w2239 -> [_ w2264]
                      tunnel: w2238 -> [_ w2263]
                      frame False {
                        n1298 = local read "New: VT-Sat"() -> (w2259:dbl)
                        n1299 = Number To Fractional String(number=w2259) -> (F-format string=w2254:string)  [unwired: 3 in]
                        n1300 = Divide(x=w2253, y=3) -> (x/y=w2256:dbl)
                        n1301 = To Word Integer(number=w2256) -> (16bit integer=w2255:i16)
                        n1302 = Replace Array Subset(array=w2257, new element=w2254, index (row)=w2255, index (col)=1) -> (w2252:string[][])
                      }
                      frame True {
                        n1303 = local read "New: VT-Sat"() -> (w2267:dbl)
                        n1304 = Search 1D Array(1D array=w2263, element="Threshold V (V):") -> (index of element=w2262:i32)  [unwired: 1 in]
                        n1305 = Divide(x=w2262, y=3) -> (x/y=w2270:dbl)
                        n1306 = To Word Integer(number=w2270) -> (16bit integer=w2261:i16)
                        n1307 = Format Value(format string="%#g", value (0)=w2267) -> (output string=w2273:string)  [unwired: 1 in]
                        n1308 = Build Array(w2264, w2273) -> (w2269:string[])
                        n1309 = Replace Array Subset(array=w2266, new element=w2269, index (row)=w2261) -> (w2265:string[][])  [unwired: 1 in]
                      }
                    }
                    n1310 = local write "Save1 Array"(w2248) -> ()
                  }
                  frame #10 {
                    n1311 = local read "Save1 Array"() -> (w2274:string[][])
                    n1312 = Array Size(array=w2274) -> (size(s)=w2280:i32[])
                    n1313 = Array Subset(array=w2274, index (row)=0, index (col)=0, length (col)=3) -> (w2276:string[][])  [unwired: 1 in]
                    n1314 = Index Array(array=w2280, index=0) -> (element=w2282:i32)
                    n1315 = Reshape Array(w2276, w2282) -> (w2275:string[])
                    n1316 = Search 1D Array(1D array=w2275, element="VT-Lin (V):") -> (index of element=w2285:i32)  [unwired: 1 in]
                    n1317 = Equal?(x=w2285, y=-1) -> (x = y?=w2284:bool)
                    n1318 = case shown="False" w2284 {
                      tunnel: w2274 -> [w2295 w2298]
                      tunnel: w2285 -> [w2292 _]
                      tunnel: [w2291 w2298] -> w2283
                      frame False {
                        n1319 = local read "New: VT-Lin"() -> (w2289:dbl)
                        n1320 = Divide(x=w2292, y=3) -> (x/y=w2294:dbl)
                        n1321 = Format Value(format string="%#g", value (0)=w2289) -> (output string=w2288:string)  [unwired: 1 in]
                        n1322 = To Word Integer(number=w2294) -> (16bit integer=w2293:i16)
                        n1323 = Replace Array Subset(array=w2295, new element=w2288, index (row)=w2293, index (col)=1) -> (w2291:string[][])
                      }
                      frame True {
                      }
                    }
                    n1324 = local write "Save1 Array"(w2283) -> ()
                  }
                  frame #11 {
                    w2299 = "STS-Sat (V/decade):"
                    n1325 = local read "Save1 Array"() -> (w2301:string[][])
                    n1326 = Array Size(array=w2301) -> (size(s)=w2306:i32[])
                    n1327 = Array Subset(array=w2301, index (row)=0, index (col)=0, length (col)=3) -> (w2302:string[][])  [unwired: 1 in]
                    n1328 = Index Array(array=w2306, index=0) -> (element=w2308:i32)
                    n1329 = Reshape Array(w2302, w2308) -> (w2300:string[])
                    n1330 = Search 1D Array(1D array=w2300, element=w2299) -> (index of element=w2311:i32)  [unwired: 1 in]
                    n1331 = Equal?(x=w2311, y=-1) -> (x = y?=w2310:bool)
                    n1332 = case shown="True" w2310 {
                      tunnel: w2301 -> [w2320 w2326]
                      tunnel: w2311 -> [w2317 _]
                      tunnel: [w2316 w2327] -> w2309
                      tunnel: w2300 -> [_ w2325]
                      tunnel: w2299 -> [_ w2324]
                      frame False {
                        n1333 = local read "New: STS"() -> (w2314:dbl)
                        n1334 = Divide(x=w2317, y=3) -> (x/y=w2319:dbl)
                        n1335 = Format Value(format string="%#g", value (0)=w2314) -> (output string=w2313:string)  [unwired: 1 in]
                        n1336 = To Word Integer(number=w2319) -> (16bit integer=w2318:i16)
                        n1337 = Replace Array Subset(array=w2320, new element=w2313, index (row)=w2318, index (col)=1) -> (w2316:string[][])
                      }
                      frame True {
                        n1338 = local read "New: STS"() -> (w2328:dbl)
                        n1339 = Search 1D Array(1D array=w2325, element="S.T.S. (V/decade):") -> (index of element=w2331:i32)  [unwired: 1 in]
                        n1340 = Divide(x=w2331, y=3) -> (x/y=w2332:dbl)
                        n1341 = To Word Integer(number=w2332) -> (16bit integer=w2323:i16)
                        n1342 = Format Value(format string="%#g", value (0)=w2328) -> (output string=w2335:string)  [unwired: 1 in]
                        n1343 = Build Array(w2324, w2335) -> (w2330:string[])
                        n1344 = Replace Array Subset(array=w2326, new element=w2330, index (row)=w2323) -> (w2327:string[][])  [unwired: 1 in]
                      }
                    }
                    n1345 = local write "Save1 Array"(w2309) -> ()
                  }
                  frame #12 {
                    w2336 = "Trap Density-VT (Traps/Vcm^2):"
                    n1346 = local read "Save1 Array"() -> (w2338:string[][])
                    n1347 = Array Size(array=w2338) -> (size(s)=w2343:i32[])
                    n1348 = Array Subset(array=w2338, index (row)=0, index (col)=0, length (col)=3) -> (w2339:string[][])  [unwired: 1 in]
                    n1349 = Index Array(array=w2343, index=0) -> (element=w2345:i32)
                    n1350 = Reshape Array(w2339, w2345) -> (w2337:string[])
                    n1351 = Search 1D Array(1D array=w2337, element=w2336) -> (index of element=w2348:i32)  [unwired: 1 in]
                    n1352 = Equal?(x=w2348, y=-1) -> (x = y?=w2347:bool)
                    n1353 = case shown="True" w2347 {
                      tunnel: w2338 -> [w2357 w2362]
                      tunnel: w2348 -> [w2353 _]
                      tunnel: [w2352 w2363] -> w2346
                      tunnel: w2337 -> [_ w2361]
                      tunnel: w2336 -> [_ w2360]
                      frame False {
                        n1354 = local read "New: Trap Density-VT"() -> (w2351:dbl)
                        n1355 = Format Value(format string="%#g", value (0)=w2351) -> (output string=w2354:string)  [unwired: 1 in]
                        n1356 = Divide(x=w2353, y=3) -> (x/y=w2356:dbl)
                        n1357 = To Word Integer(number=w2356) -> (16bit integer=w2355:i16)
                        n1358 = Replace Array Subset(array=w2357, new element=w2354, index (row)=w2355, index (col)=1) -> (w2352:string[][])
                      }
                      frame True {
                        n1359 = local read "New: Trap Density-VT"() -> (w2373:dbl)
                        n1360 = Search 1D Array(1D array=w2361, element="STS-Sat (V/decade):") -> (index of element=w2368:i32)  [unwired: 1 in]
                        n1361 = Divide(x=w2368, y=3) -> (x/y=w2367:dbl)
                        n1362 = To Word Integer(number=w2367) -> (16bit integer=w2369:i16)
                        n1363 = Format Value(format string="%#g", value (0)=w2373) -> (output string=w2364:string)  [unwired: 1 in]
                        n1364 = Build Array(w2360, w2364) -> (w2371:string[])
                        n1365 = Increment(x=w2369) -> (x+1=w2370:i16)
                        n1366 = Insert Into Array(array=w2362, index (row)=w2370, new element=w2371) -> (w2363:string[][])  [unwired: 1 in]
                      }
                    }
                    n1367 = local write "Save1 Array"(w2346) -> ()
                  }
                  frame #13 {
                    w2374 = "Trap Density-STS (Traps/Vcm^2):"
                    n1368 = local read "Save1 Array"() -> (w2376:string[][])
                    n1369 = Array Size(array=w2376) -> (size(s)=w2381:i32[])
                    n1370 = Array Subset(array=w2376, index (row)=0, index (col)=0, length (col)=3) -> (w2377:string[][])  [unwired: 1 in]
                    n1371 = Index Array(array=w2381, index=0) -> (element=w2383:i32)
                    n1372 = Reshape Array(w2377, w2383) -> (w2375:string[])
                    n1373 = Search 1D Array(1D array=w2375, element=w2374) -> (index of element=w2386:i32)  [unwired: 1 in]
                    n1374 = Equal?(x=w2386, y=-1) -> (x = y?=w2385:bool)
                    n1375 = case shown="True" w2385 {
                      tunnel: w2376 -> [w2395 w2400]
                      tunnel: w2386 -> [w2392 _]
                      tunnel: [w2391 w2401] -> w2384
                      tunnel: w2375 -> [_ w2399]
                      tunnel: w2374 -> [_ w2398]
                      frame False {
                        n1376 = local read "New: Trap Density-STS"() -> (w2389:dbl)
                        n1377 = Divide(x=w2392, y=3) -> (x/y=w2394:dbl)
                        n1378 = To Word Integer(number=w2394) -> (16bit integer=w2393:i16)
                        n1379 = Format Value(format string="%#g", value (0)=w2389) -> (output string=w2388:string)  [unwired: 1 in]
                        n1380 = Replace Array Subset(array=w2395, new element=w2388, index (row)=w2393, index (col)=1) -> (w2391:string[][])
                      }
                      frame True {
                        n1381 = local read "New: Trap Density-STS"() -> (w2402:dbl)
                        n1382 = Search 1D Array(1D array=w2399, element="Trap Density-VT (Traps/Vcm^2):") -> (index of element=w2407:i32)  [unwired: 1 in]
                        n1383 = Divide(x=w2407, y=3) -> (x/y=w2408:dbl)
                        n1384 = To Word Integer(number=w2408) -> (16bit integer=w2406:i16)
                        n1385 = Format Value(format string="%#g", value (0)=w2402) -> (output string=w2411:string)  [unwired: 1 in]
                        n1386 = Build Array(w2398, w2411) -> (w2404:string[])
                        n1387 = Increment(x=w2406) -> (x+1=w2405:i16)
                        n1388 = Insert Into Array(array=w2400, index (row)=w2405, new element=w2404) -> (w2401:string[][])  [unwired: 1 in]
                      }
                    }
                    n1389 = local write "Save1 Array"(w2384) -> ()
                  }
                }
                n1390 = Concatenate Strings(w1949, "\\", w1947) -> (w1948:string)
                n1391 = String To Path(string=w1948) -> (path=w1938:path)
                n1392 = disable-structure shown="Disabled" {
                  frame Disabled {
                  }
                  frame Enabled {
                  }
                }
              }
              frame #2 {
                n1393 = Equal?(x=w2470, y=w2467) -> (x = y?=w2469:bool)
                n1394 = case shown="False" w2469 {
                  tunnel: w2470 -> [w2473 _]
                  tunnel: w2467 -> [w2472 _]
                  frame False {
                    n1395 = Move(source path=w2473, 9:TRUE, 10:w2472) -> ()  [unwired: 2 in, 3 out]
                  }
                  frame True {
                  }
                }
              }
              frame #3 {
                n1396 = local write "Transfer File"(w2474) -> ()
                n1397 = call-poly <vilib>:"Write To Spreadsheet File.vi"("2D data"=w2475, "file path (dialog if empty)"=w2474) -> ()  [unwired: 6 in, 1 out]
              }
            }
          }
          event "Save Changes? 2": Mouse Down {
            n1398 = event-data() -> ()  [unwired: 1 in, 5 out]
            n1399 = stacked-sequence {
              seq-local: [w2533 _ _ _ _] -> [_ w3016 _ _ _]
              seq-local: [w2532 _ _ _ _] -> [_ w3017 _ _ _]
              seq-local: [w2532 _ _ _ _] -> [_ w3015 _ _ _]
              seq-local: [w2534 _ _ _ _] -> [_ w3013 _ _ _]
              seq-local: [_ w3017 _ _ _] -> [_ _ w3022 _ _]
              seq-local: [_ w3013 _ _ _] -> [_ _ w3021 _ _]
              frame #0 {
                n1400 = local read "Transfer File"() -> (w2533:path)
                n1401 = local read "New: Temp"() -> (w2536:dbl)
                n1402 = local read "New: Length"() -> (w2539:dbl)
                n1403 = local read "New: Width"() -> (w2537:dbl)
                n1404 = To Word Integer(number=w2536) -> (16bit integer=w2535:i16)
                n1405 = Number To Decimal String(number=w2535) -> (decimal integer string=w2543:string)  [unwired: 1 in]
                n1406 = To Single Precision Float(number=w2537) -> (single precision float=w2538:sgl)
                n1407 = To Single Precision Float(number=w2539) -> (single precision float=w2540:sgl)
                n1408 = local read "Index"() -> (w2547:string)
                n1409 = Strip Path(path=w2533) -> (stripped path=w2552:path)  [unwired: 1 out]
                n1410 = Number To Decimal String(number=w2540) -> (decimal integer string=w2545:string)  [unwired: 1 in]
                n1411 = Number To Decimal String(number=w2538) -> (decimal integer string=w2546:string)  [unwired: 1 in]
                n1412 = Concatenate Strings("_", w2543, "K") -> (w2541:string)
                n1413 = call "Build Text2"("Temp"=w2541, "Index"=w2547, "Length"=w2545, "Width"=w2546) -> ("Result"=w2548:string)  [unwired: 10 in, 1 out]
                n1414 = Path To String(path=w2552) -> (string=w2550:string)
                n1415 = Concatenate Strings(w2550, "\\", w2548) -> (w2549:string)
                n1416 = stacked-sequence {
                  tunnel: [_ _ _ _ _ _ _ _ _ _ _ _ _ w2975] -> _
                  tunnel: w2533 -> [w2554 _ _ _ _ _ _ _ _ _ _ _ _ _]
                  tunnel: [_ _ _ _ _ _ _ _ _ _ _ _ _ w2975] -> w2534
                  frame #0 {
                    n1417 = call-poly <vilib>:"Read From Spreadsheet File.vi"("file path (dialog if empty)"=w2554) -> ("all rows"=w2553:string[][])  [unwired: 6 in, 4 out]
                    n1418 = Array Size(array=w2553) -> (size(s)=w2558:i32[])
                    n1419 = Array Subset(array=w2553, index (row)=0, index (col)=0, length (col)=3) -> (w2562:string[][])  [unwired: 1 in]
                    n1420 = Index Array(array=w2558, index=0) -> (element=w2556:i32)
                    n1421 = Reshape Array(w2562, w2556) -> (w2555:string[])
                    n1422 = Search 1D Array(1D array=w2555, element="Dielectric (nm):") -> (index of element=w2565:i32)  [unwired: 1 in]
                    n1423 = Equal?(x=w2565, y=-1) -> (x = y?=w2564:bool)
                    n1424 = case shown="False" w2564 {
                      tunnel: w2553 -> [w2573 w2577]
                      tunnel: w2565 -> [w2569 _]
                      tunnel: [w2568 w2577] -> w2563
                      frame False {
                        n1425 = local read "New: Dielectric"() -> (w2575:dbl)
                        n1426 = Number To Fractional String(number=w2575) -> (F-format string=w2570:string)  [unwired: 3 in]
                        n1427 = Divide(x=w2569, y=3) -> (x/y=w2572:dbl)
                        n1428 = To Word Integer(number=w2572) -> (16bit integer=w2571:i16)
                        n1429 = Replace Array Subset(array=w2573, new element=w2570, index (row)=w2571, index (col)=1) -> (w2568:string[][])
                      }
                      frame True {
                      }
                    }
                    n1430 = local write "Save1 Array"(w2563) -> ()
                  }
                  frame #1 {
                    n1431 = local read "Save1 Array"() -> (w2579:string[][])
                    n1432 = Array Size(array=w2579) -> (size(s)=w2582:i32[])
                    n1433 = Array Subset(array=w2579, index (row)=0, index (col)=0, length (col)=3) -> (w2586:string[][])  [unwired: 1 in]
                    n1434 = Index Array(array=w2582, index=0) -> (element=w2580:i32)
                    n1435 = Reshape Array(w2586, w2580) -> (w2578:string[])
                    n1436 = Search 1D Array(1D array=w2578, element="Comments:") -> (index of element=w2589:i32)  [unwired: 1 in]
                    n1437 = Equal?(x=w2589, y=-1) -> (x = y?=w2588:bool)
                    n1438 = case shown="False" w2588 {
                      tunnel: w2579 -> [w2597 w2600]
                      tunnel: w2589 -> [w2594 _]
                      tunnel: [w2593 w2600] -> w2587
                      frame False {
                        n1439 = local read "Comments:"() -> (w2592:string)
                        n1440 = Divide(x=w2594, y=3) -> (x/y=w2596:dbl)
                        n1441 = To Word Integer(number=w2596) -> (16bit integer=w2595:i16)
                        n1442 = Replace Array Subset(array=w2597, new element=w2592, index (row)=w2595, index (col)=1) -> (w2593:string[][])
                      }
                      frame True {
                      }
                    }
                    n1443 = local write "Save1 Array"(w2587) -> ()
                  }
                  frame #2 {
                    n1444 = local read "Save1 Array"() -> (w2602:string[][])
                    n1445 = Array Size(array=w2602) -> (size(s)=w2605:i32[])
                    n1446 = Array Subset(array=w2602, index (row)=0, index (col)=0, length (col)=3) -> (w2609:string[][])  [unwired: 1 in]
                    n1447 = Index Array(array=w2605, index=0) -> (element=w2603:i32)
                    n1448 = Reshape Array(w2609, w2603) -> (w2601:string[])
                    n1449 = Search 1D Array(1D array=w2601, element="Length (um):") -> (index of element=w2612:i32)  [unwired: 1 in]
                    n1450 = Equal?(x=w2612, y=-1) -> (x = y?=w2611:bool)
                    n1451 = case shown="False" w2611 {
                      tunnel: w2602 -> [w2622 w2625]
                      tunnel: w2612 -> [w2619 _]
                      tunnel: [w2618 w2625] -> w2610
                      frame False {
                        n1452 = local read "New: Length"() -> (w2615:dbl)
                        n1453 = Divide(x=w2619, y=3) -> (x/y=w2621:dbl)
                        n1454 = Format Value(format string="%#g", value (0)=w2615) -> (output string=w2616:string)  [unwired: 1 in]
                        n1455 = To Word Integer(number=w2621) -> (16bit integer=w2620:i16)
                        n1456 = Replace Array Subset(array=w2622, new element=w2616, index (row)=w2620, index (col)=1) -> (w2618:string[][])
                      }
                      frame True {
                      }
                    }
                    n1457 = local write "Save1 Array"(w2610) -> ()
                  }
                  frame #3 {
                    n1458 = local read "Save1 Array"() -> (w2627:string[][])
                    n1459 = Array Size(array=w2627) -> (size(s)=w2632:i32[])
                    n1460 = Array Subset(array=w2627, index (row)=0, index (col)=0, length (col)=3) -> (w2628:string[][])  [unwired: 1 in]
                    n1461 = Index Array(array=w2632, index=0) -> (element=w2634:i32)
                    n1462 = Reshape Array(w2628, w2634) -> (w2626:string[])
                    n1463 = Search 1D Array(1D array=w2626, element="Width (um):") -> (index of element=w2637:i32)  [unwired: 1 in]
                    n1464 = Equal?(x=w2637, y=-1) -> (x = y?=w2636:bool)
                    n1465 = case shown="False" w2636 {
                      tunnel: w2637 -> [w2645 _]
                      tunnel: w2627 -> [w2644 w2650]
                      tunnel: [w2643 w2650] -> w2635
                      frame False {
                        n1466 = local read "New: Width"() -> (w2640:dbl)
                        n1467 = Divide(x=w2645, y=3) -> (x/y=w2647:dbl)
                        n1468 = To Word Integer(number=w2647) -> (16bit integer=w2646:i16)
                        n1469 = Format Value(format string="%#g", value (0)=w2640) -> (output string=w2641:string)  [unwired: 1 in]
                        n1470 = Replace Array Subset(array=w2644, new element=w2641, index (row)=w2646, index (col)=1) -> (w2643:string[][])
                      }
                      frame True {
                      }
                    }
                    n1471 = local write "Save1 Array"(w2635) -> ()
                  }
                  frame #4 {
                    w2660 = "Sample Temp (K):"
                    n1472 = local read "Save1 Array"() -> (w2652:string[][])
                    n1473 = Array Size(array=w2652) -> (size(s)=w2657:i32[])
                    n1474 = Array Subset(array=w2652, index (row)=0, index (col)=0, length (col)=3) -> (w2653:string[][])  [unwired: 1 in]
                    n1475 = Index Array(array=w2657, index=0) -> (element=w2659:i32)
                    n1476 = Reshape Array(w2653, w2659) -> (w2651:string[])
                    n1477 = Search 1D Array(1D array=w2651, element=w2660) -> (index of element=w2663:i32)  [unwired: 1 in]
                    n1478 = Equal?(x=w2663, y=-1) -> (x = y?=w2662:bool)
                    n1479 = case shown="True" w2662 {
                      tunnel: w2652 -> [w2672 w2686]
                      tunnel: w2663 -> [w2669 _]
                      tunnel: [w2668 w2685] -> w2661
                      tunnel: w2651 -> [_ w2688]
                      tunnel: w2660 -> [_ w2675]
                      frame False {
                        n1480 = local read "New: Temp"() -> (w2666:dbl)
                        n1481 = Divide(x=w2669, y=3) -> (x/y=w2671:dbl)
                        n1482 = Format Value(format string="%#g", value (0)=w2666) -> (output string=w2665:string)  [unwired: 1 in]
                        n1483 = To Word Integer(number=w2671) -> (16bit integer=w2670:i16)
                        n1484 = Replace Array Subset(array=w2672, new element=w2665, index (row)=w2670, index (col)=1) -> (w2668:string[][])
                      }
                      frame True {
                        n1485 = local read "New: Temp"() -> (w2677:dbl)
                        n1486 = Search 1D Array(1D array=w2688, element="Width (um):") -> (index of element=w2682:i32)  [unwired: 1 in]
                        n1487 = Divide(x=w2682, y=3) -> (x/y=w2683:dbl)
                        n1488 = To Word Integer(number=w2683) -> (16bit integer=w2681:i16)
                        n1489 = Format Value(format string="%#g", value (0)=w2677) -> (output string=w2676:string)  [unwired: 1 in]
                        n1490 = Build Array(w2675, w2676) -> (w2679:string[])
                        n1491 = Increment(x=w2681) -> (x+1=w2680:i16)
                        n1492 = Insert Into Array(array=w2686, index (row)=w2680, new element=w2679) -> (w2685:string[][])  [unwired: 1 in]
                      }
                    }
                    n1493 = local write "Save1 Array"(w2661) -> ()
                  }
                  frame #5 {
                    w2698 = "Mobility-Sat (cm^2/Vs):"
                    n1494 = local read "Save1 Array"() -> (w2690:string[][])
                    n1495 = Array Size(array=w2690) -> (size(s)=w2695:i32[])
                    n1496 = Array Subset(array=w2690, index (row)=0, index (col)=0, length (col)=3) -> (w2691:string[][])  [unwired: 1 in]
                    n1497 = Index Array(array=w2695, index=0) -> (element=w2697:i32)
                    n1498 = Reshape Array(w2691, w2697) -> (w2689:string[])
                    n1499 = Search 1D Array(1D array=w2689, element=w2698) -> (index of element=w2701:i32)  [unwired: 1 in]
                    n1500 = Equal?(x=w2701, y=-1) -> (x = y?=w2700:bool)
                    n1501 = case shown="True" w2700 {
                      tunnel: w2690 -> [w2710 w2718]
                      tunnel: w2701 -> [w2707 _]
                      tunnel: [w2706 w2717] -> w2699
                      tunnel: w2689 -> [_ w2715]
                      tunnel: w2698 -> [_ w2713]
                      frame False {
                        n1502 = local read "New: Mobility-Sat"() -> (w2703:dbl)
                        n1503 = Divide(x=w2707, y=3) -> (x/y=w2709:dbl)
                        n1504 = To Word Integer(number=w2709) -> (16bit integer=w2708:i16)
                        n1505 = Format Value(format string="%#g", value (0)=w2703) -> (output string=w2704:string)  [unwired: 1 in]
                        n1506 = Replace Array Subset(array=w2710, new element=w2704, index (row)=w2708, index (col)=1) -> (w2706:string[][])
                      }
                      frame True {
                        n1507 = local read "New: Mobility-Sat"() -> (w2719:dbl)
                        n1508 = Search 1D Array(1D array=w2715, element="Mobility (cm^2/Vs):") -> (index of element=w2722:i32)  [unwired: 1 in]
                        n1509 = Divide(x=w2722, y=3) -> (x/y=w2723:dbl)
                        n1510 = To Word Integer(number=w2723) -> (16bit integer=w2714:i16)
                        n1511 = Format Value(format string="%#g", value (0)=w2719) -> (output string=w2716:string)  [unwired: 1 in]
                        n1512 = Build Array(w2713, w2716) -> (w2721:string[])
                        n1513 = Replace Array Subset(array=w2718, new element=w2721, index (row)=w2714) -> (w2717:string[][])  [unwired: 1 in]
                      }
                    }
                    n1514 = local write "Save1 Array"(w2699) -> ()
                  }
                  frame #6 {
                    w2735 = "Mobility-Lin (cm^2/Vs):"
                    n1515 = local read "Save1 Array"() -> (w2726:string[][])
                    n1516 = Array Size(array=w2726) -> (size(s)=w2732:i32[])
                    n1517 = Array Subset(array=w2726, index (row)=0, index (col)=0, length (col)=3) -> (w2728:string[][])  [unwired: 1 in]
                    n1518 = Index Array(array=w2732, index=0) -> (element=w2734:i32)
                    n1519 = Reshape Array(w2728, w2734) -> (w2727:string[])
                    n1520 = Search 1D Array(1D array=w2727, element=w2735) -> (index of element=w2738:i32)  [unwired: 1 in]
                    n1521 = Equal?(x=w2738, y=-1) -> (x = y?=w2737:bool)
                    n1522 = case shown="True" w2737 {
                      tunnel: w2726 -> [w2747 w2753]
                      tunnel: w2738 -> [w2744 _]
                      tunnel: [w2743 w2752] -> w2736
                      tunnel: w2727 -> [_ w2751]
                      tunnel: w2735 -> [_ w2750]
                      frame False {
                        n1523 = local read "Calc: Mobility-Lin"() -> (w2740:dbl)
                        n1524 = Divide(x=w2744, y=3) -> (x/y=w2746:dbl)
                        n1525 = To Word Integer(number=w2746) -> (16bit integer=w2745:i16)
                        n1526 = Format Value(format string="%#g", value (0)=w2740) -> (output string=w2741:string)  [unwired: 1 in]
                        n1527 = Replace Array Subset(array=w2747, new element=w2741, index (row)=w2745, index (col)=1) -> (w2743:string[][])
                      }
                      frame True {
                        n1528 = local read "Calc: Mobility-Lin"() -> (w2754:dbl)
                        n1529 = Search 1D Array(1D array=w2751, element="Mobility-Sat (cm^2/Vs):") -> (index of element=w2759:i32)  [unwired: 1 in]
                        n1530 = Divide(x=w2759, y=3) -> (x/y=w2760:dbl)
                        n1531 = To Word Integer(number=w2760) -> (16bit integer=w2758:i16)
                        n1532 = Format Value(format string="%#g", value (0)=w2754) -> (output string=w2763:string)  [unwired: 1 in]
                        n1533 = Build Array(w2750, w2763) -> (w2756:string[])
                        n1534 = Increment(x=w2758) -> (x+1=w2757:i16)
                        n1535 = Insert Into Array(array=w2753, index (row)=w2757, new element=w2756) -> (w2752:string[][])  [unwired: 1 in]
                      }
                    }
                    n1536 = local write "Save1 Array"(w2736) -> ()
                  }
                  frame #7 {
                    w2773 = "On/Off I-Sat:"
                    n1537 = local read "Save1 Array"() -> (w2764:string[][])
                    n1538 = Array Size(array=w2764) -> (size(s)=w2770:i32[])
                    n1539 = Array Subset(array=w2764, index (row)=0, index (col)=0, length (col)=3) -> (w2766:string[][])  [unwired: 1 in]
                    n1540 = Index Array(array=w2770, index=0) -> (element=w2772:i32)
                    n1541 = Reshape Array(w2766, w2772) -> (w2765:string[])
                    n1542 = Search 1D Array(1D array=w2765, element=w2773) -> (index of element=w2776:i32)  [unwired: 1 in]
                    n1543 = Equal?(x=w2776, y=-1) -> (x = y?=w2775:bool)
                    n1544 = case shown="True" w2775 {
                      tunnel: w2764 -> [w2785 w2792]
                      tunnel: w2776 -> [w2782 _]
                      tunnel: [w2781 w2793] -> w2774
                      tunnel: w2765 -> [_ w2790]
                      tunnel: w2773 -> [_ w2788]
                      frame False {
                        n1545 = local read "Calc: On/Off"() -> (w2778:dbl)
                        n1546 = Divide(x=w2782, y=3) -> (x/y=w2784:dbl)
                        n1547 = To Word Integer(number=w2784) -> (16bit integer=w2783:i16)
                        n1548 = Format Value(format string="%#g", value (0)=w2778) -> (output string=w2779:string)  [unwired: 1 in]
                        n1549 = Replace Array Subset(array=w2785, new element=w2779, index (row)=w2783, index (col)=1) -> (w2781:string[][])
                      }
                      frame True {
                        n1550 = local read "Calc: On/Off"() -> (w2794:dbl)
                        n1551 = Search 1D Array(1D array=w2790, element="On/Off Current:") -> (index of element=w2797:i32)  [unwired: 1 in]
                        n1552 = Divide(x=w2797, y=3) -> (x/y=w2798:dbl)
                        n1553 = To Word Integer(number=w2798) -> (16bit integer=w2789:i16)
                        n1554 = Format Value(format string="%#g", value (0)=w2794) -> (output string=w2791:string)  [unwired: 1 in]
                        n1555 = Build Array(w2788, w2791) -> (w2796:string[])
                        n1556 = Replace Array Subset(array=w2792, new element=w2796, index (row)=w2789) -> (w2793:string[][])  [unwired: 1 in]
                      }
                    }
                    n1557 = local write "Save1 Array"(w2774) -> ()
                  }
                  frame #8 {
                    w2810 = "Off I-Sat (A):"
                    n1558 = local read "Save1 Array"() -> (w2801:string[][])
                    n1559 = Array Size(array=w2801) -> (size(s)=w2807:i32[])
                    n1560 = Array Subset(array=w2801, index (row)=0, index (col)=0, length (col)=3) -> (w2803:string[][])  [unwired: 1 in]
                    n1561 = Index Array(array=w2807, index=0) -> (element=w2809:i32)
                    n1562 = Reshape Array(w2803, w2809) -> (w2802:string[])
                    n1563 = Search 1D Array(1D array=w2802, element=w2810) -> (index of element=w2813:i32)  [unwired: 1 in]
                    n1564 = Equal?(x=w2813, y=-1) -> (x = y?=w2812:bool)
                    n1565 = case shown="True" w2812 {
                      tunnel: w2801 -> [w2822 w2828]
                      tunnel: w2813 -> [w2819 _]
                      tunnel: [w2818 w2827] -> w2811
                      tunnel: w2802 -> [_ w2826]
                      tunnel: w2810 -> [_ w2825]
                      frame False {
                        n1566 = local read "Calc: Off I-Sat"() -> (w2817:dbl)
                        n1567 = Divide(x=w2819, y=3) -> (x/y=w2821:dbl)
                        n1568 = Format Value(format string="%#g", value (0)=w2817) -> (output string=w2815:string)  [unwired: 1 in]
                        n1569 = To Word Integer(number=w2821) -> (16bit integer=w2820:i16)
                        n1570 = Replace Array Subset(array=w2822, new element=w2815, index (row)=w2820, index (col)=1) -> (w2818:string[][])
                      }
                      frame True {
                        n1571 = local read "Calc: Off I-Sat"() -> (w2829:dbl)
                        n1572 = Search 1D Array(1D array=w2826, element="On/Off I-Sat:") -> (index of element=w2834:i32)  [unwired: 1 in]
                        n1573 = Divide(x=w2834, y=3) -> (x/y=w2835:dbl)
                        n1574 = To Word Integer(number=w2835) -> (16bit integer=w2833:i16)
                        n1575 = Format Value(format string="%#g", value (0)=w2829) -> (output string=w2838:string)  [unwired: 1 in]
                        n1576 = Build Array(w2825, w2838) -> (w2831:string[])
                        n1577 = Increment(x=w2833) -> (x+1=w2832:i16)
                        n1578 = Insert Into Array(array=w2828, index (row)=w2832, new element=w2831) -> (w2827:string[][])  [unwired: 1 in]
                      }
                    }
                    n1579 = local write "Save1 Array"(w2811) -> ()
                  }
                  frame #9 {
                    w2840 = "Vt-Sat (V):"
                    n1580 = local read "Save1 Array"() -> (w2841:string[][])
                    n1581 = Array Size(array=w2841) -> (size(s)=w2846:i32[])
                    n1582 = Array Subset(array=w2841, index (row)=0, index (col)=0, length (col)=3) -> (w2842:string[][])  [unwired: 1 in]
                    n1583 = Index Array(array=w2846, index=0) -> (element=w2848:i32)
                    n1584 = Reshape Array(w2842, w2848) -> (w2839:string[])
                    n1585 = Search 1D Array(1D array=w2839, element=w2840) -> (index of element=w2851:i32)  [unwired: 1 in]
                    n1586 = Equal?(x=w2851, y=-1) -> (x = y?=w2850:bool)
                    n1587 = case shown="True" w2850 {
                      tunnel: w2841 -> [w2858 w2867]
                      tunnel: w2851 -> [w2854 _]
                      tunnel: [w2853 w2866] -> w2849
                      tunnel: w2840 -> [_ w2865]
                      tunnel: w2839 -> [_ w2864]
                      frame False {
                        n1588 = local read "New: VT-Sat"() -> (w2860:dbl)
                        n1589 = Number To Fractional String(number=w2860) -> (F-format string=w2855:string)  [unwired: 3 in]
                        n1590 = Divide(x=w2854, y=3) -> (x/y=w2857:dbl)
                        n1591 = To Word Integer(number=w2857) -> (16bit integer=w2856:i16)
                        n1592 = Replace Array Subset(array=w2858, new element=w2855, index (row)=w2856, index (col)=1) -> (w2853:string[][])
                      }
                      frame True {
                        n1593 = local read "New: VT-Sat"() -> (w2868:dbl)
                        n1594 = Search 1D Array(1D array=w2864, element="Threshold V (V):") -> (index of element=w2863:i32)  [unwired: 1 in]
                        n1595 = Divide(x=w2863, y=3) -> (x/y=w2871:dbl)
                        n1596 = To Word Integer(number=w2871) -> (16bit integer=w2862:i16)
                        n1597 = Format Value(format string="%#g", value (0)=w2868) -> (output string=w2874:string)  [unwired: 1 in]
                        n1598 = Build Array(w2865, w2874) -> (w2870:string[])
                        n1599 = Replace Array Subset(array=w2867, new element=w2870, index (row)=w2862) -> (w2866:string[][])  [unwired: 1 in]
                      }
                    }
                    n1600 = local write "Save1 Array"(w2849) -> ()
                  }
                  frame #10 {
                    n1601 = local read "Save1 Array"() -> (w2875:string[][])
                    n1602 = Array Size(array=w2875) -> (size(s)=w2881:i32[])
                    n1603 = Array Subset(array=w2875, index (row)=0, index (col)=0, length (col)=3) -> (w2877:string[][])  [unwired: 1 in]
                    n1604 = Index Array(array=w2881, index=0) -> (element=w2883:i32)
                    n1605 = Reshape Array(w2877, w2883) -> (w2876:string[])
                    n1606 = Search 1D Array(1D array=w2876, element="VT-Lin (V):") -> (index of element=w2886:i32)  [unwired: 1 in]
                    n1607 = Equal?(x=w2886, y=-1) -> (x = y?=w2885:bool)
                    n1608 = case shown="False" w2885 {
                      tunnel: w2875 -> [w2896 w2899]
                      tunnel: w2886 -> [w2893 _]
                      tunnel: [w2892 w2899] -> w2884
                      frame False {
                        n1609 = local read "New: VT-Lin"() -> (w2890:dbl)
                        n1610 = Divide(x=w2893, y=3) -> (x/y=w2895:dbl)
                        n1611 = Format Value(format string="%#g", value (0)=w2890) -> (output string=w2889:string)  [unwired: 1 in]
                        n1612 = To Word Integer(number=w2895) -> (16bit integer=w2894:i16)
                        n1613 = Replace Array Subset(array=w2896, new element=w2889, index (row)=w2894, index (col)=1) -> (w2892:string[][])
                      }
                      frame True {
                      }
                    }
                    n1614 = local write "Save1 Array"(w2884) -> ()
                  }
                  frame #11 {
                    w2900 = "STS-Sat (V/decade):"
                    n1615 = local read "Save1 Array"() -> (w2902:string[][])
                    n1616 = Array Size(array=w2902) -> (size(s)=w2907:i32[])
                    n1617 = Array Subset(array=w2902, index (row)=0, index (col)=0, length (col)=3) -> (w2903:string[][])  [unwired: 1 in]
                    n1618 = Index Array(array=w2907, index=0) -> (element=w2909:i32)
                    n1619 = Reshape Array(w2903, w2909) -> (w2901:string[])
                    n1620 = Search 1D Array(1D array=w2901, element=w2900) -> (index of element=w2912:i32)  [unwired: 1 in]
                    n1621 = Equal?(x=w2912, y=-1) -> (x = y?=w2911:bool)
                    n1622 = case shown="True" w2911 {
                      tunnel: w2902 -> [w2921 w2927]
                      tunnel: w2912 -> [w2918 _]
                      tunnel: [w2917 w2928] -> w2910
                      tunnel: w2901 -> [_ w2926]
                      tunnel: w2900 -> [_ w2925]
                      frame False {
                        n1623 = local read "New: STS"() -> (w2915:dbl)
                        n1624 = Divide(x=w2918, y=3) -> (x/y=w2920:dbl)
                        n1625 = Format Value(format string="%#g", value (0)=w2915) -> (output string=w2914:string)  [unwired: 1 in]
                        n1626 = To Word Integer(number=w2920) -> (16bit integer=w2919:i16)
                        n1627 = Replace Array Subset(array=w2921, new element=w2914, index (row)=w2919, index (col)=1) -> (w2917:string[][])
                      }
                      frame True {
                        n1628 = local read "New: STS"() -> (w2929:dbl)
                        n1629 = Search 1D Array(1D array=w2926, element="S.T.S. (V/decade):") -> (index of element=w2932:i32)  [unwired: 1 in]
                        n1630 = Divide(x=w2932, y=3) -> (x/y=w2933:dbl)
                        n1631 = To Word Integer(number=w2933) -> (16bit integer=w2924:i16)
                        n1632 = Format Value(format string="%#g", value (0)=w2929) -> (output string=w2936:string)  [unwired: 1 in]
                        n1633 = Build Array(w2925, w2936) -> (w2931:string[])
                        n1634 = Replace Array Subset(array=w2927, new element=w2931, index (row)=w2924) -> (w2928:string[][])  [unwired: 1 in]
                      }
                    }
                    n1635 = local write "Save1 Array"(w2910) -> ()
                  }
                  frame #12 {
                    w2937 = "Trap Density-VT (Traps/Vcm^2):"
                    n1636 = local read "Save1 Array"() -> (w2939:string[][])
                    n1637 = Array Size(array=w2939) -> (size(s)=w2944:i32[])
                    n1638 = Array Subset(array=w2939, index (row)=0, index (col)=0, length (col)=3) -> (w2940:string[][])  [unwired: 1 in]
                    n1639 = Index Array(array=w2944, index=0) -> (element=w2946:i32)
                    n1640 = Reshape Array(w2940, w2946) -> (w2938:string[])
                    n1641 = Search 1D Array(1D array=w2938, element=w2937) -> (index of element=w2949:i32)  [unwired: 1 in]
                    n1642 = Equal?(x=w2949, y=-1) -> (x = y?=w2948:bool)
                    n1643 = case shown="True" w2948 {
                      tunnel: w2939 -> [w2958 w2963]
                      tunnel: w2949 -> [w2954 _]
                      tunnel: [w2953 w2964] -> w2947
                      tunnel: w2938 -> [_ w2962]
                      tunnel: w2937 -> [_ w2961]
                      frame False {
                        n1644 = local read "New: Trap Density-VT"() -> (w2952:dbl)
                        n1645 = Format Value(format string="%#g", value (0)=w2952) -> (output string=w2955:string)  [unwired: 1 in]
                        n1646 = Divide(x=w2954, y=3) -> (x/y=w2957:dbl)
                        n1647 = To Word Integer(number=w2957) -> (16bit integer=w2956:i16)
                        n1648 = Replace Array Subset(array=w2958, new element=w2955, index (row)=w2956, index (col)=1) -> (w2953:string[][])
                      }
                      frame True {
                        n1649 = local read "New: Trap Density-VT"() -> (w2974:dbl)
                        n1650 = Search 1D Array(1D array=w2962, element="STS-Sat (V/decade):") -> (index of element=w2969:i32)  [unwired: 1 in]
                        n1651 = Divide(x=w2969, y=3) -> (x/y=w2968:dbl)
                        n1652 = To Word Integer(number=w2968) -> (16bit integer=w2970:i16)
                        n1653 = Format Value(format string="%#g", value (0)=w2974) -> (output string=w2965:string)  [unwired: 1 in]
                        n1654 = Build Array(w2961, w2965) -> (w2972:string[])
                        n1655 = Increment(x=w2970) -> (x+1=w2971:i16)
                        n1656 = Insert Into Array(array=w2963, index (row)=w2971, new element=w2972) -> (w2964:string[][])  [unwired: 1 in]
                      }
                    }
                    n1657 = local write "Save1 Array"(w2947) -> ()
                  }
                  frame #13 {
                    w2976 = "Trap Density-STS (Traps/Vcm^2):"
                    n1658 = local read "Save1 Array"() -> (w2978:string[][])
                    n1659 = Array Size(array=w2978) -> (size(s)=w2983:i32[])
                    n1660 = Array Subset(array=w2978, index (row)=0, index (col)=0, length (col)=3) -> (w2979:string[][])  [unwired: 1 in]
                    n1661 = Index Array(array=w2983, index=0) -> (element=w2985:i32)
                    n1662 = Reshape Array(w2979, w2985) -> (w2977:string[])
                    n1663 = Search 1D Array(1D array=w2977, element=w2976) -> (index of element=w2987:i32)  [unwired: 1 in]
                    n1664 = Equal?(x=w2987, y=-1) -> (x = y?=w2986:bool)
                    n1665 = case shown="True" w2986 {
                      tunnel: w2978 -> [w2996 w3001]
                      tunnel: w2987 -> [w2993 _]
                      tunnel: [w2992 w3002] -> w2975
                      tunnel: w2977 -> [_ w3000]
                      tunnel: w2976 -> [_ w2999]
                      frame False {
                        n1666 = local read "New: Trap Density-STS"() -> (w2990:dbl)
                        n1667 = Divide(x=w2993, y=3) -> (x/y=w2995:dbl)
                        n1668 = To Word Integer(number=w2995) -> (16bit integer=w2994:i16)
                        n1669 = Format Value(format string="%#g", value (0)=w2990) -> (output string=w2989:string)  [unwired: 1 in]
                        n1670 = Replace Array Subset(array=w2996, new element=w2989, index (row)=w2994, index (col)=1) -> (w2992:string[][])
                      }
                      frame True {
                        n1671 = local read "New: Trap Density-STS"() -> (w3003:dbl)
                        n1672 = Search 1D Array(1D array=w3000, element="Trap Density-VT (Traps/Vcm^2):") -> (index of element=w3008:i32)  [unwired: 1 in]
                        n1673 = Divide(x=w3008, y=3) -> (x/y=w3009:dbl)
                        n1674 = To Word Integer(number=w3009) -> (16bit integer=w3007:i16)
                        n1675 = Format Value(format string="%#g", value (0)=w3003) -> (output string=w3012:string)  [unwired: 1 in]
                        n1676 = Build Array(w2999, w3012) -> (w3005:string[])
                        n1677 = Increment(x=w3007) -> (x+1=w3006:i16)
                        n1678 = Insert Into Array(array=w3001, index (row)=w3006, new element=w3005) -> (w3002:string[][])  [unwired: 1 in]
                      }
                    }
                    n1679 = local write "Save1 Array"(w2975) -> ()
                  }
                }
                n1680 = String To Path(string=w2549) -> (path=w2532:path)
                "No Image 2" <- w2532
              }
              frame #1 {
                n1681 = Equal?(x=w3016, y=w3015) -> (x = y?=w3014:bool)
                n1682 = case shown="False" w3014 {
                  tunnel: w3016 -> [w3020 _]
                  tunnel: w3015 -> [w3019 _]
                  frame False {
                    n1683 = Move(source path=w3020, 9:TRUE, 10:w3019) -> ()  [unwired: 2 in, 3 out]
                  }
                  frame True {
                  }
                }
              }
              frame #2 {
                n1684 = local write "Transfer File"(w3022) -> ()
                n1685 = call-poly <vilib>:"Write To Spreadsheet File.vi"("2D data"=w3021, "file path (dialog if empty)"=w3022) -> ()  [unwired: 6 in, 1 out]
              }
              frame #3 {
                w3032 = "\\"
                w3033 = "TSP"
                w3171 = 0
                # "Transpose"
                # "Moves to next file and displays new image/data"
                n1686 = property on="Image Out" class="ImageControl"() -> (error out=w3134:errorcluster, "Image Center Position"=w3138:cluster{"X":u32, "Y":u32})  [unwired: 2 in, 1 out]
                n1687 = local read "Transfer File"() -> (w3176:path)
                n1688 = Strip Path(path=w3176) -> (stripped path=w3025:path, name=w3184:string)
                n1689 = Unbundle(w3138) -> ("X"=w3136:u32)  [unwired: 1 out]
                n1690 = Strip Path(path=w3025) -> (stripped path=w3028:path)  [unwired: 1 out]
                n1691 = local write "Transfer Folder"(w3025) -> ()
                n1692 = Bundle("X"=w3136, 0) -> (w3137:cluster{"X":u32, i32})  [unwired: 1 in]
                n1693 = local read "Folder Index"() -> (w3046:dbl)
                n1694 = Path To String(path=w3028) -> (string=w3031:string)
                n1695 = property on="Image Out" class="ImageControl"(error in=w3134, "Image Center Position"=w3137) -> ()  [unwired: 1 in, 2 out]
                n1696 = List Folder(path=w3025) -> (filenames=w3181:string[])  [unwired: 3 in, 3 out]
                n1697 = Search 1D Array(1D array=w3181, element=w3184) -> (index of element=w3178:i32)  [unwired: 1 in]
                n1698 = Array Size(array=w3181) -> (size(s)=w3177:i32)
                n1699 = Decrement(x=w3177) -> (x-1=w3179:i32)
                n1700 = Equal?(x=w3178, y=w3179) -> (x = y?=w3180:bool)
                n1701 = local read "Folder Index"() -> (w3130:dbl)
                n1702 = case shown="False" w3180 {
                  tunnel: w3130 -> [w3320 _]
                  tunnel: [w3319 0] -> w3129
                  frame False {
                    n1703 = Increment(x=w3320) -> (x+1=w3319:dbl)
                  }
                  frame True {
                  }
                }
                n1704 = invoke on="Image Out" class="ImageControl" method="Clear ROI"() -> ()  [unwired: 3 in, 3 out]
                n1705 = local write "Folder Index"(w3129) -> ()
                n1706 = Path To String(path=w3025) -> (string=w3185:string)
                n1707 = Index Array(array=w3181, index=w3129) -> (element=w3024:string)
                n1708 = String Subset(string=w3024, offset (0)=3) -> (substring=w3027:string)  [unwired: 1 in]
                n1709 = Concatenate Strings(w3033, w3027) -> (w3029:string)
                n1710 = Concatenate Strings(w3031, w3032, w3033, w3032, w3029) -> (w3030:string)
                n1711 = String To Path(string=w3030) -> (path=w3023:path)
                n1712 = local write "Transport File"(w3023) -> ()
                n1713 = Strip Path(path=w3023) -> (stripped path=w3045:path, name=w3036:string)
                n1714 = local write "Transport Folder"(w3045) -> ()
                n1715 = List Folder(path=w3045) -> (filenames=w3040:string[], error out=w3048:errorcluster)  [unwired: 3 in, 2 out]
                n1716 = Array Size(array=w3040) -> (size(s)=w3044:i32)
                n1717 = Search 1D Array(1D array=w3040, element=w3036) -> (index of element=w3043:i32)  [unwired: 1 in]
                n1718 = Decrement(x=w3044) -> (x-1=w3042:i32)
                n1719 = Equal?(x=w3043, y=w3042) -> (x = y?=w3041:bool)
                n1720 = case shown="False" w3041 {
                  tunnel: w3046 -> [w3188 _]
                  tunnel: [w3187 0] -> w3047
                  tunnel: w3048 -> [w3186 w3189]
                  tunnel: [w3186 w3189] -> _
                  frame False {
                    n1721 = Increment(x=w3188) -> (x+1=w3187:dbl)
                  }
                  frame True {
                  }
                }
                n1722 = local write "Folder Index"(w3047) -> ()
                n1723 = Path To String(path=w3045) -> (string=w3035:string)
                n1724 = Index Array(array=w3040, index=w3047) -> (element=w3039:string)
                n1725 = local write "Data Name:"(w3039) -> ()
                n1726 = Concatenate Strings(w3035, "\\", w3039) -> (w3037:string)
                n1727 = String To Path(string=w3037) -> (path=w3034:path)
                n1728 = Strip Path(path=w3034) -> ()  [unwired: 2 out]
                n1729 = call-poly <vilib>:"Read From Spreadsheet File.vi"("file path (dialog if empty)"=w3034) -> ("all rows"=w3062:string[][])  [unwired: 6 in, 4 out]
                n1730 = Array Size(array=w3062) -> (size(s)=w3068:i32[])
                n1731 = Array Subset(array=w3062, length (col)=1) -> (w3064:string[][])  [unwired: 3 in]
                n1732 = Index Array(array=w3068, index=0) -> (element=w3057:i32)
                n1733 = Reshape Array(w3064, w3057) -> (w3063:string[])
                n1734 = Search 1D Array(1D array=w3063, element="Vd") -> (index of element=w3061:i32)  [unwired: 1 in]
                n1735 = Increment(x=w3061) -> (x+1=w3060:i32)
                n1736 = Array Subset(array=w3062, index (row)=w3060) -> (w3058:string[][])  [unwired: 3 in]
                n1737 = local write "Data Name:"(w3024) -> ()
                n1738 = Fract/Exp String To Number(string=w3058, default (0 dbl)="default (0 dbl) 4") -> (number=w3050:ext[][])  [unwired: 2 in, 1 out]
                n1739 = Delete From Array(array=w3050) -> (array with subset deleted=w3049:ext[][])  [unwired: 3 in, 1 out]
                n1740 = Concatenate Strings(w3185, "\\", w3024) -> (w3183:string)
                n1741 = Delete From Array(array=w3049, index (col)=0 ("Deaktivierter Index (Spalte)")) -> (deleted portion=w3054:ext[], array with subset deleted=w3055:ext[][])  [unwired: 2 in]
                n1742 = String To Path(string=w3183) -> (path=w3083:path)
                n1743 = call "Recorded Values.vi"("Path"=w3083) -> ("Recorded Char"=w3085:T6, "Recorded Prop"=w3086:T7, "Fabrication Prop"=w3084:T8)  [unwired: 8 in]
                n1744 = Unbundle By Name(w3085) -> ("Mobility-Sat"=w3098:dbl, "Moblitity-Lin"=w3099:dbl, "On/Off"=w3100:dbl, "Off Current"=w3101:dbl, "Vt-Sat"=w3077:dbl, "STS"=w3102:dbl, "Trap Density-VT"=w3103:dbl, "Trap Density-STS"=w3104:dbl)
                n1745 = Unbundle By Name(w3086) -> ("Date Recorded"=w3094:string, "Index"=w3095:string, "Length"=w3096:dbl, "Width"=w3097:dbl, "Sample Temp"=w3080:dbl)
                n1746 = Unbundle By Name(w3084) -> ("Date Created"=w3105:string, "Material"=w3087:string, "Solvent"=w3088:string, "Concentration"=w3089:dbl, "Method"=w3090:string, "Dielectric (nm)"=w3091:dbl, "Treatment"=w3092:string, "Comments"=w3093:string)
                n1747 = local write "Rec: Off I-Sat"(w3101) -> ()
                n1748 = local write "Rec: Comments"(w3093) -> ()
                n1749 = local write "Rec: VT-Sat"(w3077) -> ()
                n1750 = local write "Date Created"(w3105) -> ()
                n1751 = local write "Rec: Material"(w3087) -> ()
                n1752 = local write "Rec: Solvent"(w3088) -> ()
                n1753 = local write "Rec: Concentration"(w3089) -> ()
                n1754 = local write "Rec: Method"(w3090) -> ()
                n1755 = local write "Rec: Dielectric (d)"(w3091) -> ()
                n1756 = local write "Surface Treatment:"(w3092) -> ()
                n1757 = local write "Index"(w3095) -> ()
                n1758 = local write "Rec: Mobility-Sat"(w3098) -> ()
                n1759 = local write "Rec: Mobility-Lin"(w3099) -> ()
                n1760 = local write "Rec: On/Off"(w3100) -> ()
                n1761 = local write "Rec: STS"(w3102) -> ()
                n1762 = local write "Rec: Trap Density-VT"(w3103) -> ()
                n1763 = local write "Rec: Trap Density-STS"(w3104) -> ()
                n1764 = local write "Date Recorded"(w3094) -> ()
                n1765 = local write "Rec: Length"(w3096) -> ()
                n1766 = local write "Rec: Width"(w3097) -> ()
                n1767 = local write "Rec: Temp"(w3080) -> ()
                n1768 = Equal To 0?(x=w3080) -> (x = 0?=w3081:bool)
                n1769 = case shown="False" w3081 {
                  tunnel: [w3197 w3198] -> w3078
                  tunnel: w3080 -> [w3197 _]
                  frame False {
                  }
                  frame True {
                    n1770 = local read "Room Temp"() -> (w3198:dbl)
                  }
                }
                n1771 = local read "NumPoints Log"() -> (w3126:dbl)
                n1772 = Transpose 2D Array(2D array=w3055) -> (transposed array=w3056:ext[][])
                n1773 = local write "Transfer File"(w3083) -> ()
                n1774 = local read "Num Pts"() -> (w3115:dbl)
                n1775 = local read "Num Pts"() -> (w3127:dbl)
                n1776 = for {
                  tunnel: w3054 -> [w3195]
                  tunnel: w3056 -> [w3196] mode=indexing
                  tunnel: [w3194] -> w3052 mode=indexing
                  n1777 = Bundle(w3195, w3196) -> (w3194:cluster{ext[], ext[]})  [unwired: 1 in]
                }
                n1778 = call-poly <vilib>:"Read From Spreadsheet File.vi"("file path (dialog if empty)"=w3083) -> ("all rows"=w3173:string[][])  [unwired: 6 in, 4 out]
                n1779 = call "Mobility-Vt Calculator-File.vi"("NumPts"=w3127, "Path"=w3083) -> ("Graph Cluster"=w3074:T9, "Output"=w3128:T10, "Index-Sat"=w3108:dbl, "Index-Lin"=w3114:dbl)  [unwired: 5 in, 1 out]
                n1780 = Unbundle By Name(w3074) -> ("Raw Sat"=w3071:cluster{dbl[], dbl[]}[], "Sqrt Sat"=w3073:cluster{dbl[], dbl[]}[], "Raw Lin"=w3070:cluster{dbl[], dbl[]}[], "Sqrt Lin"=w3072:cluster{dbl[], dbl[]}[], "Log Lin"=w3069:cluster{dbl[], dbl[]}[])  [unwired: 1 out]
                n1781 = Decimate 1D Array(w3072) -> (w3122:cluster{dbl[], dbl[]}[])  [unwired: 1 out]
                n1782 = Array To Cluster(array=w3122) -> (cluster=w3120:T11)
                n1783 = Unbundle(w3120) -> ("[0]"=w3121:cluster{dbl[], dbl[]})  [unwired: 8 out]
                n1784 = Unbundle(w3121) -> (w3119:dbl[], w3118:dbl[])
                n1785 = Array Subset(array=w3118, index=w3114, length=w3115) -> (w3116:dbl[])
                n1786 = Array Subset(array=w3119, index=w3114, length=w3115) -> (w3117:dbl[])
                n1787 = call "STS Calculator-File.vi"("NumPts"=w3126, "Path"=w3083) -> ("STS Index-Sat"=w3125:dbl, "XY Graph-Sat"=w3124:cluster{dbl[], dbl[]}[], "Ouput"=w3123:cluster{"STS-Sat":dbl, "STS-Lin":dbl})  [unwired: 5 in, 2 out]
                n1788 = local write "Transport"(w3052) -> ()
                n1789 = Array Size(array=w3052) -> (size(s)=w3051:i32)
                n1790 = local read "New: Dielectric"() -> (w3110:dbl)
                n1791 = local write "Sat-Trans Slider"(w3108) -> ()
                n1792 = for {
                  N: w3051 -> [_]
                  i -> [w3193]
                  n1793 = local read "Transport Line Color"() -> (w3192:u32)
                  n1794 = local read "Ring"() -> (w3191:u16)
                  n1795 = property on="Transport" class="XYGraph (strict)"("Active Plot"=w3193, "Plot.Plot Color"=w3192, "Plot.Line Width"=w3191) -> ()  [unwired: 2 in, 2 out]
                }
                n1796 = local write "Lin Id-Used"(w3116) -> ()
                n1797 = local write "Lin-Vg Array-Used"(w3117) -> ()
                n1798 = local write "MobVi Index"(w3108) -> ()
                n1799 = local write "Index 2"(w3125) -> ()
                n1800 = local write "Sqrt-Sat"(w3073) -> ()
                n1801 = local write "Sat-Log"(w3124) -> ()
                n1802 = Unbundle By Name(w3128) -> ("Mobility-Sat"=w3113:dbl, "Vt-Sat"=w3075:dbl, "Mobility-Lin"=w3112:dbl, "Mobility-Lin"=w3111:dbl, "Off I-Sat"=w3106:dbl, "On/Off I-Sat"=w3076:dbl)
                n1803 = local write "Sqrt-Lin"(w3072) -> ()
                n1804 = Array Size(array=w3173) -> (size(s)=w3172:i32[])
                n1805 = local write "Raw- Sat"(w3071) -> ()
                n1806 = local write "New: Temp"(w3078) -> ()
                n1807 = Unbundle By Name(w3123) -> ("STS-Sat"=w3109:dbl)
                n1808 = call "Trap Density_STS.vi"("Temp (T) [K]"=w3078, "S.T.S. (S)"=w3109, "Dielectric"=w3110) -> ("Trap Density (N)"=w3082:dbl)  [unwired: 8 in]
                n1809 = local write "Calc: Mobility-Lin"(w3112) -> ()
                n1810 = local write "Raw- Lin"(w3070) -> ()
                n1811 = local write "Calc: Mobility-Sat"(w3113) -> ()
                n1812 = local write "Log-Lin"(w3069) -> ()
                n1813 = local write "Calc: Off I-Sat"(w3106) -> ()
                n1814 = local write "Calc: VT-Sat"(w3075) -> ()
                n1815 = local write "New: VT-Lin"(w3111) -> ()
                n1816 = local write "New: Trap Density-STS"(w3082) -> ()
                n1817 = local write "Calc: Trap Density-STS"(w3082) -> ()
                n1818 = local read "Image Folder"() -> (w3162:path)
                n1819 = local read "New: Dielectric"() -> (w3107:dbl)
                n1820 = Decimate 1D Array(w3073) -> (w3157:cluster{dbl[], dbl[]}[])  [unwired: 1 out]
                n1821 = Decimate 1D Array(w3124) -> (w3147:cluster{dbl[], dbl[]}[])  [unwired: 1 out]
                n1822 = Index Array(array=w3172, index=w3171) -> (element=w3153:i32)
                n1823 = Array Subset(array=w3173, index (row)=w3171, index (col)=w3171, length (col)=3) -> (w3174:string[][])  [unwired: 1 in]
                n1824 = local write "Calc: STS"(w3109) -> ()
                n1825 = local write "New: VT-Sat"(w3075) -> ()
                n1826 = local write "New: Mobility-Sat"(w3113) -> ()
                n1827 = local write "Calc: On/Off"(w3076) -> ()
                n1828 = local write "New: Mobility-Lin"(w3112) -> ()
                n1829 = List Folder(path=w3162) -> (filenames=w3167:string[])  [unwired: 3 in, 3 out]
                n1830 = local write "New: VT-Lin"(w3111) -> ()
                n1831 = Array To Cluster(array=w3157) -> (cluster=w3159:T11)
                n1832 = Array To Cluster(array=w3147) -> (cluster=w3145:T11)
                n1833 = Reshape Array(w3174, w3153) -> (w3160:string[])
                n1834 = Subtract(x=w3153, y=20) -> (x-y=w3152:i32)
                n1835 = local write "New: STS"(w3109) -> ()
                n1836 = property on="Sat-Trans Slider" class="Slide (strict)"("Scale.Maximum"=w3152) -> ()  [unwired: 2 in, 2 out]
                n1837 = call "Trap Density_VT.vi"("VT"=w3075, "Dielectric"=w3107) -> ("Trap Density-VT"=w3079:dbl)
                n1838 = Unbundle(w3159) -> ("[0]"=w3158:cluster{dbl[], dbl[]})  [unwired: 8 out]
                n1839 = Unbundle(w3145) -> ("[0]"=w3146:cluster{dbl[], dbl[]})  [unwired: 8 out]
                n1840 = Search 1D Array(1D array=w3160, element="Index:") -> (index of element=w3168:i32)  [unwired: 1 in]
                n1841 = local write "New: Trap Density-VT"(w3079) -> ()
                n1842 = local write "Calc: Trap Density-VT"(w3079) -> ()
                n1843 = Unbundle(w3158) -> (w3149:dbl[], w3148:dbl[])
                n1844 = Unbundle(w3146) -> (w3144:dbl[], w3143:dbl[])
                n1845 = Increment(x=w3168) -> (x+1=w3169:i32)
                n1846 = Array Subset(array=w3149, index=w3108, length=w3127) -> (w3156:dbl[])
                n1847 = Array Subset(array=w3148, index=w3108, length=w3127) -> (w3155:dbl[])
                n1848 = Array Subset(array=w3144, index=w3125, length=w3126) -> (w3151:dbl[])
                n1849 = Array Subset(array=w3143, index=w3125, length=w3126) -> (w3150:dbl[])
                n1850 = Index Array(array=w3160, index=w3169) -> (element=w3165:string)
                n1851 = local write "Vg Array-Log-Used"(w3150) -> ()
                n1852 = local write "Sat Id-Log-Used"(w3151) -> ()
                n1853 = local write "Sat Id-Used"(w3155) -> ()
                n1854 = local write "Index"(w3165) -> ()
                n1855 = local write "Sat Vg Array-Used"(w3156) -> ()
                n1856 = while {
                  tunnel: w3167 -> [w3206]
                  tunnel: w3165 -> [w3204]
                  tunnel: [w3203] -> _
                  tunnel: [w3203] -> w3166
                  tunnel: w3153 -> [w3202]
                  i -> [w3203]
                  stop <- w3199 stop-if-true
                  n1857 = Index Array(array=w3206, index=w3203) -> (element=w3207:string)
                  n1858 = xnode "Match Regular Expression"("input string"=w3207, "regular expression"=w3204) -> ("whole match"=w3205:string)  [unwired: 4 in, 4 out]
                  n1859 = Equal?(x=w3205, y=w3204) -> (x = y?=w3201:bool)
                  n1860 = Equal?(x=w3202, y=w3203) -> (x = y?=w3200:bool)
                  n1861 = Or(x=w3201, y=w3200) -> (x .or. y?=w3199:bool)
                }
                n1862 = Path To String(path=w3162) -> (string=w3164:string)
                n1863 = Index Array(array=w3167, index=w3166) -> (element=w3141:string)
                n1864 = local write "Image Name"(w3141) -> ()
                n1865 = Empty String/Path?(string/path=w3141) -> (empty?=w3142:bool)
                n1866 = Concatenate Strings(w3164, "\\", w3141) -> (w3163:string)
                n1867 = String To Path(string=w3163) -> (path=w3140:path)
                n1868 = local read "No Image File"() -> (w3139:path)
                n1869 = Select(t=w3139, s=w3142, f=w3140) -> (s? t:f=w3133:path)
                n1870 = local write "Image File"(w3133) -> ()
                n1871 = local read "Image Out"() -> (w3131:T2)
                n1872 = call "IMAQ ReadFile"("File Path"=w3133, "Image"=w3131) -> ("Image Out"=w3132:T2)  [unwired: 5 in, 4 out]
                n1873 = local write "Image Out"(w3132) -> ()
                n1874 = local write "Image Out 2"(w3132) -> ()
              }
              frame #4 {
                # "Output ROI data"
                n1875 = local read "Image Folder"() -> (w3322:path)
                n1876 = Build Path(base path=w3322, name or relative path="ROI") -> (appended path=w3324:path)
                n1877 = local read "Index"() -> (w3323:string)
                n1878 = Build Path(base path=w3324, name or relative path=w3323) -> (appended path=w3329:path)
                n1879 = invoke on="Image Out" class="ImageControl" method="Clear ROI"() -> (error out=w3328:errorcluster)  [unwired: 3 in, 2 out]
                n1880 = call <vilib>:"Check if File or Folder Exists.vi"("error in (no error)"=w3328, "path"=w3329) -> ("file or folder exists?"=w3326:bool, "dup path"=w3327:path)  [unwired: 7 in, 1 out]
                n1881 = case shown="True" w3326 {
                  tunnel: w3327 -> [_ w3330]
                  frame False {
                  }
                  frame True {
                    n1882 = Read from Text File(file (use dialog)=w3330) -> (text=w3334:string)  [unwired: 3 in, 3 out]
                    n1883 = property on="Image Out" class="ImageControl"() -> ("ROI"=w3331:T12)  [unwired: 2 in, 2 out]
                    n1884 = Unflatten From String(type=w3331, binary string=w3334) -> (value=w3332:T12, error out=w3333:errorcluster)  [unwired: 3 in, 1 out]
                    n1885 = property on="Image Out" class="ImageControl"(error in=w3333, "ROI"=w3332) -> ()  [unwired: 1 in, 2 out]
                  }
                }
              }
            }
            n1886 = flat-sequence {
              tunnel: [w2489] -> w2476
              tunnel: w2476 -> [w2503]
              frame #0 {
                # "Makes Empty File for Transformer Data"
                n1887 = local read "Transfer Folder"() -> (w2478:path)
                n1888 = Build Path(base path=w2478, name or relative path="Stats") -> (appended path=w2480:path)
                n1889 = call <vilib>:"Check if File or Folder Exists.vi"("path"=w2480) -> ("file or folder exists?"=w2481:bool, "dup path"=w2482:path)  [unwired: 8 in, 1 out]
                n1890 = case shown="False" w2481 {
                  tunnel: [w2486 w2488] -> w2483
                  tunnel: w2482 -> [w2487 w2488]
                  frame False {
                    n1891 = Create Folder(path (use dialog)=w2487) -> (created path=w2486:path)  [unwired: 2 in, 2 out]
                  }
                  frame True {
                  }
                }
                n1892 = Build Path(base path=w2483, name or relative path="Tranformer Data.txt") -> (appended path=w2485:path)
                n1893 = call-poly <vilib>:"Write To Spreadsheet File.vi"("append to file? (new file:F)"=TRUE, "file path (dialog if empty)"=w2485) -> ()  [unwired: 6 in, 1 out]
              }
              frame #1 {
                # "Adds Headers if they don't exist"
                n1894 = local read "Transfer Folder"() -> (w2495:path)
                n1895 = Concatenate Strings("Stats\\", "Tranformer Data.txt") -> (w2496:string)
                n1896 = Build Path(base path=w2495, name or relative path=w2496) -> (appended path=w2489:path)
                n1897 = call-poly <vilib>:"Read From Spreadsheet File.vi"("file path (dialog if empty)"=w2489) -> ("first row"=w2494:string[])  [unwired: 6 in, 4 out]
                n1898 = Search 1D Array(1D array=w2494, element="DeviceID") -> (index of element=w2492:i32)  [unwired: 1 in]
                n1899 = Equal?(x=w2492, y=0) -> (x = y?=w2490:bool)
                n1900 = case shown="False" w2490 {
                  tunnel: w2489 -> [w2500 _]
                  frame False {
                    n1901 = local read "Transformer \nHeaders"() -> (w2499:string[])
                    n1902 = call-poly <vilib>:"Write To Spreadsheet File.vi"("1D data"=w2499, "file path (dialog if empty)"=w2500) -> ()  [unwired: 6 in, 1 out]
                  }
                  frame True {
                  }
                }
              }
              frame #2 {
                # "Adds current device if it doesn't exist"
                n1903 = local read "Current \nRecord"() -> (w2506:string[])
                n1904 = Index Array(array=w2506, index=0) -> (element=w2505:string)
                n1905 = local read "Transfer Folder"() -> (w2508:path)
                n1906 = Concatenate Strings("Stats\\", "Tranformer Data.txt") -> (w2509:string)
                n1907 = local write "Current Device ID"(w2505) -> ()
                n1908 = local read "Current Device ID"() -> (w2515:string)
                n1909 = Build Path(base path=w2508, name or relative path=w2509) -> (appended path=w2507:path)
                n1910 = call-poly <vilib>:"Read From Spreadsheet File.vi"("file path (dialog if empty)"=w2507) -> ("all rows"=w2502:string[][])  [unwired: 6 in, 4 out]
                n1911 = Index Array(array=w2502, index (col)=0) -> (element=w2513:string[])  [unwired: 1 in]
                n1912 = Search 1D Array(1D array=w2513, element=w2515) -> (index of element=w2501:i32)  [unwired: 1 in]
                n1913 = Equal?(x=w2501, y=-1) -> (x = y?=w2504:bool)
                n1914 = case shown="False" w2504 {
                  tunnel: w2503 -> [w2517 w2530]
                  tunnel: w2501 -> [w2522 _]
                  tunnel: w2502 -> [w2523 _]
                  frame False {
                    n1915 = local read "Current \nRecord"() -> (w2521:string[])
                    n1916 = Replace Array Subset(array=w2523, new element=w2521, index (row)=w2522) -> (w2518:string[][])  [unwired: 1 in]
                    n1917 = flat-sequence {
                      tunnel: [w2524] -> _
                      tunnel: [w2525] -> _
                      tunnel: [w2525] -> w2520
                      tunnel: [w2524] -> w2519
                      tunnel: w2518 -> [w2525]
                      tunnel: w2517 -> [w2524]
                      tunnel: w2520 -> [w2527]
                      tunnel: w2519 -> [w2526]
                      frame #0 {
                        n1918 = Delete(path (use dialog)=w2524) -> ()  [unwired: 4 in, 3 out]
                      }
                      frame #1 {
                        n1919 = call-poly <vilib>:"Write To Spreadsheet File.vi"("append to file? (new file:F)"=TRUE, "2D data"=w2527, "file path (dialog if empty)"=w2526) -> ()  [unwired: 5 in, 1 out]
                      }
                    }
                  }
                  frame True {
                    n1920 = local read "Current \nRecord"() -> (w2529:string[])
                    n1921 = call-poly <vilib>:"Write To Spreadsheet File.vi"("append to file? (new file:F)"=TRUE, "1D data"=w2529, "file path (dialog if empty)"=w2530) -> ()  [unwired: 5 in, 1 out]
                  }
                }
              }
            }
          }
          event "Export": Mouse Down {
            n1922 = event-data() -> ()  [unwired: 1 in, 7 out]
            n1923 = flat-sequence {
              frame #0 {
                n1924 = stacked-sequence {
                  frame #0 {
                    n1925 = local read "Independant Variable"() -> (w3336:string)
                    n1926 = Equal?(x=w3336, y="Length (um):") -> (x = y?=w3337:bool)
                    n1927 = case shown="True" w3337 {
                      frame False {
                      }
                      frame True {
                        n1928 = local write "X Axis Display Type"("1") -> ()
                        n1929 = local write "Opj X Axis"("2") -> ()
                      }
                    }
                  }
                  frame #1 {
                    n1930 = local read "Independant Variable"() -> (w3341:string)
                    n1931 = Equal?(x=w3341, y="Sample Temp (K):") -> (x = y?=w3342:bool)
                    n1932 = case shown="True" w3342 {
                      frame False {
                      }
                      frame True {
                        n1933 = local write "X Axis Display Type"("1") -> ()
                        n1934 = local write "Opj X Axis"("1") -> ()
                      }
                    }
                  }
                  frame #2 {
                    n1935 = local read "Independant Variable"() -> (w3346:string)
                    n1936 = Equal?(x=w3346, y="Mobility-Sat (cm^2/Vs):") -> (x = y?=w3347:bool)
                    n1937 = case shown="True" w3347 {
                      frame False {
                      }
                      frame True {
                        n1938 = local write "X Axis Display Type"("2") -> ()
                        n1939 = local write "Opj X Axis"("2") -> ()
                      }
                    }
                  }
                  frame #3 {
                    n1940 = local read "Independant Variable"() -> (w3351:string)
                    n1941 = Equal?(x=w3351, y="Mobility-Lin (cm^2/Vs):") -> (x = y?=w3352:bool)
                    n1942 = case shown="True" w3352 {
                      frame False {
                      }
                      frame True {
                        n1943 = local write "X Axis Display Type"("2") -> ()
                        n1944 = local write "Opj X Axis"("2") -> ()
                      }
                    }
                  }
                  frame #4 {
                    n1945 = local read "Independant Variable"() -> (w3356:string)
                    n1946 = Equal?(x=w3356, y="On/Off I-Sat:") -> (x = y?=w3357:bool)
                    n1947 = case shown="True" w3357 {
                      frame False {
                      }
                      frame True {
                        n1948 = local write "X Axis Display Type"("2") -> ()
                        n1949 = local write "Opj X Axis"("2") -> ()
                      }
                    }
                  }
                  frame #5 {
                    n1950 = local read "Independant Variable"() -> (w3361:string)
                    n1951 = Equal?(x=w3361, y="Off I-Sat (A):") -> (x = y?=w3362:bool)
                    n1952 = case shown="True" w3362 {
                      frame False {
                      }
                      frame True {
                        n1953 = local write "X Axis Display Type"("2") -> ()
                        n1954 = local write "Opj X Axis"("2") -> ()
                      }
                    }
                  }
                  frame #6 {
                    n1955 = local read "Independant Variable"() -> (w3366:string)
                    n1956 = Equal?(x=w3366, y="Vt-Sat (V):") -> (x = y?=w3367:bool)
                    n1957 = case shown="True" w3367 {
                      frame False {
                      }
                      frame True {
                        n1958 = local write "X Axis Display Type"("1") -> ()
                        n1959 = local write "Opj X Axis"("1") -> ()
                      }
                    }
                  }
                  frame #7 {
                    n1960 = local read "Independant Variable"() -> (w3371:string)
                    n1961 = Equal?(x=w3371, y="STS-Sat (V/decade):") -> (x = y?=w3372:bool)
                    n1962 = case shown="True" w3372 {
                      frame False {
                      }
                      frame True {
                        n1963 = local write "X Axis Display Type"("1") -> ()
                        n1964 = local write "Opj X Axis"("1") -> ()
                      }
                    }
                  }
                  frame #8 {
                    n1965 = local read "Independant Variable"() -> (w3376:string)
                    n1966 = Equal?(x=w3376, y="Trap Density-VT (Traps/Vcm^2):") -> (x = y?=w3377:bool)
                    n1967 = case shown="True" w3377 {
                      frame False {
                      }
                      frame True {
                        n1968 = local write "X Axis Display Type"("2") -> ()
                        n1969 = local write "Opj X Axis"("2") -> ()
                      }
                    }
                  }
                  frame #9 {
                    n1970 = local read "Independant Variable"() -> (w3381:string)
                    n1971 = Equal?(x=w3381, y="Trap Density-STS (Traps/Vcm^2):") -> (x = y?=w3382:bool)
                    n1972 = case shown="True" w3382 {
                      frame False {
                      }
                      frame True {
                        n1973 = local write "X Axis Display Type"("2") -> ()
                        n1974 = local write "Opj X Axis"("2") -> ()
                      }
                    }
                  }
                }
              }
              frame #1 {
                n1975 = local read "Transfer Folder"() -> (w3390:path)
                n1976 = Build Path(base path=w3390, name or relative path="Stats") -> (appended path=w3391:path)
                n1977 = local read "Origin Project File"() -> (w3402:path)
                n1978 = call <vilib>:"Check if File or Folder Exists.vi"("path"=w3391) -> ("file or folder exists?"=w3406:bool, "dup path"=w3405:path)  [unwired: 8 in, 1 out]
                n1979 = call <userlib>:"OA_ConnectToOrigin.vi"() -> ("error out"=w3403:errorcluster, "Origin.IOApplication"=w3404:refnum<k7>)  [unwired: 8 in]
                n1980 = case shown="False" w3406 {
                  tunnel: w3405 -> [w3579 w3580]
                  tunnel: [w3578 w3580] -> w3389
                  frame False {
                    n1981 = Create Folder(path (use dialog)=w3579) -> (created path=w3578:path)  [unwired: 2 in, 2 out]
                  }
                  frame True {
                  }
                }
                n1982 = call <userlib>:"OA_Load.vi"("error in (no error)"=w3403, "Path"=w3402, "Origin.IOApplication"=w3404) -> ("error out"=w3400:errorcluster, "Origin.IOApplication"=w3401:refnum<k7>)  [unwired: 1 out]
                n1983 = call "OAExecute.vi"("script"="document -m 3;", "Error IO"=w3400, "Origin.IOApplication"=w3401) -> ("Error IO Out"=w3398:errorcluster, "Origin.IOApplication"=w3399:refnum<k7>)  [unwired: 1 in, 1 out]
                n1984 = call "File Dialog"("start path"=w3391) -> ("selected path"=w3393:path)  [unwired: 11 in, 3 out]
                n1985 = local read "Independant Variable"() -> (w3386:string)
                n1986 = stacked-sequence {
                  tunnel: w3390 -> [w3417 w3447 w3459 w3481 w3501 w3522 w3543 w3566]
                  tunnel: w3389 -> [w3418 w3446 w3460 w3480 w3502 w3523 w3544 w3567]
                  tunnel: w3399 -> [w3420 w3444 w3462 w3483 w3504 w3525 w3546 w3569]
                  tunnel: w3398 -> [w3419 w3445 w3461 w3482 w3503 w3524 w3545 w3568]
                  tunnel: [_ _ _ _ _ _ _ w3564] -> w3388
                  tunnel: [_ _ _ _ _ _ _ w3565] -> w3387
                  tunnel: w3386 -> [w3416 w3437 w3458 w3479 w3500 w3521 w3542 w3563]
                  frame #0 {
                    n1987 = local read "X Axis Display Type"() -> (w3408:string)
                    n1988 = local read "Opj X Axis"() -> (w3413:string)
                    n1989 = Concatenate Strings("window -a MOBLGraph;\nlayer.x.type=", w3413, "; layer.x.label.numFormat = ", w3408, "; Y3 = 1; X3 = 1;", "window -a MOBLTable;\nwindow -s TV;") -> (w3411:string)
                    n1990 = call "Param_Analysis_7_24b_JW.vi"("Independant Variable"=w3416, "error in (no error)"=w3419, "Data Folder"=w3417, "Parameter String"="Mobility-Lin (cm^2/Vs):", "Parameter Name"="Mobility-Lin", "Stats Folder"=w3418) -> ("error out"=w3422:errorcluster, "Output Array"=w3424:string[][], "Variables"=w3415:T18)  [unwired: 2 in, 1 out]
                    n1991 = call "Origin_Export_7_27a_JW.vi"("Input Conditions"=w3415, "Analysis Array"=w3424, "error in (no error)"=w3422, "Parameter Worksheet Name"="[MOBLTable]Mobilities", "Parameter Folder Script"="pe_cd \"Mobility-Lin\";", "Origin.IOApplication"=w3420) -> ("error out"=w3421:errorcluster, "reference out"=w3423:refnum<k7>)  [unwired: 3 in, 1 out]
                    n1992 = call "OAExecute.vi"("script"=w3411, "Error IO"=w3421, "Origin.IOApplication"=w3423) -> ()  [unwired: 1 in, 3 out]
                  }
                  frame #1 {
                    n1993 = local read "X Axis Display Type"() -> (w3429:string)
                    n1994 = local read "Opj X Axis"() -> (w3434:string)
                    n1995 = Concatenate Strings("window -a MOBSGraph;\nlayer.x.type=", w3434, "; layer.x.label.numFormat = ", w3429, "; Y3 = 1; X3 = 1;", "window -a MOBSTable;\nwindow -s TV;") -> (w3432:string)
                    n1996 = call "Param_Analysis_7_24b_JW.vi"("Independant Variable"=w3437, "error in (no error)"=w3445, "Data Folder"=w3447, "Parameter String"="Mobility-Sat (cm^2/Vs):", "Parameter Name"="Mobility-Sat", "Stats Folder"=w3446) -> ("error out"=w3440:errorcluster, "Output Array"=w3438:string[][], "Variables"=w3436:T18)  [unwired: 2 in, 1 out]
                    n1997 = call "Origin_Export_7_27a_JW.vi"("Input Conditions"=w3436, "Analysis Array"=w3438, "error in (no error)"=w3440, "Parameter Worksheet Name"="[MOBSTable]Mobilities", "Parameter Folder Script"="pe_cd \"Mobility-Sat\";", "Origin.IOApplication"=w3444) -> ("error out"=w3439:errorcluster, "reference out"=w3441:refnum<k7>)  [unwired: 3 in, 1 out]
                    n1998 = call "OAExecute.vi"("script"=w3432, "Error IO"=w3439, "Origin.IOApplication"=w3441) -> ()  [unwired: 1 in, 3 out]
                  }
                  frame #2 {
                    n1999 = local read "X Axis Display Type"() -> (w3450:string)
                    n2000 = local read "Opj X Axis"() -> (w3455:string)
                    n2001 = Concatenate Strings("window -a NSTSGraph;\nlayer.x.type=", w3455, "; layer.x.label.numFormat = ", w3450, "; Y3 = 1; X3 = 1;", "window -a NSTSTable;\nwindow -s TV;") -> (w3453:string)
                    n2002 = call "Param_Analysis_7_24b_JW.vi"("Independant Variable"=w3458, "error in (no error)"=w3461, "Data Folder"=w3459, "Parameter String"="Trap Density-STS (Traps/Vcm^2):", "Parameter Name"="Trap Density-STS", "Stats Folder"=w3460) -> ("error out"=w3465:errorcluster, "Output Array"=w3463:string[][], "Variables"=w3457:T18)  [unwired: 2 in, 1 out]
                    n2003 = call "Origin_Export_7_27a_JW.vi"("Input Conditions"=w3457, "Analysis Array"=w3463, "error in (no error)"=w3465, "Parameter Worksheet Name"="[NSTSTable]Trap Densities", "Parameter Folder Script"="pe_cd \"N-STS\";", "Origin.IOApplication"=w3462) -> ("error out"=w3464:errorcluster, "reference out"=w3466:refnum<k7>)  [unwired: 3 in, 1 out]
                    n2004 = call "OAExecute.vi"("script"=w3453, "Error IO"=w3464, "Origin.IOApplication"=w3466) -> ()  [unwired: 1 in, 3 out]
                  }
                  frame #3 {
                    n2005 = local read "X Axis Display Type"() -> (w3471:string)
                    n2006 = local read "Opj X Axis"() -> (w3476:string)
                    n2007 = call "Param_Analysis_7_24b_JW.vi"("Independant Variable"=w3479, "error in (no error)"=w3482, "Data Folder"=w3481, "Parameter String"="Trap Density-VT (Traps/Vcm^2):", "Parameter Name"="Trap Density-Vt", "Stats Folder"=w3480) -> ("error out"=w3486:errorcluster, "Output Array"=w3484:string[][], "Variables"=w3478:T18)  [unwired: 2 in, 1 out]
                    n2008 = Concatenate Strings("window -a NVtGraph;\nlayer.x.type=", w3476, "; layer.x.label.numFormat = ", w3471, "; Y3 = 1; X3 = 1;", "window -a NVtTable;\nwindow -s TV;") -> (w3474:string)
                    n2009 = call "Origin_Export_7_27a_JW.vi"("Input Conditions"=w3478, "Analysis Array"=w3484, "error in (no error)"=w3486, "Parameter Worksheet Name"="[NVTTable]Trap Densities", "Parameter Folder Script"="pe_cd \"N-Vt\";", "Origin.IOApplication"=w3483) -> ("error out"=w3485:errorcluster, "reference out"=w3487:refnum<k7>)  [unwired: 3 in, 1 out]
                    n2010 = call "OAExecute.vi"("script"=w3474, "Error IO"=w3485, "Origin.IOApplication"=w3487) -> ()  [unwired: 1 in, 3 out]
                  }
                  frame #4 {
                    n2011 = local read "X Axis Display Type"() -> (w3492:string)
                    n2012 = local read "Opj X Axis"() -> (w3497:string)
                    n2013 = Concatenate Strings("window -a OffIGraph;\nlayer.x.type=", w3497, "; layer.x.label.numFormat = ", w3492, "; Y3 = 1; X3 = 1;", "window -a OffITable;\nwindow -s TV;") -> (w3495:string)
                    n2014 = call "Param_Analysis_7_24b_JW.vi"("Independant Variable"=w3500, "error in (no error)"=w3503, "Data Folder"=w3501, "Parameter String"="Off I-Sat (A):", "Parameter Name"="Off I-Sat", "Stats Folder"=w3502) -> ("error out"=w3507:errorcluster, "Output Array"=w3505:string[][], "Variables"=w3499:T18)  [unwired: 2 in, 1 out]
                    n2015 = call "Origin_Export_7_27a_JW.vi"("Input Conditions"=w3499, "Analysis Array"=w3505, "error in (no error)"=w3507, "Parameter Worksheet Name"="[OffItable]OffCurrents", "Parameter Folder Script"="pe_cd \"OffI-Sat\";", "Origin.IOApplication"=w3504) -> ("error out"=w3506:errorcluster, "reference out"=w3508:refnum<k7>)  [unwired: 3 in, 1 out]
                    n2016 = call "OAExecute.vi"("script"=w3495, "Error IO"=w3506, "Origin.IOApplication"=w3508) -> ()  [unwired: 1 in, 3 out]
                  }
                  frame #5 {
                    n2017 = local read "X Axis Display Type"() -> (w3513:string)
                    n2018 = local read "Opj X Axis"() -> (w3518:string)
                    n2019 = Concatenate Strings("window -a OnOffGraph;\nlayer.x.type=", w3518, "; layer.x.label.numFormat = ", w3513, "; Y3 = 1; X3 = 1;", "window -a OnOffTable;\nwindow -s TV;") -> (w3516:string)
                    n2020 = call "Param_Analysis_7_24b_JW.vi"("Independant Variable"=w3521, "error in (no error)"=w3524, "Data Folder"=w3522, "Parameter String"="On/Off I-Sat:", "Parameter Name"="OnOff Ratio", "Stats Folder"=w3523) -> ("error out"=w3528:errorcluster, "Output Array"=w3526:string[][], "Variables"=w3520:T18)  [unwired: 2 in, 1 out]
                    n2021 = call "Origin_Export_7_27a_JW.vi"("Input Conditions"=w3520, "Analysis Array"=w3526, "error in (no error)"=w3528, "Parameter Worksheet Name"="[OnOffTable]On/Off Ratios", "Parameter Folder Script"="pe_cd \"OnOff-Ratio\";", "Origin.IOApplication"=w3525) -> ("error out"=w3527:errorcluster, "reference out"=w3529:refnum<k7>)  [unwired: 3 in, 1 out]
                    n2022 = call "OAExecute.vi"("script"=w3516, "Error IO"=w3527, "Origin.IOApplication"=w3529) -> ()  [unwired: 1 in, 3 out]
                  }
                  frame #6 {
                    n2023 = local read "X Axis Display Type"() -> (w3534:string)
                    n2024 = local read "Opj X Axis"() -> (w3539:string)
                    n2025 = call "Param_Analysis_7_24b_JW.vi"("Independant Variable"=w3542, "error in (no error)"=w3545, "Data Folder"=w3543, "Parameter String"="STS-Sat (V/decade):", "Parameter Name"="STS-Sat", "Stats Folder"=w3544) -> ("error out"=w3549:errorcluster, "Output Array"=w3547:string[][], "Variables"=w3541:T18)  [unwired: 2 in, 1 out]
                    n2026 = Concatenate Strings("window -a SGraph;\nlayer.x.type=", w3539, "; layer.x.label.numFormat = ", w3534, "; Y3 = 1; X3 = 1;", "window -a STable;\nwindow -s TV;") -> (w3537:string)
                    n2027 = call "Origin_Export_7_27a_JW.vi"("Input Conditions"=w3541, "Analysis Array"=w3547, "error in (no error)"=w3549, "Parameter Worksheet Name"="[STable]Threshold Swing", "Parameter Folder Script"="pe_cd \"STS-Sat\";", "Origin.IOApplication"=w3546) -> ("error out"=w3548:errorcluster, "reference out"=w3550:refnum<k7>)  [unwired: 3 in, 1 out]
                    n2028 = call "OAExecute.vi"("script"=w3537, "Error IO"=w3548, "Origin.IOApplication"=w3550) -> ()  [unwired: 1 in, 3 out]
                  }
                  frame #7 {
                    n2029 = local read "X Axis Display Type"() -> (w3555:string)
                    n2030 = local read "Opj X Axis"() -> (w3560:string)
                    n2031 = Concatenate Strings("window -a VtGraph;\nlayer.x.type=", w3560, "; layer.x.label.numFormat = ", w3555, "; Y3 = 1; X3 = 1;", "window -a VtTable;\nwindow -s TV;") -> (w3558:string)
                    n2032 = call "Param_Analysis_7_24b_JW.vi"("Independant Variable"=w3563, "error in (no error)"=w3568, "Data Folder"=w3566, "Parameter String"="Vt-Sat (V):", "Parameter Name"="Vt-Sat", "Stats Folder"=w3567) -> ("error out"=w3572:errorcluster, "Output Array"=w3570:string[][], "Variables"=w3562:T18)  [unwired: 2 in, 1 out]
                    n2033 = call "Origin_Export_7_27a_JW.vi"("Input Conditions"=w3562, "Analysis Array"=w3570, "error in (no error)"=w3572, "Parameter Worksheet Name"="[VtTable]Threshold Voltages", "Parameter Folder Script"="pe_cd \"Vt-Sat\";", "Origin.IOApplication"=w3569) -> ("error out"=w3571:errorcluster, "reference out"=w3573:refnum<k7>)  [unwired: 3 in, 1 out]
                    n2034 = call "OAExecute.vi"("script"=w3558, "Error IO"=w3571, "Origin.IOApplication"=w3573) -> ("Error IO Out"=w3564:errorcluster, "Origin.IOApplication"=w3565:refnum<k7>)  [unwired: 1 in, 1 out]
                  }
                }
                n2035 = Path To String(path=w3393) -> (string=w3392:string)
                n2036 = call "OAExecute.vi"("script"="pe_cd /; ", "Error IO"=w3388, "Origin.IOApplication"=w3387) -> ("Error IO Out"=w3394:errorcluster, "Origin.IOApplication"=w3395:refnum<k7>)  [unwired: 1 in, 1 out]
                n2037 = call <userlib>:"OASaveProject.vi"("path"=w3392, "Error IO"=w3394, "Origin.IOApplication"=w3395) -> ()  [unwired: 3 out]
              }
            }
          }
          event "Blank Button": Mouse Down {
            n2038 = event-data() -> ()  [unwired: 1 in, 7 out]
            n2039 = local read "Transfer File"() -> (w3588:path)
            n2040 = disable-structure shown="Disabled" {
              frame Disabled {
                n2041 = local read "Folder Index"() -> (w3589:dbl)
                n2042 = Decrement(x=w3589) -> (x-1=w3590:dbl)
                n2043 = local write "Folder Index"(w3590) -> ()
              }
              frame Enabled {
              }
            }
            n2044 = Strip Path(path=w3588) -> (stripped path=w3584:path, name=w3586:string)
            n2045 = Path To String(path=w3584) -> (string=w3583:string)
            n2046 = Concatenate Strings(w3583, "\\", "X_", w3586) -> (w3582:string)
            n2047 = String To Path(string=w3582) -> (path=w3581:path)
            n2048 = Move(source path=w3588, 10:w3581) -> ()  [unwired: 3 in, 3 out]
            n2049 = local write "Transfer File"(w3581) -> ()
          }
          event "Cancel Button": Mouse Down {
            (unwired) 6
            n2050 = event-data() -> ()  [unwired: 1 in, 7 out]
            n2051 = call "Simulate_Keyboard.vi"("Action"=2, "Virtual Key"=162) -> ()  [unwired: 7 in, 1 out]
          }
        }
        n2052 = Multiply(x=w468, y=10) -> (x*y=w470:sgl)
        n2053 = case shown="\"0\"" w509 {
          tunnel: w483 -> [w648 w654 w658 w660 w664 w666 w668 w670 w672 w674 w676 w678 w680 w682 w684 w686 w688 w690 w692 w694 w696 w698 w700 w702 w704 w706 w708 w710 w712 w714 w716 w718 w720 w722 w724 w726 w728 w730 w732 w734 w736 w738 w740 w742 w744 w746 w748 w750 w752 w754 w756 w758 w760 w762 w764 w766 w768 w770 w772 w774 w776 w778 w780 w782 w784 w786 w788 w790 w792 w794 w796 w798 w800 w802 w804 w806 w808 w810 w812 w814 w816 w818 w820 w822 w824 w826 w828 w830 w832 w834 w836 w838 w840 w842 w844 w846 w848 w850 w852 w854 w856 w858 w860 w862 w864]
          tunnel: [w648 w653 w657 w660 w664 w666 w668 w670 w672 w674 w676 w678 w680 w682 w684 w686 w688 w690 w692 w694 w696 w698 w700 w702 w704 w706 w708 w710 w712 w714 w716 w718 w720 w722 w724 w726 w728 w730 w732 w734 w736 w738 w740 w742 w744 w746 w748 w750 w752 w754 w756 w758 w760 w762 w764 w766 w768 w770 w772 w774 w776 w778 w780 w782 w784 w786 w788 w790 w792 w794 w796 w798 w800 w802 w804 w806 w808 w810 w812 w814 w816 w818 w820 w822 w824 w826 w828 w830 w832 w834 w836 w838 w840 w842 w844 w846 w848 w850 w852 w854 w856 w858 w860 w862 w864] -> w508
          tunnel: w484 -> [w650 w652 w656 w662 w663 w665 w667 w669 w671 w673 w675 w677 w679 w681 w683 w685 w687 w689 w691 w693 w695 w697 w699 w701 w703 w705 w707 w709 w711 w713 w715 w717 w719 w721 w723 w725 w727 w729 w731 w733 w735 w737 w739 w741 w743 w745 w747 w749 w751 w753 w755 w757 w759 w761 w763 w765 w767 w769 w771 w773 w775 w777 w779 w781 w783 w785 w787 w789 w791 w793 w795 w797 w799 w801 w803 w805 w807 w809 w811 w813 w815 w817 w819 w821 w823 w825 w827 w829 w831 w833 w835 w837 w839 w841 w843 w845 w847 w849 w851 w853 w855 w857 w859 w861 w863]
          tunnel: [w649 w652 w656 w661 w663 w665 w667 w669 w671 w673 w675 w677 w679 w681 w683 w685 w687 w689 w691 w693 w695 w697 w699 w701 w703 w705 w707 w709 w711 w713 w715 w717 w719 w721 w723 w725 w727 w729 w731 w733 w735 w737 w739 w741 w743 w745 w747 w749 w751 w753 w755 w757 w759 w761 w763 w765 w767 w769 w771 w773 w775 w777 w779 w781 w783 w785 w787 w789 w791 w793 w795 w797 w799 w801 w803 w805 w807 w809 w811 w813 w815 w817 w819 w821 w823 w825 w827 w829 w831 w833 w835 w837 w839 w841 w843 w845 w847 w849 w851 w853 w855 w857 w859 w861 w863] -> w507
          tunnel: w470 -> [w647 w651 w655 w659 _ _ _ _ _ _ _ _ _ _ _ _ _ _ _ _ _ _ _ _ _ _ _ _ _ _ _ _ _ _ _ _ _ _ _ _ _ _ _ _ _ _ _ _ _ _ _ _ _ _ _ _ _ _ _ _ _ _ _ _ _ _ _ _ _ _ _ _ _ _ _ _ _ _ _ _ _ _ _ _ _ _ _ _ _ _ _ _ _ _ _ _ _ _ _ _ _ _ _ _ _]
          frame "DOWN" {
            n2054 = Add(x=w650, y=w647) -> (x+y=w649:sgl)
          }
          frame "LEFT" {
            n2055 = Subtract(x=w654, y=w651) -> (x-y=w653:sgl)
          }
          frame "RIGHT" {
            n2056 = Add(x=w658, y=w655) -> (x+y=w657:sgl)
          }
          frame "UP" {
            n2057 = Subtract(x=w662, y=w659) -> (x-y=w661:sgl)
          }
          frame "ENTER (num pad)" {
          }
          frame "' (quote)" {
          }
          frame "END" {
          }
          frame "EQUALS" {
          }
          frame "ESCAPE" {
          }
          frame "GRAVE (`)" {
          }
          frame "HOME" {
          }
          frame "INSERT" {
          }
          frame "LBRACKET" {
          }
          frame "LCONTROL" {
          }
          frame "L ALT" {
          }
          frame "LSHIFT" {
          }
          frame "LWIN" {
          }
          frame "MINUS" {
          }
          frame "MULTIPLY" {
          }
          frame "NEXT" {
          }
          frame "NUMLOCK" {
          }
          frame "NUMPAD_0" {
          }
          frame "NUMPAD_1" {
          }
          frame "NUMPAD_2" {
          }
          frame "NUMPAD_3" {
          }
          frame "NUMPAD_4" {
          }
          frame "NUMPAD_5" {
          }
          frame "NUMPAD_6" {
          }
          frame "NUMPAD_7" {
          }
          frame "NUMPAD_8" {
          }
          frame "NUMPAD_9" {
          }
          frame "PAUSE" {
          }
          frame "PERIOD" {
          }
          frame "PRIOR (PG UP)" {
          }
          frame "RBRACKET" {
          }
          frame "RCONTROL" {
          }
          frame "RETURN" {
          }
          frame "R ALT" {
          }
          frame "RSHIFT" {
          }
          frame "RWIN" {
          }
          frame "SCROLL" {
          }
          frame "SEMICOLON" {
          }
          frame "SLASH" {
          }
          frame "SPACE" {
          }
          frame "SUBTRACT" {
          }
          frame "TAB" {
          }
          frame "DIVIDE" {
          }
          frame "DELETE" {
          }
          frame "DECIMAL" {
          }
          frame "COMMA" {
          }
          frame "CAPITAL" {
          }
          frame "BACKSLASH" {
          }
          frame "BACK" {
          }
          frame "ADD" {
          }
          frame "F15" {
          }
          frame "F14" {
          }
          frame "F13" {
          }
          frame "F12" {
          }
          frame "F11" {
          }
          frame "F10" {
          }
          frame "F9" {
          }
          frame "F8" {
          }
          frame "F7" {
          }
          frame "F6" {
          }
          frame "F5" {
          }
          frame "F4" {
          }
          frame "F3" {
          }
          frame "F2" {
          }
          frame "F1" {
          }
          frame "Z" {
          }
          frame "Y" {
          }
          frame "X" {
          }
          frame "W" {
          }
          frame "V" {
          }
          frame "U" {
          }
          frame "T" {
          }
          frame "S" {
          }
          frame "R" {
          }
          frame "Q" {
          }
          frame "P" {
          }
          frame "O" {
          }
          frame "N" {
          }
          frame "M" {
          }
          frame "L" {
          }
          frame "K" {
          }
          frame "J" {
          }
          frame "I" {
          }
          frame "H" {
          }
          frame "G" {
          }
          frame "F" {
          }
          frame "E" {
          }
          frame "D" {
          }
          frame "C" {
          }
          frame "B" {
          }
          frame "A" {
          }
          frame "9" {
          }
          frame "8" {
          }
          frame "7" {
          }
          frame "6" {
          }
          frame "5" {
          }
          frame "4" {
          }
          frame "3" {
          }
          frame "2" {
          }
          frame "1" {
          }
          frame "0" {
          }
        }
        n2058 = Bundle(w486, w485, w500, w499, 0.0) -> (w498:cluster{dbl, dbl, dbl, dbl, dbl})  [unwired: 1 in]
        n2059 = Bundle("X"=w508, "Y"=w507) -> (w502:cluster{"X":sgl, "Y":sgl})  [unwired: 1 in]
        n2060 = Divide(x=20, y=w469) -> (x/y=w472:sgl)
        n2061 = property on="Image Out" class="ImageControl"("Image Center Position"=w502) -> ()  [unwired: 2 in, 2 out]
        n2062 = call "IMAQ Convert Rectangle to ROI (Polygon)"("Rectangle"=w498) -> ("ROI Descriptor"=w496:T4)  [unwired: 7 in, 2 out]
        n2063 = Bundle("Application Font", w472, w476, w476, w476, w476, w476, TRUE, w474) -> (w478:T19)  [unwired: 1 in]
        n2064 = property on="Image Out 2" class="ImageControl"("ROI"=w496) -> ()  [unwired: 2 in, 2 out]
        n2065 = Bundle(w474, w478, w474, w474) -> (w477:T20)  [unwired: 1 in]
        n2066 = property on="Image Out" class="ImageControl"() -> ("ROI"=w461:T12)  [unwired: 2 in, 2 out]
        n2067 = Unbundle By Name(w461) -> ("Contours"=w525:T16)
        n2068 = local read "Image Out"() -> (w480:T2)
        n2069 = call "IMAQ Clear Overlay"("Image"=w480) -> ("Image Out"=w479:T2)  [unwired: 9 in, 1 out]
        n2070 = Initialize Array(0) -> (w523:i32[])  [unwired: 1 in]
        n2071 = local read "Magnification"() -> (w514:u16)
        n2072 = Array Size(array=w525) -> (size(s)=w524:i32)
        n2073 = Build Array(0.505025, 0.252522, 0.127742, 0.050345, 0.031129) -> (w515:dbl[])
        n2074 = Array Subset(array=w515, index=w514, length=1) -> (w512:dbl[])
        n2075 = property on="Image Out" class="ImageControl"() -> ("ZoomInteger"=w504:cluster{"X":i32, "Y":i32})  [unwired: 2 in, 2 out]
        n2076 = To Double Precision Float(number=w512) -> (double precision float=w511:dbl[])
        n2077 = for {
          N: w524 -> [_]
          shift-right: [w887] -> _
          shift-left: w525 -> [w887]
          shift-right: [w885] -> w510
          shift-left: w523 -> [w884]
          tunnel: w511 -> [w883]
          shift-right: [w880] -> _
          shift-left: w479 -> [w882]
          tunnel: w477 -> [w875]
          i -> [w879]
          n2078 = Index Array(array=w887, index=w879) -> (element=w896:T21)
          n2079 = Unbundle(w896) -> ("Points"=w895:i32[])  [unwired: 2 out]
          n2080 = Array To Cluster(array=w895) -> (cluster=w894:T22)
          n2081 = Unbundle(w894) -> ("Points[0]"=w874:i32, "Points[1]"=w871:i32, "Points[2]"=w886:i32, "Points[3]"=w892:i32)  [unwired: 5 out]
          n2082 = Add(x=w874, y=10) -> (x+y=w872:i32)
          n2083 = Subtract(x=w871, y=w892) -> (x-y=w891:i32)
          n2084 = Subtract(x=w874, y=w886) -> (x-y=w893:i32)
          n2085 = Square(x=w891) -> (x^2=w889:i32)
          n2086 = Square(x=w893) -> (x^2=w890:i32)
          n2087 = Add(x=w890, y=w889) -> (x+y=w888:i32)
          n2088 = Square Root(x=w888) -> (sqrt(x)=w865:dbl)
          n2089 = Multiply(x=w865, y=0.5) -> (x*y=w868:dbl)
          n2090 = Add(x=w868, y=w871) -> (x+y=w870:dbl)
          n2091 = Bundle(w872, w870) -> (w881:cluster{i32, dbl})  [unwired: 1 in]
          n2092 = Multiply(x=w865, y=w883) -> (x*y=w878:dbl[])
          n2093 = Index Array(array=w878) -> (element=w877:dbl)  [unwired: 1 in]
          n2094 = Number To Fractional String(number=w877) -> (F-format string=w876:string)  [unwired: 3 in]
          n2095 = call "IMAQ Overlay Text"("BG Color (Transparent)"=u32 0, "Text Color (black)"=u32 16448250, "Font, Size & Style"=w875, "String"=w876, "Origin"=w881, "Image"=w882) -> ("Image Out"=w880:T2)  [unwired: 4 in, 1 out]
          n2096 = Build Array (concatenate)(w884, w878) -> (w885:dbl[])
          n2097 = local write "Numeric 3"(w865) -> ()
        }
        n2098 = local write "ROI Descriptor"(w461) -> ()
        n2099 = Unbundle(w504) -> ("X"=w503:i32)  [unwired: 1 out]
        n2100 = Add Array Elements(numeric array=w510) -> (sum=w521:dbl)
        n2101 = local write "Distances"(w510) -> ()
        n2102 = local write "Total Width"(w521) -> ()
        n2103 = local write "Zoom"(w503) -> ()
        n2104 = local read "Manual-Width"() -> (w427:bool)
        n2105 = local read "Total Width"() -> (w464:dbl)
        n2106 = local read "Rec: Width"() -> (w462:dbl)
        n2107 = case shown="False" w427 {
          frame False {
            n2108 = property on="New: Width" class="DigNum (strict)"("DisabledEnum"=1) -> ()  [unwired: 2 in, 2 out]
          }
          frame True {
            n2109 = property on="New: Width" class="DigNum (strict)"("DisabledEnum"=0) -> ()  [unwired: 2 in, 2 out]
          }
        }
        n2110 = Not(x=w427) -> (.not. x?=w459:bool)
        n2111 = Equal To 0?(x=w464) -> (x = 0?=w460:bool)
        n2112 = Or(x=w460, y=w427) -> (x .or. y?=w463:bool)
        n2113 = And(x=w460, y=w459) -> (x .and. y?=w458:bool)
        n2114 = case shown="True" w458 {
          tunnel: w462 -> [_ w623]
          frame False {
          }
          frame True {
            n2115 = local write "New: Width"(w623) -> ()
          }
        }
        n2116 = case shown="False" w463 {
          tunnel: w464 -> [w625 _]
          frame False {
            n2117 = local write "New: Width"(w625) -> ()
            n2118 = property on="New: Width" class="DigNum (strict)"("DisabledEnum"=1) -> ()  [unwired: 2 in, 2 out]
          }
          frame True {
            n2119 = property on="New: Width" class="DigNum (strict)"("DisabledEnum"=0) -> ()  [unwired: 2 in, 2 out]
          }
        }
        n2120 = local read "Manual Comments"() -> (w428:bool)
        n2121 = local read "Rec: Comments"() -> (w429:string)
        n2122 = local read "Manuel-Dielectric"() -> (w455:bool)
        n2123 = local read "Rec: Dielectric (d)"() -> (w454:dbl)
        n2124 = local read "Manuel-Length"() -> (w456:bool)
        n2125 = local read "Rec: Length"() -> (w457:dbl)
        n2126 = case shown="True" w428 {
          tunnel: w429 -> [w606 _]
          frame False {
            n2127 = local write "Comments:"(w606) -> ()
            n2128 = property on="Comments:" class="Str"("DisabledEnum"=1) -> ()  [unwired: 2 in, 2 out]
          }
          frame True {
            n2129 = property on="Comments:" class="Str"("DisabledEnum"=0) -> ()  [unwired: 2 in, 2 out]
          }
        }
        n2130 = case shown="True" w456 {
          tunnel: w457 -> [w621 _]
          frame False {
            n2131 = local write "New: Length"(w621) -> ()
            n2132 = property on="New: Length" class="DigNum (strict)"("DisabledEnum"=1) -> ()  [unwired: 2 in, 2 out]
          }
          frame True {
            n2133 = property on="New: Length" class="DigNum (strict)"("DisabledEnum"=0) -> ()  [unwired: 2 in, 2 out]
          }
        }
        n2134 = case shown="True" w455 {
          tunnel: w454 -> [w618 _]
          frame False {
            n2135 = local write "New: Dielectric"(w618) -> ()
            n2136 = property on="New: Dielectric" class="DigNum (strict)"("DisabledEnum"=1) -> ()  [unwired: 2 in, 2 out]
          }
          frame True {
            n2137 = property on="New: Dielectric" class="DigNum (strict)"("DisabledEnum"=0) -> ()  [unwired: 2 in, 2 out]
          }
        }
      }
    }
  }
  n2138 = disable-structure shown="Disabled" {
    frame Disabled {
      # "Transformer Work"
      n2139 = Build Array("DeviceID", "Fabricator", "Deposition", "Date", "Sample", "Row", "Column", "L (um)", "W (um)", "Material", "Treatment", "TC (mM)", "Solvent", "C (%)", "ST (C)", "Drops", "Wait (s)", "RT (F)", "RH (%)", "Ramp (s)", "RPM", "Accel (RPM/s)", "Time (s)", "Mobility", "On/Off", "Vt", "S.T.S") -> (→"Transformer \nHeaders":string[])
    }
    frame Enabled {
    }
  }
